vi "OxygenExtractor_elife34.vi"(14 "Image_array":T3[](array[typedef])=["IMAGE0", "Image1"]) -> (19 "Local error":errorcluster caption="error in")   [LabVIEW 2013]
uses:
  <vilib>/vision/Image Controls.llb/IMAQ Image.ctl
  <vilib>/Analysis/baseanly.llb/Mean (DBL).vi
  <vilib>/Analysis/NI_AALBase.lvlib
  Phosphorescence - Mode.lvlib
  <vilib>/vision/NI_Vision_Development_Module.lvlib
  <vilib>/Analysis/NI_AALPro.lvlib
panel:
  out "Acquisition Time":timestamp=timestamp(-9593251200 s since 1904-01-01)
  in  "Point Number":i32
  in  "Save":bool
  in  "Time onglets":enum32{"Averaged", "Time-lapsed"}(tab)
  out "Average fit":dbl[][](graph)
  out "DataValues":T1(array[cluster])
  in  "Analyse Average":bool
  in  "Pulse Amplitu Analysis":enum32{"RBC Flow", "EAT", "pO2 RBC/InterRBC"}(tab)=enum."pO2 RBC/InterRBC"
  in  "Channel Analysed RBC Flow":u16(ring)=1 items=["1", "2"]
  out "RBC anal Checked":dbl[][](graph)
  out "Mean Flow":dbl format="%#_3g"
  out "Mean Hematocrit":dbl format="%#_3g"
  in  "Analyse RBCs Flow":bool
  in  "from time (s)":dbl
  in  "to time (s)":dbl max=9.984
  in  "Point Analysed":i32 max=600
  in  "Analyse EAT":bool
  in  "Channel analysed for EAT":u16(ring) items=["1", "2"]
  in  "Around RBCs Analysis":enum32{"Tau", "Po2", "Number of decays"}(tab)=enum."Number of decays"
  out "Tau / RBCs":cluster{dbl[], dbl[]}(graph) caption="Measurement"
  out "PO2 / RBCs":cluster{dbl[], dbl[]}(graph) caption="Measurement"
  out "Decays / RBCs":cluster{dbl[], i32[]}(graph) caption="Measurement"
  out "Point EAT":i32 max=600
  in  "RBC before":bool
  in  "RBC after":bool
  in  "Analyse PO2 RBC/InterRBC":bool
  out "Std pO2 (1)":dbl format="%#_3g"
  out "pO2 (1)":dbl format="%#_3g"
  out "Std pO2 (2)":dbl format="%#_3g"
  out "pO2 (2)":dbl format="%#_3g"
  out "Std Tau 1":dbl format="%#_3g"
  out "Amplitude 1":dbl format="%#_3g"
  out "Std Tau 2":dbl format="%#_3g"
  out "Amplitude 2":dbl format="%#_3g"
  out "Number of decays 2":i32
  out "Number of decays 1":i32
  out "Tau 2 (us)":dbl format="%#_3g"
  out "Tau 1 (us)":dbl format="%#_3g"
  out "Average fit 1/2":dbl[][](graph)
  in  "From time (ms) 1":dbl=-1.0 min=-10.7328
  in  "To time (ms) 1":dbl=1.0 max=38.1888
  in  "From time (ms) 2":dbl=8.0 min=-10.7328
  in  "To time (ms) 2":dbl=12.0 max=38.1888
  in  "Min":dbl=-3.0 format="%#.1f"
  in  "Max":dbl=20.0 format="%#.1f"
  in  "Channel Analysed":u16(ring) items=["1", "2"]
  out "Total number of points":i32=1
  in  "LUT":u16(ring)=7 items=["grey-progress", "gray", "gray + high", "gray + bounds", "gradient", "temperature", "cold/hot (1/2)", "cold/hot (1/4)", "odd/even"]
  in  "Display raw Data":bool=TRUE
  out "Standard error Tau (us)":dbl format="%#_3g"
  out "element 2":dbl
  out "element":dbl
  out "Tau (us)":dbl format="%#_3g"
  out "Area (au)":dbl format="%#_3g"
  out "amplitude":dbl caption="Amplitude (au)" format="%#_3g"
  out "size(s) 3":i32[](array[numeric])=[2, 40000]
  out "size(s) 2":i32[](array[numeric])=[4, 267]
  out "size(s)":i32[](array[numeric])=[8, 267]
  in  "Time":dbl[](array[numeric])
  in  "Tau":dbl[](array[numeric])
  in  "Po2":dbl[](array[numeric])
  in  "Decays":i32[](array[numeric])=[0, 0, 0, 0, 0, 0, 0, 0, 0, 0, 0, 0, 0, 0, 0, 0, 0, 0, 0, 0, 0, 0, 0, 0, 0, 0, 0, 0, 0, 0, 0, 0, 0, 0, 0, 0, 0, 0, 0, 0, 0, 0, 0, 0, 0, 0, 0, 0, 0, 0, 0, 0, 0, 0, 0, 0, 0, 0, 0, 0, 0, 0, 0, 0, 0, 0, 0, 0, 0, 0, 0, 0, 0, 0, 0, 0, 0, 0, 0, 0, 0, 0, 0, 0, 0, 0, 0, 0, 0, 0, 0, 0, 0, 0, 0, 0, 0, 0, 0, 0, 0, 0, 0, 0, 0, 0, 0, 0, 0, 0, 0, 0, 0, 0, 0, 0, 0, 0, 0, 0, 0, 0, 0, 0, 0, 0, 0, 0, 0, 0, 0, 0, 0, 0, 0, 0, 0, 0, 0, 0, 0, 0, 0, 0, 0, 0, 0, 0, 0, 0, 0, 0, 0, 0, 0, 0, 0, 0, 0, 0, 0, 0, 0, 0, 0, 0, 0, 0, 0, 0, 0, 0, 0, 0, 0, 0, 0, 0, 0, 0, 0, 0, 0, 0, 0, 0, 0, 0, 0, 0, 0, 0, 0, 0, 0, 0, 0, 0, 0, 0, 0, 0, 0, 0, 0, 0, 0, 0, 0, 0, 0, 0, 0, 0, 0, 0, 0, 0, 0, 0, 0, 0, 0, 0, 0]
  out "Decays Max":i32=20000
  out "BA":bool
  out "RBC_before":i32[](array[numeric])
  out "RBC_after":i32[](array[numeric])
  out "Cells detect":u8[](array[numeric])
  out "Average fit 2":dbl[][](graph)=[[234.9197268868795, 232.23934305222366, 229.69994463923234, 227.888171249308, 226.6098911238236, 223.73740542535523, 221.40745525004613, 219.90182690533308, 217.30485329396566, 217.11736482745894, 216.68702712677614, 215.40763978593836, 215.2103709171434, 214.11810297102787, 212.40228824506366, 210.0345082118472, 208.90514855139324, 208.88060527772652, 208.52112935966045, 207.90090422587193, 207.060712308544, 206.41409854216644, 207.19985237128623, 206.4203727625023, 204.68186012179368, 203.77246724487912, 202.63627975641262, 201.80531463369624, 201.31887802177525, 201.88134342129544, 201.80715999261855, 201.11422771729102, 200.49898505259273, 199.00756597158147, 197.83299501753092, 198.52112935966045, 199.2378667650858, 198.64772098173094, 198.0005536076767, 197.43329027495847, 197.48902011441226, 197.4725964200037, 197.0042443255213, 197.83078058682415, 197.77966414467613, 198.14965860859937, 198.19154825613583, 197.06551024174203, 196.30872854770251, 195.9422402657317, 195.32349141908102, 196.50433659346743, 196.7776342498616, 196.0428123269976, 196.01107215353386, 196.26960693854954, 195.3941686658055, 194.80162391585162, 194.9665990035062, 195.37386971766009, 195.15630190071968, 194.81823214615244, 194.5357076951467, 193.93854954788708, 193.71858276434767, 193.5956818601218, 194.29027495847942, 194.8739619856062, 194.54456541797379, 194.27495847942424, 194.0310020298948, 193.6194869902196, 193.30540690164236, 192.56966229931723, 192.14965860859937, 193.18988743310575, 193.57446023251524, 193.7158147259642, 193.98523712862152, 194.10075659715815, 193.94777634249863, 193.32884295995572, 193.38125115334933, 193.38734083779295, 193.57556744786862, 193.61192101863813, 193.41169957556744, 192.5100572061266, 192.1064772098173, 192.0363535707695, 191.87027126776158, 192.7449713969367, 193.06809374423327, 192.66248385310942, 192.8745155932829, 192.62059420557298, 192.75770437350064, 192.75899612474626, 192.55729839453772, 193.15925447499538, 193.2967337147075, 193.37479239712124, 193.3400996493818, 192.9815464107769, 192.63388078981362, 192.15501014947407, 192.01974534046872, 192.24801623915852, 192.51577781878575, 192.4493448975826, 192.21184720428124, 192.29839453773758, 192.13452666543643, 192.4899427938734, 192.4096696807529, 192.51097988558774, 192.4880974349511, 192.27514301531647, 192.53607676693116, 192.73150027680384, 192.39084701974534, 192.19265547148922, 192.27440487174755, 192.38678723011625, 192.49086547333457, 192.3098357630559, 192.0819339361506, 191.84406717106478, 191.68794980623733, 191.9007196899797, 192.50931906255767, 192.63332718213692, 192.58184166820448, 192.7067724672449, 192.61985606200406, 191.94390108876178, 192.1225318324414, 191.83262594574646, 191.80697545672632, 192.260380143938, 192.4270160546226, 192.17457095405055, 191.94611551946855, 191.8180476102602, 191.9922494925263, 191.99372577966415, 191.9245248200775, 192.31241926554713, 192.28510795349695, 192.29507289167742, 192.155748293043, 191.37183982284554, 191.57316848126962, 191.7805868241373, 191.67023436058312, 192.65731684812695, 192.9660453958295, 192.74589407639786, 192.6015870086732, 192.0226979147444, 191.5517623177708, 191.25004613397306, 191.38125115334933, 191.8900166082303, 192.3965676324045, 192.22144307067725, 191.96272374976934, 191.21147813249678, 191.03598449898504, 191.27385126407086, 191.3098357630559, 191.8317032662853, 192.10131020483485, 192.72393430522237, 193.18693485883003, 192.75456726333272, 192.1961616534416, 192.45137479239713, 192.3436058313342, 192.58294888355786, 192.28289352279018, 192.12862151688503, 192.365011994833, 191.81472596420005, 191.3781140431814, 191.20760287875993, 191.21369256320355, 191.57981177338993, 191.9007196899797, 192.23399151134896, 192.3393615058129, 192.0219597711755, 191.6170880236206, 191.19468536630376, 191.197268868795, 191.3513563388079, 191.62391585163314, 191.79590330319246, 192.00073814356892, 191.77929507289167, 192.0658793135265, 192.2967337147075, 192.2199667835394, 192.44952943347482, 192.5238973980439, 192.2502306698653, 192.15740911607307, 191.81195792581656, 191.43513563388078, 191.23731315740912, 191.18305960509318, 191.61431998523713, 192.27016054622624, 192.17401734637386, 192.09909577412807, 191.96438457279942, 192.07215353386235, 191.81306514116997, 191.51743864181583, 191.63775604355047, 191.8167558590146, 191.86934858830043, 192.27606569477763, 191.9911422771729, 191.9119763794058, 191.67613950913452, 191.75179922494925, 192.06329581103526, 192.0856246539952, 192.32939656763241, 192.3816202251338, 191.96622993172173, 191.66340653257058, 191.47093559697362, 191.5458571692194, 191.7211662668389, 191.88503413914006, 192.316294519284, 192.32607492157226, 191.97342683151874, 191.92710832256873, 191.8597527219044, 191.78150950359844, 192.44270160546228, 192.78759918804207, 192.5065510241742, 192.47536445838716, 192.19173279202806, 192.2384203727625, 192.50212216276066, 192.82026204096698, 192.72282708986899, 192.4179737959033, 192.07233806975458, 192.0219597711755, 191.6997601033401, 191.66377560435504, 191.5322015131943, 191.57852002214432, 191.4043181398782, 191.9815464107769, 192.11016792766193, 192.05572983945376, 191.9719505443809, 192.1956080457649, 191.72208894630006, 191.44860675401367], [231.0665661286319, 229.30635283621848, 227.6254158206747, 226.02018464647355, 224.4872496829386, 223.02335486193417, 221.62539076173397, 220.29038800237745, 219.01551093848562, 217.79805163613858, 216.63542412102234, 215.5251588856263, 214.46489764382545, 213.4523883217047, 212.485480273986, 211.5621197158976, 210.68034536078187, 209.83828425417641, 209.0341477955191, 208.26622793902712, 207.53289356568047, 206.8325870186035, 206.1638207944857, 205.5251743840136, 204.91529125460332, 204.33287596902403, 203.77669143379282, 203.24555627149593, 202.738342311455, 202.2539721934085, 201.7914170791181, 201.34969446703982, 200.92786610541722, 200.52503599936492, 200.1403485077085, 199.7729865255391, 199.42216974862143, 199.0871530159696, 198.7672247270695, 198.46170533038642, 198.16994587994668, 197.89132665692833, 197.62525585333185, 197.3711683149361, 197.1285243408685, 196.89680853724016, 196.67552872241083, 196.46421488155846, 196.2624181683326, 196.06970995147137, 195.88568090435666, 195.70994013557393, 195.5421143586296, 195.38184709906278, 195.22879793726705, 195.0826417854136, 194.9430681969407, 194.8097807071418, 194.6824962034527, 194.560944324099, 194.4448668838279, 194.33401732550323, 194.22816019639978, 194.12707064808416, 194.03053395882003, 193.93834507748304, 193.85030818801692, 193.76623629350578, 193.68595081897848, 193.6092812321022, 193.53606468095913, 193.4661456481366, 193.3993756203968, 193.33561277322343, 193.27472166957583, 193.21657297221077, 193.16104316896028, 193.1080143103828, 193.05737375922962, 193.00901395119513, 192.962832166442, 192.91873031141688, 192.87661471049202, 192.83639590699156, 192.79798847317875, 192.76131082880104, 192.7262850678077, 192.69283679287133, 192.66089495736253, 192.6303917144416, 192.6012622729467, 192.57344475977263, 192.54688008844772, 192.52151183362983, 192.49728611125462, 192.47415146408187, 192.45205875239643, 192.43096104963172, 192.41081354269434, 192.3915734367777, 192.37319986446252, 192.35565379891156, 192.33889797097362, 192.32289679002108, 192.30761626835277, 192.29302394900162, 192.2790888367935, 192.2657813325113, 192.2530731700239, 192.24093735624686, 192.22934811380705, 192.21828082628957, 192.20771198595077, 192.19761914378586, 192.18798086184574, 192.17877666770107, 192.16998701095739, 192.16159322172848, 192.15357747098037, 192.1459227326609, 192.13861274753523, 192.1316319886501, 192.12496562835318, 192.1185995067983, 192.11252010186868, 192.1067145004551, 192.10117037102734, 192.09587593744124, 192.09081995392515, 192.0859916811932, 192.0813808636342, 192.0769777075279, 192.0727728602425, 192.06875739036897, 192.06492276874994, 192.0612608503632, 192.05776385702111, 192.0544243608492, 192.0512352685086, 192.04818980612947, 192.04528150492268, 192.0425041874397, 192.0398519544511, 192.03731917241635, 192.03490046151757, 192.0325906842325, 192.03038493442205, 192.02827852690916, 192.02626698752726, 192.02434604361676, 192.0225116149496, 192.0207598050625, 192.0190868929807, 192.01748932531424, 192.0159637087103, 192.01450680264549, 192.0131155125427, 192.01178688319806, 192.0105180925038, 192.00930644545386, 192.00814936841965, 192.00704440368324, 192.0059892042172, 192.00498152869918, 192.00401923675125, 192.0031002843936, 192.00222271970296, 192.00138467866643, 192.00058438122238, 191.99982012747947, 191.99909029410568, 191.99839333088056, 191.9977277574023, 191.99709215994312, 191.99648518844674, 191.99590555366038, 191.9953520243966, 191.99482342491794, 191.99431863243973, 191.9938365747451, 191.99337622790756, 191.99293661411613, 191.99251679959835, 191.9921158926369, 191.99173304167545, 191.99136743351008, 191.99101829156177, 191.990684874227, 191.99036647330246, 191.9900624124809, 191.98977204591446, 191.9894947568429, 191.98922995628354, 191.9889770817803, 191.98873559620884, 191.9885049866358, 191.9882847632293, 191.9880744582184, 191.98787362489952, 191.98768183668778, 191.98749868621073, 191.98732378444305, 191.98715675988038, 191.98699725775012, 191.9868449392578, 191.98669948086763, 191.98656057361512, 191.98642792245093, 191.9863012456141, 191.9861802740336, 191.9860647507567, 191.98595443040344, 191.98584907864512, 191.98574847170676, 191.9856523958917, 191.98556064712778, 191.9854730305338, 191.9853893600055, 191.98530945782056, 191.9852331542607, 191.9851602872515, 191.98509070201797, 191.9850242507559, 191.9849607923179, 191.98490019191348, 191.98484232082285, 191.9847870561235, 191.98473428042914, 191.9846838816402, 191.98463575270594, 191.98458979139687, 191.9845459000878, 191.98450398555028, 191.9844639587547, 191.9844257346812, 191.98438923213894, 191.98435437359387, 191.98432108500378, 191.98428929566126, 191.98425893804338, 191.98422994766827, 191.98420226295823, 191.98417582510885, 191.98415057796421, 191.98412646789745, 191.98410344369702, 191.9840814564578, 191.98406045947723, 191.98404040815618, 191.98402125990413, 191.98400297404876, 191.9839855117496, 191.9839688359154, 191.9839529111254, 191.98393770355423, 191.98392318089984, 191.983909312315, 191.98389606834186, 191.98388342084922, 191.98387134297283, 191.9838598090584, 191.98384879460704, 191.98383827622322, 191.98382823156513, 191.98381863929714, 191.9838094790446, 191.9838007313504], [236.6262185575532, 233.9168654267263, 231.36638716432952, 229.46511580591297, 228.15291172316577, 225.1913434645764, 222.78412271875396, 221.28731431960676, 218.61083027480655, 218.4686786585376, 218.04278191224296, 216.7151395278533, 216.50897751453505, 215.3766704202868, 213.57554136949977, 211.14940322093548, 209.99719303386448, 210.0026506034353, 209.65871406989817, 208.9722796281753, 208.08140571853608, 207.42169950673673, 208.27859090179476, 207.48003577290848, 205.6633865926187, 204.714343472552, 203.5470226995514, 202.67316481630306, 202.13477026192092, 202.77149163417295, 202.71059837215444, 201.95886807614508, 201.3224431923964, 199.77566249561448, 198.53191792742783, 199.2718649691466, 200.04232982514614, 199.40944527949063, 198.7032124682996, 198.12294829909882, 198.20004100442614, 198.20164503633788, 197.72141526161138, 198.5664660081357, 198.4960658223256, 198.8706788474995, 198.92534620366226, 197.74133892340302, 196.9423412470641, 196.58368168961104, 195.95449446246917, 197.21293843230475, 197.46421057179646, 196.65068380980603, 196.61716211822178, 196.9666860652067, 196.03944833327645, 195.4070417087573, 195.58770501118283, 195.98679385779226, 195.7430317492035, 195.38010784654531, 195.0896810578094, 194.4745984760779, 194.24584194489236, 194.10329643363303, 194.8645426022806, 195.48250800147278, 195.08363970634107, 194.79025625878498, 194.52155670437855, 194.09555287606295, 193.7986510633217, 193.0230994106797, 192.55827756553458, 193.67237972143687, 194.09113056832376, 194.2298868891572, 194.5093647013314, 194.65130906315983, 194.500986700652, 193.8390888732644, 193.91375562916883, 193.85239193516128, 194.05818345116845, 194.11564853481707, 193.87029649680906, 192.90838211656845, 192.48369076245245, 192.43347797668966, 192.26937235389326, 193.20909811622698, 193.55501707016458, 193.0818327938614, 193.3359588247288, 193.05102906711207, 193.2131130414731, 193.23498868084442, 192.97796078019388, 193.65707566112286, 193.77857565296242, 193.85075714213136, 193.7998935606442, 193.43763246474737, 193.07961300342564, 192.56219183817635, 192.40633279090167, 192.6557438838756, 192.96071009630424, 192.86983910754813, 192.58301392879702, 192.72232358976467, 192.5595673864358, 193.00006456350965, 192.89204828674644, 192.93840517203012, 192.90402668025402, 192.63741074357856, 192.9385288472247, 193.20201268039784, 192.83285036062748, 192.59345863020565, 192.7271801062424, 192.8126726936899, 192.90265293592046, 192.67833997628793, 192.42829987286413, 192.2236253043258, 192.0937337569141, 192.30684116453853, 192.97396366647777, 193.06864318325276, 192.97281981247735, 193.10112316735726, 193.00150675502326, 192.2868161956913, 192.53651681843158, 192.21110834954814, 192.19789461552094, 192.6675655045845, 192.83061819483606, 192.5382261153347, 192.2753559061272, 192.20670037833304, 192.43223413199865, 192.4034868780543, 192.33986236167632, 192.74258616835172, 192.6998860444645, 192.66604012162742, 192.55039798558857, 191.69009516182422, 191.92995142463693, 192.1879409395458, 192.0533872121068, 193.11174204267104, 193.4428734205042, 193.16702597052407, 192.98498282268358, 192.3760662825357, 191.89777504970516, 191.56539752125886, 191.7357966323987, 192.26174640072034, 192.79962937096, 192.6154466160675, 192.34773994434124, 191.51676105471378, 191.3334189201643, 191.6425762166577, 191.6891998544663, 192.21471819155488, 192.49829513682275, 193.1637195763447, 193.70628868324854, 193.2388024397523, 192.62168783580142, 192.91511572695617, 192.81157867410158, 193.0209730150035, 192.66409605257547, 192.48505188099244, 192.76945573631676, 192.19076637487535, 191.72190873129034, 191.53737907418176, 191.54632702124437, 191.90606790289795, 192.26808206211322, 192.61122094039158, 192.71358177360997, 192.39200510031483, 191.97307514421945, 191.52313611446277, 191.5558725885915, 191.67719264542183, 191.95903819098956, 192.1351316877156, 192.3616659128391, 192.17074063700505, 192.51001674289498, 192.7717659802508, 192.67823520189958, 192.86976441736704, 192.95685272466903, 192.66701880863178, 192.5388443468772, 192.17184083272565, 191.76728998519033, 191.55221298231538, 191.5002306077201, 191.9531942097333, 192.66416098950762, 192.58783326886504, 192.47539843107737, 192.35136043633761, 192.5586917415031, 192.2631972316567, 191.88557045378099, 191.95385767343785, 192.18437938020332, 192.26573741924986, 192.76795285706407, 192.42167268350977, 192.32242755628437, 192.04017071981698, 192.12847053094276, 192.4220511126696, 192.4307031345332, 192.70072410054323, 192.77835860919137, 192.36913601693948, 192.04266950261172, 191.80830163873244, 191.93012556558148, 192.11456068010742, 192.24636990050462, 192.6982147146858, 192.69319231684014, 192.34285608143048, 192.31761436012863, 192.2612560681386, 192.1535080166765, 192.86668481388574, 193.22866685964823, 192.887897136364, 192.86523274660993, 192.61969988551502, 192.65385825095495, 192.94155403582377, 193.2984858331657, 193.14578092683539, 192.76939168761237, 192.3936108524359, 192.3449598119352, 192.05564839660448, 192.02945811365035, 191.8840108132697, 191.98358052340132, 191.74178232915372, 192.35865110104183, 192.47754849779463, 192.40509391824074, 192.35126153405633, 192.62770728609317, 192.12215677962152, 191.81696029193262], [233.2132352162058, 230.56182067772102, 228.03350211413516, 226.311226692703, 225.0668705244814, 222.28346738613408, 220.0307877813383, 218.5163394910594, 215.99887631312478, 215.76605099638027, 215.33127234130933, 214.10014004402342, 213.91176431975174, 212.85953552176892, 211.22903512062754, 208.9196132027589, 207.813104068922, 207.75855995201772, 207.38354464942273, 206.82952882356855, 206.04001889855192, 205.40649757759616, 206.1211138407777, 205.3607097520961, 203.70033365096864, 202.83059101720625, 201.72553681327383, 200.93746445108943, 200.50298578162958, 200.99119520841793, 200.90372161308267, 200.26958735843695, 199.67552691278905, 198.23946944754846, 197.134072107634, 197.7703937501743, 198.43340370502548, 197.88599668397126, 197.2978947470538, 196.7436322508181, 196.77799922439837, 196.74354780366951, 196.28707338943124, 197.0950951655126, 197.06326246702668, 197.42863836969923, 197.4577503086094, 196.38968156008104, 195.67511584834094, 195.30079884185236, 194.69248837569288, 195.7957347546301, 196.09105792792673, 195.43494084418916, 195.40498218884593, 195.5725278118924, 194.74888899833454, 194.19620612294594, 194.34549299582955, 194.7609455775279, 194.56957205223586, 194.25635644575956, 193.981734332484, 193.40250061969627, 193.19132358380298, 193.08806728661057, 193.71600731467822, 194.26541596973962, 194.0054911296065, 193.7596607000635, 193.54044735541106, 193.14342110437624, 192.81216273996301, 192.11622518795477, 191.74103965166415, 192.70739514477464, 193.0577898967067, 193.20174256277122, 193.46110955591163, 193.55020413115648, 193.39456598434526, 192.81859704664706, 192.84874667752982, 192.92228974042462, 193.0929514445688, 193.1081935024592, 192.95310265432582, 192.11173229568473, 191.72926365718217, 191.63922916484935, 191.4711701816299, 192.28084467764643, 192.58117041830195, 192.24313491235745, 192.41307236183698, 192.1901593440339, 192.3022957055282, 192.2830035686481, 192.13663600888157, 192.6614332888679, 192.81489177645258, 192.89882765211112, 192.88030573811943, 192.52546035680643, 192.1881485762016, 191.74782846077179, 191.63315789003576, 191.84028859444143, 192.07084554126726, 192.02885068761705, 191.84068047976547, 191.8744654857105, 191.70948594443706, 191.97982102423717, 191.92729107475935, 192.08355459914537, 192.07216818964818, 191.9128752870544, 192.13362468663763, 192.26098787320984, 191.9488436788632, 191.7918523127728, 191.8216296372527, 191.9609017665426, 192.07907801074867, 191.94133154982387, 191.73556799943705, 191.46450903780377, 191.28216585556055, 191.49459821542087, 192.04467445863756, 192.1980111810211, 192.1908635239316, 192.31242176713252, 192.23820536898486, 191.60098598183225, 191.70854684645124, 191.45414354194477, 191.4160562979317, 191.85319478329149, 192.02341391440916, 191.8109157927664, 191.6168751328099, 191.42939484218738, 191.55226485305394, 191.58396468127398, 191.50918727847866, 191.88225236274255, 191.8703298625294, 191.92410566172742, 191.7610986004974, 191.05358448386687, 191.2163855379023, 191.37323270872878, 191.28708150905945, 192.20289165358287, 192.48921737115478, 192.32476218227166, 192.2181911946628, 191.66932954695312, 191.20574958583643, 190.93469474668726, 191.02670567429996, 191.51828681574025, 191.993505893849, 191.82743952528702, 191.57770755519743, 190.90619521027978, 190.7385500778058, 190.90512631148403, 190.9304716716455, 191.44868834101572, 191.70432527284694, 192.28414903410004, 192.6675810344115, 192.27033208691313, 191.7706354710818, 191.9876338578381, 191.87563298856682, 192.14492475211222, 191.90169099300488, 191.77219115277762, 191.96056825334924, 191.43868555352475, 191.03431935507245, 190.8778266833381, 190.88105810516274, 191.25355564388192, 191.53335731784617, 191.85676208230635, 191.9651412380158, 191.65191444203614, 191.26110090302174, 190.86623461814474, 190.83866514899847, 191.02552003219398, 191.28879351227673, 191.4566749186693, 191.63981037429875, 191.3878495087783, 191.621741884158, 191.8217014491642, 191.76169836517923, 192.0292944495826, 192.0909420714188, 191.8334425310988, 191.77597388526894, 191.45207501890746, 191.10298128257122, 190.92241333250286, 190.86588860246624, 191.27544576074095, 191.87616010294485, 191.76020142388268, 191.72279311717878, 191.57740870926122, 191.58561532622159, 191.36293305068324, 191.14930682985067, 191.32165441366308, 191.44913233782586, 191.472959757351, 191.78417853249118, 191.56061187083606, 191.5015252025272, 191.31210829845205, 191.37512791895574, 191.7045405094009, 191.74054617345723, 191.9580690347216, 191.9848818410762, 191.56332384650398, 191.28414356252944, 191.1335695552148, 191.16158877285733, 191.3277718535704, 191.5236983777755, 191.93437432388222, 191.95895752630437, 191.603997581607, 191.53660228500883, 191.45824937567022, 191.40951099052037, 192.0187183970388, 192.3465315164359, 192.1252049119844, 192.0854961701644, 191.7637656985411, 191.82298249457006, 192.06269028969754, 192.34203824876826, 192.2998732529026, 192.06655590419422, 191.75106528707326, 191.69895973041577, 191.34387181007574, 191.29809309505973, 191.18039221311892, 191.17345952088732, 191.06685395060268, 191.60444172051197, 191.74278735752924, 191.70636576066678, 191.59263955470544, 191.76350880543666, 191.3220211129786, 191.08025321609472]]
  out "Average fit  3":dbl[][](graph)=[[361.98715164676076, 357.74737604053564, 349.9804560260586, 339.81722765110385, 333.22982265653275, 327.76076728193993, 324.60712993123417, 319.78954035468695, 314.35522982265655, 309.4455302207745, 302.92001447701773, 299.2213174086138, 297.1279406442273, 293.2345276872964, 288.36138255519364, 284.0752804922186, 277.904632645675, 272.4963807455664, 268.9420919290626, 268.5562794064423, 265.80528411147304, 263.0919290626131, 261.20285921100253, 257.7978646398842, 254.13011219688744, 251.06170828809266, 248.2643865363735, 247.28447339847992, 245.47828447339847, 242.92001447701773, 240.62269272529858, 240.8581252262034, 239.92327180600796, 236.69905899384727, 233.0515743756786, 232.7178791169019, 233.18005790807095, 232.46073108939558, 231.76239594643502, 229.27723488961274, 226.4196525515744, 225.17643865363735, 223.99077090119437, 223.76981541802388, 224.55899384726746, 222.7792254795512, 221.2839305103149, 219.96000723850887, 219.96833152370613, 219.2757871878393, 216.91639522258416, 216.61871154542163, 216.4361201592472, 215.30365544697793, 213.71226927252985, 212.47828447339847, 211.58161418747738, 211.16322837495477, 210.09428157799493, 209.7529858849077, 209.29044516829532, 209.3346000723851, 208.7547955121245, 209.28736880202678, 208.22909880564603, 207.3825551936301, 205.70774520448788, 205.89268910604414, 205.5019905899385, 205.28646398841838, 205.2082880926529, 204.88545059717697, 203.99764748461817, 203.07908070937387, 203.4011943539631, 203.5910242490047, 203.22891784292435, 203.17734346724575, 203.31270358306188, 203.44064422728917, 202.24068041983352, 200.93213897937025, 199.82446615997105, 199.93376764386537, 199.7801302931596, 199.94553022077451, 200.42309084328627, 200.57148027506335, 199.97140788997467, 199.16847629388346, 198.45258776692, 198.62486427795875, 199.06623235613463, 198.66865725660514, 198.60351067680057, 198.60712993123417, 197.88128845457837, 197.78935939196526, 197.2616720955483, 197.10495837857403, 197.3108939558451, 197.18349619978284, 197.04524068041982, 196.42870068765833, 197.34183858125226, 197.97792254795513, 197.55971769815417, 197.13789359391964, 196.14513210278682, 195.66757148027506, 195.06279406442272, 195.01791530944627, 195.40047050307638, 195.40047050307638, 195.3720593557727, 195.30094100615273, 196.22566051393412, 196.6138255519363, 197.31921824104234, 195.9719507781397, 195.18946796959827, 194.83586681143683, 194.39974665218966, 194.0988056460369, 193.8373145132103, 194.3291711907347, 195.00941006152732, 194.63282663771264, 194.20629750271445, 194.52497285559176, 194.73163228374955, 196.42580528411148, 196.24212812160695, 195.60369163952225, 195.0866811436844, 194.33568584871517, 194.0640608034745, 193.89721317408615, 193.7303655446978, 193.44064422728917, 193.24665218964893, 193.36789721317407, 193.8346000723851, 193.57582338038364, 193.87423090843285, 193.61165399927614, 193.44607310893957, 194.20810712993122, 194.1838581252262, 193.5727470141151, 193.30962721679333, 193.1026058631922, 192.7915309446254, 192.9011943539631, 192.95674990951863, 193.45747376040535, 194.13264567499095, 194.50723850886718, 194.41838581252262, 193.50506695620703, 193.0743756786102, 193.21679334057185, 192.85088671733624, 192.98117987694536, 192.91820484980093, 193.347629388346, 193.76492942453854, 193.11093014838943, 192.55211726384366, 191.89902280130292, 191.50941006152732, 191.94100615273254, 191.8177705392689, 192.33260948244663, 192.76746290264205, 192.8460007238509, 192.40589938472675, 192.27687296416937, 192.43901556279405, 192.81505609844373, 193.07419471588852, 193.256786102063, 193.0893955845096, 192.28610206297503, 192.07853782120884, 192.0106768005791, 191.62540716612378, 192.10622511762577, 192.5727470141151, 193.05772710821572, 193.17625769091566, 192.5358306188925, 192.01719145855952, 192.1550850524792, 191.9902280130293, 192.3916033297141, 192.50470503076366, 192.9605501266739, 193.20557365182773, 192.90408975750995, 192.3564965617083, 192.066594281578, 191.96905537459284, 192.9632645674991, 193.2328990228013, 193.1539992761491, 193.00162866449512, 192.49149475208108, 192.17752442996743, 191.97068403908796, 191.8563155989866, 192.23977560622512, 192.85486789721318, 193.24846181686573, 193.08070937386898, 192.89359391965255, 192.55573651827723, 191.95204487875498, 191.83116178067317, 192.54578356858488, 192.9167571480275, 192.9534925805284, 192.54759319580165, 192.37893593919654, 192.0088671733623, 191.67734346724575, 191.38472674629026, 191.661961635903, 191.9254433586681, 192.3836409699602, 192.71425986246834, 192.42978646398842, 192.44245385450597, 192.1521896489323, 191.4755700325733, 191.8816503800217, 192.1900108577633, 192.49077090119437, 192.35251538183135, 192.28356858487152, 191.91929062613102, 191.49258052841114, 191.51972493666304, 192.19525877669201, 192.1628664495114, 192.14603691639522, 192.17046688382194, 192.2495475931958, 192.17625769091566, 192.05066956207023, 192.07238508867172, 192.352696344553, 192.40463264567498, 192.50253347810352, 192.8845457835686, 192.92309084328627, 192.17788635541078, 192.01501990589938, 192.4835323923272, 193.14332247557005, 192.74068041983352, 192.4545783568585, 192.5901194353963, 192.371335504886, 191.93811074918565, 191.90644227289178, 191.65924719507782], [350.75705096081435, 345.0654666784949, 339.5784851222621, 334.2887511738493, 329.18917411891886, 324.2729181421932, 319.5333931642692, 314.9642460078337, 310.5593518814381, 306.31280616941694, 302.2189165169451, 298.2721951996231, 294.46735176736337, 290.79928595271565, 287.2630808341264, 283.85399624496745, 280.56746241949816, 277.39907386724497, 274.3445834675865, 271.39989677662777, 268.56106653873314, 265.82428739535976, 263.1858907840998, 260.64234002109316, 258.1902255602191, 255.82626042271187, 253.5472757910737, 251.35021676137936, 249.2321382482778, 247.19020103720223, 245.22166797849627, 243.32390031835507, 241.49435416166247, 239.73057706198333, 238.03020473413983, 236.39095788496488, 234.8106391579847, 233.28713018793468, 231.8183887611605, 230.4024460780978, 229.03740411416123, 227.721433075505, 226.45276894624422, 225.2297111238498, 224.05062013954665, 222.91391546065978, 221.8180733719621, 220.7616249331845, 219.7431540099495, 218.76129537548996, 217.81473288060727, 216.90219768941682, 216.02246657851518, 215.17436029728935, 214.3567419871701, 213.56851565771052, 212.80862471744683, 212.07605055757233, 211.36981118652574, 210.6889599136638, 210.03258408025377, 209.3998038360842, 208.78977096005482, 208.20166772316406, 207.6347057923701, 207.0881251738565, 206.56119319428538, 206.053203518673, 205.56347520357093, 205.09135178428375, 204.63620039489965, 204.19741091995462, 203.77439517659272, 203.3665861261262, 202.97343711393893, 202.59442113671378, 202.229030136002, 201.87677431718774, 201.53718149293428, 201.20979645023255, 200.894180340203, 200.58991008983324, 200.29657783486243, 200.01379037305273, 199.7411686371147, 199.47834718657992, 199.22497371794017, 198.98070859239618, 198.74522438058293, 198.51820542366139, 198.29934741018815, 198.08835696819617, 197.88495127193903, 197.68885766277248, 197.49981328366445, 197.31756472684393, 197.14186769411603, 196.97248666938845, 196.80919460296974, 196.65177260721686, 196.50000966312328, 196.35370233745513, 196.21265451005556, 196.07667711095203, 195.94558786691445, 195.8192110571237, 195.69737727762376, 195.5799232142413, 195.4666914236683, 195.35753012241454, 195.2522929833469, 195.15083893954252, 195.05303199519327, 194.95874104330787, 194.8678396899673, 194.78020608489786, 194.69572275813485, 194.61427646255814, 194.5357580220878, 194.46006218533756, 194.38708748452845, 194.3167360994747, 194.24891372645908, 194.18352945182176, 194.12049563009356, 194.05972776651018, 194.00114440374955, 193.94466701274118, 193.8902198874004, 193.8377300431469, 193.78712711907122, 193.73834328361835, 193.69131314366177, 193.64597365684605, 193.6022640470807, 193.56012572307174, 193.5195021997821, 193.48033902271524, 193.44258369492067, 193.40618560662355, 193.37109596738398, 193.33726774069484, 193.3046555809312, 193.27321577256575, 193.24290617156964, 193.2136861489199, 193.18551653613736, 193.1583595727829, 193.1321788558405, 193.10693929092037, 193.0826070452161, 193.05914950215274, 193.03653521766557, 193.01473387805018, 192.993716259328, 192.97345418807262, 192.95392050364404, 192.93508902178095, 192.9169344995014, 192.8994326012655, 192.88255986635446, 192.8662936774222, 192.85061223017757, 192.83549450415643, 192.82092023454442, 192.80686988501253, 192.79332462152948, 192.78026628711515, 192.76767737750185, 192.7555410176704, 192.74384093922973, 192.73256145860955, 192.72168745603716, 192.7112043552699, 192.701098104056, 192.6913551552982, 192.6819624488942, 192.67290739423012, 192.66417785330302, 192.65576212445046, 192.6476489266648, 192.63982738447132, 192.63228701334998, 192.6250177056814, 192.61800971719776, 192.61125365392107, 192.60474045957076, 192.59846140342407, 192.5924080686128, 192.58657234084077, 192.5809463975069, 192.5755226972192, 192.5702939696859, 192.56525320596975, 192.5603936490928, 192.55570878497895, 192.55119233372193, 192.54683824116745, 192.54264067079768, 192.5385939959076, 192.53469279206269, 192.53093182982752, 192.52730606775592, 192.52381064563312, 192.52044087796077, 192.51719224767618, 192.51406040009726, 192.51104113708544, 192.5081304114179, 192.50532432136274, 192.50261910544847, 192.50001113742218, 192.49749692138852, 192.49507308712361, 192.49273638555738, 192.49048368441822, 192.48831196403438, 192.48621831328614, 192.4841999257035, 192.48225409570438, 192.48037821496763, 192.47856976893684, 192.4768263334496, 192.475145571488, 192.47352523004594, 192.471963137109, 192.47045719874296, 192.46900539628706, 192.4676057836478, 192.46625648469052, 192.4649556907243, 192.4637016580777, 192.46249270576118, 192.4613272132139, 192.4602036181315, 192.45912041437168, 192.45807614993547, 192.45706942502073, 192.45609889014585, 192.45516324434075, 192.454261233403, 192.4533916482166, 192.45255332313124, 192.45174513439972, 192.45096599867162, 192.45021487154116, 192.4494907461471, 192.44879265182317, 192.4481196527969, 192.44747084693523, 192.44684536453528, 192.44624236715842, 192.44566104650653, 192.44510062333842, 192.44456034642525, 192.44403949154358, 192.4435373605046, 192.44305328021812, 192.4425866017905, 192.44213669965467, 192.44170297073157, 192.44128483362184, 192.44088172782648, 192.44049311299543, 192.44011846820328, 192.439757291251, 192.43940909799278], [365.25570048647614, 360.9663185287028, 353.1168188169238, 342.80036533045757, 336.15022351613686, 330.63089566292956, 327.4778222209384, 322.6706033882907, 317.1528636098707, 312.21577067293975, 305.6181598375633, 301.88915296850456, 299.7438890811282, 295.81082213317205, 290.8625686002171, 286.5097095691867, 280.21951425160745, 274.74874032103213, 271.1291203250122, 270.77254842490163, 268.007196364775, 265.2248507650524, 263.2885604886723, 259.85028033659023, 256.14573976352807, 253.0154184556474, 250.1789879764434, 249.20641141731264, 247.36450433863592, 244.78458999965915, 242.42001085406397, 242.71027749594745, 241.73428301643256, 238.4056901916552, 234.66130424142887, 234.33496478409245, 234.866310165342, 234.1518046791831, 233.38799380555704, 230.81439764410095, 227.8806360951708, 226.63731916607878, 225.44219412347707, 225.1972440809539, 226.04204753459226, 224.24640916369358, 222.6777639131533, 221.32791210243698, 221.35664558029754, 220.6769468200448, 218.22691267711716, 217.89249835635127, 217.71227072175017, 216.57516531500963, 214.92777148557138, 213.7023562508207, 212.7641707332041, 212.36348166830666, 211.25962412270658, 210.87697472983314, 210.4096231156084, 210.4523063916633, 209.84067777182509, 210.43425025224832, 209.34373592391154, 208.43813681330226, 206.73114952285852, 206.93572729896462, 206.51530943523562, 206.26495433341225, 206.2102675420696, 205.88237156179878, 204.962485376975, 203.97265077962686, 204.32338943088251, 204.55547110906448, 204.13334228726367, 204.09561836348593, 204.21225938247156, 204.41224122026244, 203.1506991774739, 201.7723437231445, 200.61331593156902, 200.72879514120459, 200.56028230612537, 200.73707921605174, 201.28109132539097, 201.43682617224212, 200.81900806034346, 199.94427329907975, 199.18143630964315, 199.34842835757675, 199.83879118286657, 199.4069939942787, 199.35942257908906, 199.38443832065994, 198.65724985541203, 198.59844695481172, 197.99621125447538, 197.77279857841202, 198.00458281787013, 197.87228054027526, 197.73044901117427, 197.09110511878183, 198.0902869935195, 198.78383866886884, 198.30190492027313, 197.82199814427568, 196.7485055525714, 196.25753505207874, 195.58164360682846, 195.5972086456585, 196.02296413646957, 196.03654051152543, 196.00603174467705, 195.89981116788834, 196.92116374047302, 197.3619054361548, 198.08817628653028, 196.63691323091277, 195.7532544357004, 195.3985124823186, 194.93101683542727, 194.59328793212205, 194.31015174328294, 194.84492720958698, 195.6100782884604, 195.23056450494715, 194.74532639668277, 195.1057467683169, 195.3369080625557, 197.15162285037871, 196.96620676005725, 196.2161508769852, 195.6473191194192, 194.88013180717752, 194.5894246425438, 194.4292466416272, 194.27492655298255, 193.92890573001222, 193.66006115355995, 193.79762782519794, 194.3114999475609, 194.07041922008648, 194.4209471618432, 194.14337601669712, 193.93500208147066, 194.7655581070133, 194.71310349669426, 194.03890769663695, 193.7357644656997, 193.539331370242, 193.22325580910336, 193.38665754173903, 193.4755755132856, 193.93876008345958, 194.6744958036813, 195.07288158255466, 194.97493561692835, 193.98770737103484, 193.5574805482085, 193.74124179988897, 193.3278915153728, 193.4226488139067, 193.32907452362184, 193.79798678784238, 194.28823130304207, 193.6022797957139, 193.00122125875484, 192.29900100293384, 191.85669157542844, 192.32416858620286, 192.1399293956919, 192.72368791366182, 193.2035220179836, 193.31899587615004, 192.87690800006376, 192.7010624912482, 192.9369584537053, 193.33011590194096, 193.57022226981778, 193.73134277308566, 193.52473404408175, 192.64458189166066, 192.4351828844709, 192.42987405962523, 191.994103716551, 192.48034796861896, 192.98019221769152, 193.53626887197356, 193.66044733056816, 192.97795741340556, 192.403528576285, 192.60778159712524, 192.41617718442674, 192.80196919313602, 192.93596024546457, 193.42940345950853, 193.6738394589513, 193.3699704441271, 192.76715379919517, 192.45494287502288, 192.3507863473849, 193.45098181599795, 193.71523543508346, 193.60212216941034, 193.39678441709418, 192.88531416990034, 192.56164306814932, 192.35987941863158, 192.24534857936146, 192.63729906984597, 193.3066929159672, 193.76142834615214, 193.55715806817912, 193.34959791154495, 192.9798591055439, 192.31038992192066, 192.19138195235107, 192.96633594701427, 193.36737982289037, 193.4229157770797, 192.94968157155427, 192.81637163212196, 192.423755088423, 192.05073712984833, 191.73183938370002, 192.01706244477162, 192.28222674034433, 192.77114536129224, 193.1550400998317, 192.8519792906563, 192.874824401097, 192.58607738983903, 191.81923325909324, 192.22729744952747, 192.5821635678914, 192.91650981031688, 192.73306528363287, 192.67249383504273, 192.31178462772624, 191.84832531114282, 191.89232684442578, 192.62039618664386, 192.55702882310072, 192.52634070620832, 192.55277715238435, 192.66775697972045, 192.6114863292112, 192.4599899503847, 192.5068110085425, 192.78701379815723, 192.8150056380759, 192.91290248941928, 193.3010912441786, 193.4034118717372, 192.59216864780015, 192.43270969132632, 192.9747909566735, 193.63108829884337, 193.17298469670257, 192.8214244802668, 192.98547443077652, 192.78245724116846, 192.31170130125676, 192.29825363067582, 192.0460791027105], [358.7186028070454, 354.5284335523685, 346.84409323519344, 336.83408997175013, 330.30942179692863, 324.8906389009503, 321.73643764152996, 316.9084773210832, 311.55759603544243, 306.6752897686093, 300.22186911647213, 296.55348184872304, 294.5119922073264, 290.65823324142076, 285.86019651017017, 281.6408514152505, 275.58975103974257, 270.24402117010067, 266.755063533113, 266.34001038798294, 263.6033718581711, 260.95900736017376, 259.11715793333275, 255.74544894317822, 252.1144846302468, 249.10799812053793, 246.3497850963036, 245.3625353796472, 243.59206460816102, 241.0554389543763, 238.82537459653318, 239.00597295645937, 238.11226059558336, 234.99242779603935, 231.44184450992833, 231.10079344971138, 231.4938056507999, 230.76965749960806, 230.136798087313, 227.74007213512454, 224.958669007978, 223.7155581411959, 222.53934767891167, 222.34238675509386, 223.07594015994266, 221.31204179540882, 219.89009710747646, 218.59210237458075, 218.58001746711471, 217.87462755563382, 215.60587776805116, 215.344924734492, 215.15996959674422, 214.03214557894623, 212.49676705948832, 211.25421269597624, 210.39905764175066, 209.96297508160288, 208.92893903328329, 208.62899703998227, 208.17126722098223, 208.21689375310686, 207.66891325242392, 208.14048735180523, 207.11446168738053, 206.32697357395796, 204.68434088611724, 204.84965091312367, 204.48867174464135, 204.3079736434245, 204.2063086432362, 203.88852963255516, 203.03280959226134, 202.18551063912088, 202.47899927704367, 202.62657738894492, 202.32449339858502, 202.25906857100557, 202.4131477836522, 202.4690472343159, 201.33066166219314, 200.091934235596, 199.03561638837309, 199.13874014652615, 198.99997828019383, 199.1539812254973, 199.56509036118157, 199.70613437788458, 199.12380771960588, 198.39267928868716, 197.72373922419686, 197.90130019834075, 198.2936735294027, 197.93032051893158, 197.84759877451208, 197.8298215418084, 197.1053270537447, 196.9802718291188, 196.52713293662123, 196.43711817873603, 196.61720509382008, 196.49471185929042, 196.36003234966537, 195.76629625653484, 196.59339016898502, 197.17200642704142, 196.81753047603522, 196.4537890435636, 195.54175865300223, 195.07760790847138, 194.54394452201697, 194.43862197323404, 194.7779768696832, 194.76440049462732, 194.73808696686837, 194.7020708444171, 195.5301572873952, 195.86574566771776, 196.5502601955544, 195.30698832536663, 194.62568150349614, 194.27322114055505, 193.86847646895205, 193.60432335995176, 193.36447728313763, 193.81341517188244, 194.40874183459425, 194.03508877047813, 193.66726860874613, 193.94419894286662, 194.1263565049434, 195.69998771784424, 195.51804948315666, 194.9912324020593, 194.52604316794958, 193.79123989025283, 193.53869696440518, 193.3651797065451, 193.18580453641306, 192.95238272456612, 192.8332432257379, 192.93816660115021, 193.35770019720928, 193.0812275406808, 193.3275146550225, 193.07993198185517, 192.9571441364085, 193.65065615284914, 193.65461275375816, 193.10658633159323, 192.88348996788696, 192.6658803561424, 192.35980608014745, 192.41573116618716, 192.43792430575166, 192.97618743735111, 193.5907955463006, 193.9415954351797, 193.86183600811688, 193.02242654137922, 192.59127080901192, 192.69234488125474, 192.37388191929966, 192.53971093998402, 192.50733517598002, 192.89727198884964, 193.241627546035, 192.61958050106495, 192.10301326893247, 191.499044599672, 191.1621285476262, 191.55784371926222, 191.49561168284592, 191.94153105123144, 192.3314037873005, 192.37300557155174, 191.93489076938974, 191.85268343709055, 191.9410726718828, 192.2999962949465, 192.57816716195927, 192.78222943104032, 192.65405712493742, 191.9276222342894, 191.7218927579468, 191.59147954153295, 191.25671061569656, 191.73210226663258, 192.16530181053866, 192.57918534445787, 192.69206805126316, 192.09370382437945, 191.63085434083405, 191.70238850783315, 191.56427884163188, 191.98123746629216, 192.07344981606275, 192.49169679383925, 192.73730784470416, 192.4382090708928, 191.94583932422142, 191.67824568813313, 191.58732440180077, 192.47554731900024, 192.75056261051913, 192.70587638288788, 192.60647291189605, 192.09767533426182, 191.79340579178555, 191.58148865954433, 191.46728261861176, 191.84225214260428, 192.40304287845916, 192.7354952875793, 192.60426067955885, 192.43758992776014, 192.13161393101055, 191.5936998355893, 191.47094160899528, 192.1252311901555, 192.46613447316463, 192.4840693839771, 192.14550482004904, 191.94150024627112, 191.59397925830157, 191.30394980464317, 191.0376141088805, 191.30686082703437, 191.56865997699188, 191.99613657862815, 192.27347962510498, 192.00759363732055, 192.01008330791495, 191.71830190802558, 191.13190680605337, 191.53600331051595, 191.7978581476352, 192.06503199207185, 191.97196548002984, 191.8946433347003, 191.5267966245358, 191.13683574567946, 191.1471230289003, 191.77012136674017, 191.76870407592207, 191.76573312658212, 191.78815661525954, 191.83133820667118, 191.74102905262012, 191.64134917375574, 191.63795916880093, 191.9183788909488, 191.99425965327407, 192.09216446678775, 192.4680003229586, 192.44276981483534, 191.7636040630214, 191.59733012047244, 191.99227382798088, 192.65555665229672, 192.30837614296448, 192.08773223345017, 192.1947644400161, 191.96021376860352, 191.56452019711455, 191.51463091510774, 191.27241528744514]]
  in  "data type":waveform(i16)[](array[waveform])
  out "N samples/decay min":i32=312
  in  "Acquisition properties":T2
  out "TmpDataPicture":T3
  in  "Conversion Policy (Full Dynamic)":T4 {"Conversion Method" items=["Full Dynamic", "Downshift", "Given Range", "90 % Dynamic", "Given Percent Range"]}
  out "Std / RBCs":dbl[][](array[numeric])
  out "Average / RBCs":dbl[][](array[numeric])
  out "Error PO2 around RBCs":dbl[](array[numeric])=[0.0, 0.0, 161.2040836868454, 38.73219150764863, 52.06123314905531, 6.087160624580337e-38, 60.47946338434948, 39.16434541629099, 32.485481230904, 28.270798219450068, 26.524399919792735, 25.53003502797235, 14.686097914670983, 15.041296822114678, 12.716397973751537, 10.654989523366996, 14.840602984999663, 14.594225661502515, 9.992995683945168, 9.781709150383362, 6.649256981373154, 4.747291645345802, 3.604424626341186, 3.8913018687881737, 2.9714025655174785, 3.0113546041649903, 2.3209689027815488, 2.098876087788983, 2.2812018175936504, 1.960349947295764, 1.9401110060900029, 1.782805684716071, 1.6941962801095243, 1.98518458325514, 1.7287816678511916, 1.7526642008773734, 1.8897383911909105, 1.878540076894968, 1.733168757087298, 1.8868589103363567, 1.776194555784892, 1.9813611382762704, 1.8686822217652008, 1.688803172744231, 1.795086387016551, 1.7722543662647712, 1.856920213450666, 1.7573820115627203, 1.8535099843963962, 1.967673257541561, 2.1607253001388567, 2.104453631230401, 1.7969389376694542, 2.11117037623537, 2.0178463798184643, 1.891767885225448, 2.1041179278743893, 1.8645920574866277, 2.1640278119963963, 1.8645815043158054, 2.302597415982519, 1.964011069218976, 2.0017134436441655, 2.3081010926050203, 1.9479715651397123, 1.7915270967536567, 1.9848376130851482, 2.1862229031068496, 2.191385105908004, 2.28685039508108, 2.3344353267703584, 2.4393757877156514, 2.190311209257636, 2.2540297938527822, 2.469830590583495, 2.499078935808259, 2.660235474457339, 2.316177567674948, 2.6831805912749602, 2.314170727077041, 2.3932789462729733, 2.2675374090515223, 2.2734619546061055, 2.879249477545812, 2.320399820608915, 2.587167839888272, 2.795265880061753, 2.48732110376029, 3.363501846656955, 2.995599257684123, 2.53449024944146, 3.2142951886004782, 2.630813026520676, 2.8984290827620196, 3.220952821168442, 3.6451853566529255, 2.8991411036864863, 2.766774860402428, 2.865777546922853, 2.9579232541115785, 3.302487033344295, 3.5524546046268948, 3.2277469064864643, 2.984152533471737, 3.112617935129897, 3.300209620876161, 3.3919816548160893, 3.8971209181836213, 3.106431410711107, 3.878065370504629, 4.694009237609732, 4.426377842153757, 3.858214995127652, 3.851170395395452, 4.703553259332945, 5.017442966095774, 3.9303241113716934, 3.6911383287194894, 6.103545230349116, 3.8723424578866914, 4.355249867188351, 5.035319735328459, 5.352974557207512, 5.381207341355095, 5.839822414617204, 5.1663220615076995, 5.514825646946649, 5.292333793666374, 6.0068390689593825, 5.587767428713819, 6.5025270001052675, 4.9275930895263755, 5.994295409034131, 5.520881874751722, 6.990114690130615, 6.851835399436859, 7.815130015429131, 6.782332242810148, 6.210935142445731, 8.665159733182241, 7.145520287106814, 6.58629211255175, 6.47603891527165, 6.493891009729253, 7.799906973202586, 7.443532821101292, 7.0519298161835255, 7.112833235973139, 6.304563757763698, 7.5660448065711785, 6.901420464745087, 7.145444324647901, 10.275972231576638, 6.9077585064344795, 9.67353910377255, 8.680129498346265, 8.728268583156048, 6.99792809499278, 12.173991377802801, 9.08536112440855, 8.155783389934925, 11.113989677720808, 5.195385223698934, 7.779333933443114, 12.092975573883283, 9.214654261618524, 10.56115665492472, 12.718066296441274, 11.307261793405148, 10.527066108349509, 13.642696146897466, 15.275701379527831, 10.982648577182445, 10.492480395102408, 13.613241802935923, 10.606524220518557, 11.74941434951697, 10.405448033941093, 9.604134535909845, 16.038283075257908, 10.878289513755787, 8.014107382493725, 10.666506779265509, 13.749063316957146, 12.116265510980329, 12.059869783566473, 13.3011232683534, 9.704449291281088, 12.736354165477488, 18.71913872084713, 17.636106608975926, 12.894073435051938, 18.07502192264925, 10.722718443521362, 10.22034069250413, 22.60323761516492, 12.619111573455319, 15.666238232852974, 12.454325572254342, 20.419708837113514, 16.772124427268643, 20.697556298460356, 20.362973833463982, 27.299358978389765, 15.794925105879734, 15.517439812732434, 12.545977071653782, 17.80312822515806, 16.6987404554246, 29.707674645701623, 44.36628564675225, 84.72568788219994, 0.0, 0.0, 0.0, 0.0, 0.0, 0.0, 0.0, 0.0, 0.0, 0.0, 0.0, 0.0, 0.0]
  out "Error Tau around RBCs":dbl[](array[numeric])=[0.0, 0.0, 2.6576160295760656, 0.6512933230021577, 1.2866105004716557, 8650172.95719788, 2.0747757813806973, 1.906895593328938, 1.661024964368098, 1.87932063312799, 2.3798249604109425, 1.254878911900616, 1.3118739695535155, 0.9466496893792453, 0.9788629761834915, 1.0365250945720552, 0.9692871034651528, 0.8696852239229983, 0.8315092537330896, 0.8644916384510862, 0.5753481503128666, 0.5856911072918298, 0.5469623015609284, 0.4999620181045545, 0.4605749198761034, 0.36824829240140605, 0.36112317232920266, 0.3824884010867234, 0.3689895335867095, 0.35592806540491445, 0.3597988334012117, 0.3498169279220879, 0.37251461482167897, 0.3243869550228511, 0.371648747420223, 0.3344545755034697, 0.3197374069595918, 0.3337359328519561, 0.34952438825353377, 0.3548705847624204, 0.37697292964180423, 0.35535575190897417, 0.36615408268974653, 0.33722150015670804, 0.3516571434974923, 0.37784274517138355, 0.38724688355965325, 0.3608845772067099, 0.34082676339717893, 0.42007747142581003, 0.38083130743739224, 0.37775378972788876, 0.39865295083089736, 0.39164972314511565, 0.37640358897214576, 0.38783678657504944, 0.4160440427685393, 0.45903294625854174, 0.4543099069005354, 0.4495543376567774, 0.35071488828930725, 0.40489190301283584, 0.4394758326899525, 0.3909599417702084, 0.43946946667145487, 0.4938361552246875, 0.42496334657689716, 0.4042272018883289, 0.4907028152271008, 0.43758399026282424, 0.4363314210702704, 0.3999381542822442, 0.4173542179004429, 0.5282563935904515, 0.4398727681991261, 0.47579005800314766, 0.4781725899364983, 0.43281323986017334, 0.4463093360693441, 0.47158066000982984, 0.445634669615095, 0.493188036244302, 0.5342839129262239, 0.4394732577702433, 0.5110306020644609, 0.5086943103846755, 0.4244421954372179, 0.469896037698148, 0.5303911022808998, 0.505371580540754, 0.48063381751284373, 0.5520847824596418, 0.4972434558489703, 0.48217034686923665, 0.6994940283949235, 0.39366486376608684, 0.5139935349320608, 0.5619464162617158, 0.5986776540639416, 0.6307757519056567, 0.45185323263332217, 0.5122632986331821, 0.6364419780823835, 0.6199428076917348, 0.6612902903105693, 0.5983747785397913, 0.5243544268284576, 0.47593793056654266, 0.4527357013933716, 0.5228034035400911, 0.5209661716352424, 0.4429824511148201, 0.5463930803288212, 0.4978439120167496, 0.5880168528708206, 0.6965383280846398, 0.5402426954357552, 0.59445543716921, 0.4173108574480802, 0.5484194986941393, 0.6367894179509829, 0.5902145906180545, 0.6362623388963498, 0.6640641836538175, 0.49481449962303337, 0.710933315984112, 0.4369069898030028, 0.5087856390107606, 0.5584575435985493, 0.7116033778319356, 0.5821455078732853, 0.8651527343944123, 0.5726452040462615, 0.3773102236499747, 0.5619000145278623, 0.586115847831369, 0.5878693324743061, 0.6381106944607859, 0.48265407962202367, 0.6029188835037391, 0.7166291677461237, 0.5233622107119065, 0.6131769506299126, 0.5823523256068754, 0.4506616770282787, 0.5596165953512222, 0.5428520254756775, 0.49537380875138876, 0.6207417556924902, 0.8058284732375991, 0.5849666462061632, 0.6591911235602361, 0.6229994207088455, 0.7086025156735122, 0.5690006173371945, 0.4278011835010632, 0.6317478583353395, 0.5436828014008961, 0.8934954875678451, 0.5466158462749693, 0.6102609186963864, 0.4184688078299235, 0.976063116045834, 0.5595160330997428, 0.670615486254349, 0.7116161436200583, 0.4771358774553331, 0.8052894749490437, 0.7233792946573152, 0.6494903504816727, 0.4803069709893352, 1.0072573027236795, 0.7986215972739006, 0.6972277596119231, 0.5827595848000051, 0.4596756485322112, 0.5637869774847095, 0.5639576990612836, 0.7342803000381696, 0.8196133263590659, 0.5845366363082696, 1.3379634863242305, 1.0489024973360253, 0.7627585475913266, 0.6966618232550706, 0.7517841394105966, 1.1913599206358338, 0.9194514605667794, 0.43446926990183715, 0.8714574584310243, 0.4298746245709736, 0.8002752680542307, 0.6659726848701372, 0.6872963368940408, 0.9331000143154946, 0.4992931998953268, 0.528252709398058, 0.8763153006918569, 0.8530907856508387, 0.8463684417648877, 0.340393048196582, 0.7784783820525997, 1.5798729175301187, 1.0861920597735435, 0.5524267616799177, 0.32174870287547624, 0.21324231450156003, 0.29328686875757376, 0.47779109664561653, 1.3464490544033443, 1.3810784600946726, 135.4563749539329, 0.0, 0.0, 0.0, 0.0, 0.0, 0.0, 0.0, 0.0, 0.0, 0.0, 0.0, 0.0, 0.0]
  out "Working file":path
  in  "Not NewlyAcquired":bool
  out "All means and fits":dbl[][][](array[numeric])=[[[349.428925, 343.6205, 338.531525, 332.91075, 327.67785, 323.45455, 318.4022, 312.48885, 307.314, 303.080025, 298.2751, 295.1001, 292.14425, 288.0041, 283.807025, 280.3876, 277.46575, 274.482675, 271.758725, 269.7288, 267.18155, 264.9167, 262.893425, 260.3201, 257.76725, 255.102775, 252.860525, 251.251925, 248.772025, 247.093675, 245.096325, 243.21415, 242.04005, 241.245375, 239.590625, 238.45325, 237.22325, 235.7478, 234.74065, 233.188475, 232.3254, 230.863175, 229.260175, 228.4722, 227.66315, 226.798025, 226.254725, 225.16775, 223.8162, 222.738925, 222.043925, 221.799, 220.8176, 219.7423, 218.7699, 218.0023, 217.273375, 216.50885, 216.164825, 216.2126, 215.3894, 214.6441, 213.988075, 213.567825, 212.6586, 212.272175, 212.23375, 211.9841, 211.35695, 211.30985, 211.15085, 210.4566, 209.727125, 209.0575, 208.621825, 208.534975, 208.329075, 207.745775, 207.58585, 206.9373, 206.533775, 205.675125, 205.4675, 205.3395, 205.18675, 205.09895, 205.015975, 204.50265, 204.134125, 203.85715, 203.373175, 203.414075, 203.199525, 203.03155, 203.2572, 202.937925, 202.75615, 202.323925, 202.156975, 202.17665, 201.895725, 202.001175, 201.95765, 201.3064, 201.104525, 200.889525, 200.4423, 200.666875, 200.660275, 200.485925, 200.6514, 200.313775, 200.05665, 199.73595, 199.298625, 199.6958, 199.9936, 199.78935, 199.4502, 198.895825, 198.588, 198.43695, 198.5303, 198.959675, 198.7242, 198.9982, 199.201475, 198.688125, 198.536125, 198.303425, 197.962325, 198.139175, 198.2954, 198.4124, 198.399225, 197.9953, 197.77015, 197.48625, 197.29135, 197.311375, 197.5119, 197.699525, 197.830325, 197.425625, 197.104875, 196.954125, 196.81285, 197.1861, 197.393875, 197.22835, 197.196175, 196.939275, 196.5688, 196.4476, 196.4522, 196.887075, 197.1458, 197.130125, 197.1908, 196.7003, 196.478775, 196.420225, 196.176825, 196.63035, 196.892775, 196.923275, 196.9035, 196.449125, 196.0815, 195.9317, 196.209825, 196.568875, 196.737025, 196.7999, 196.606925, 196.116875, 196.121, 195.833525, 195.49185, 195.69615, 195.795825, 195.9883, 196.0518, 195.7182, 195.586175, 195.494675, 195.233275, 195.66215, 195.877325, 195.87045, 195.93525, 195.68435, 195.5484, 195.34775, 195.40915, 196.21845, 196.365775, 196.1651, 195.9423, 195.558975, 195.2553, 195.32825, 195.009225, 195.38975, 195.57815, 195.63395, 195.720825, 195.48375, 195.200475, 195.0311, 195.07815, 195.510925, 195.699275, 195.615125, 195.62465, 195.34845, 195.20295, 195.0683, 195.09575, 195.39375, 195.603225, 195.9734, 196.02185, 195.582625, 195.386375, 195.379575, 195.331475, 195.392925, 195.4479, 195.59395, 195.469075, 194.997475, 194.820075, 194.72835, 195.061075, 195.395975, 195.41375, 195.452275, 195.45675, 195.2783, 195.102025, 194.8792, 194.637175, 195.20895, 195.529375, 195.515375, 195.39555, 194.988725, 194.78175, 194.861075, 194.8726, 195.1937, 195.2665, 195.2673, 195.41285, 195.156775, 194.902775, 194.774, 194.607775, 195.0283, 195.34645, 195.377175, 195.341125, 194.95315, 194.751325, 194.81975, 194.871025], [337.3160923513005, 332.77227462914755, 328.3740564690022, 324.11677235966806, 319.9959062889887, 316.0070869533835, 312.14608312088706, 308.4087991427722, 304.7912706089962, 301.2896601428618, 297.9002533304313, 294.61945478037666, 291.44378431008494, 288.36987325397496, 285.3944608901074, 282.51439098129885, 279.72660842707086, 277.0281560228815, 274.41617132320243, 271.88788360511444, 269.4406109291985, 267.0717572946075, 264.77880988529813, 262.5593364045036, 260.4109824946187, 258.3314692397608, 256.31859074835745, 254.37021181319597, 252.48426564645325, 250.65875168730304, 248.89173347977487, 247.1813366186139, 245.52574676096233, 243.92320770175346, 242.37201951077665, 240.87053672943728, 239.41716662529865, 238.01036750255432, 236.64864706663883, 235.33056084124178, 234.05471063604654, 232.8197430635674, 231.62434810351274, 230.467257713151, 229.3472444822049, 228.26312033084784, 227.21373524942084, 226.19797607853337, 225.21476532825383, 224.2630600351373, 223.3418506558781, 222.45015999641333, 221.587042175342, 220.7515816205594, 219.94289209804282, 219.1601157717587, 218.402422293693, 217.6690079230405, 216.9590946736184, 216.27192948859937, 215.60678344168917, 214.9629509639015, 214.33974909510923, 213.73651675957882, 213.15261406471905, 212.58742162230013, 212.04033989142334, 211.51078854254445, 210.99820584187552, 210.5020480555129, 210.02178887265913, 209.55691884732656, 209.1069448579306, 208.67138958420003, 208.24979100084812, 207.84170188746896, 207.44668935413796, 207.06433438221399, 206.69423137985567, 206.33598775178038, 205.98922348281, 205.65357073476085, 205.32867345625095, 205.01418700501037, 204.70977778229386, 204.41512287900846, 204.1299097331801, 203.8538357983965, 203.58660822287376, 203.32794353880743, 203.0775673616773, 202.83521409918777, 202.60062666953468, 202.37355622869995, 202.1537619064844, 201.9410105509993, 201.73507648134503, 201.53574124821495, 201.34279340217014, 201.15602826933969, 200.9752477343081, 200.80026002995982, 200.63087953405775, 200.46692657234036, 200.30822722792797, 200.15461315683646, 200.00592140940245, 199.86199425743075, 199.7226790268805, 199.58782793591277, 199.4572979381274, 199.3309505708234, 199.20865180812132, 199.09027191879233, 198.97568532864275, 198.86477048730833, 198.757409739317, 198.653489199283, 198.55289863110036, 198.45553133100745, 198.36128401439856, 198.2700567062622, 198.18175263513052, 198.09627813042655, 198.0135425231011, 197.93345804945346, 197.855939758034, 197.78090541953, 197.70827543953897, 197.63797277413713, 197.5699228481532, 197.5040534760611, 197.44029478540756, 197.37857914269324, 197.31884108162888, 197.26101723369058, 197.20504626090008, 197.15086879075903, 197.09842735326842, 197.0476663199658, 196.9985318449161, 196.9509718075935, 196.90493575759314, 196.8603748611149, 196.81724184916166, 196.7754909673977, 196.7350779276138, 196.69595986074728, 196.65809527140797, 196.62144399386077, 196.58596714941896, 196.55162710520287, 196.51838743421982, 196.48621287672333, 196.4550693028106, 196.4249236762185, 196.39574401927936, 196.36749937900015, 196.34015979422827, 196.31369626386956, 196.28808071612482, 196.2632859787119, 196.23928575004211, 196.2160545713202, 196.19356779953839, 196.17180158133561, 196.15073282769475, 196.13033918945018, 196.1105990335805, 196.0914914202608, 196.07299608065023, 196.05509339539137, 196.0377643737986, 196.02099063371318, 196.00475438200405, 195.98903839569334, 195.97382600368664, 195.9591010690888, 195.9448479720864, 195.93105159337856, 195.91769729813882, 195.90477092049102, 195.89225874848236, 195.88014750953832, 195.86842435638323, 195.85707685341242, 195.84609296350084, 195.8354610352343, 195.82516979055006, 195.8152083127733, 195.80556603503715, 195.7962327290734, 195.78719849436283, 195.77845374763294, 195.76998921269225, 195.7617959105904, 195.7538651500935, 195.74618851846478, 195.73875787254036, 195.73156533009154, 195.72460326146324, 195.7178642814809, 195.71134124161625, 195.70502722240457, 195.6989155261046, 195.6929996695937, 195.68727337749087, 195.6817305754999, 195.67636538396596, 195.67117211163853, 195.66614524963444, 195.66127946559402, 195.65656959802484, 195.65201065082638, 195.64759778799043, 195.64332632847115, 195.63919174121943, 195.63518964037667, 195.63131578062223, 195.62756605267015, 195.6239364789102, 195.62042320918837, 195.61702251672295, 195.6137307941511, 195.61054454970227, 195.6074604034943, 195.60447508394805, 195.60158542431708, 195.59878835932844, 195.59608092193096, 195.59346024014812, 195.59092353403136, 195.58846811271124, 195.58609137154303, 195.58379078934388, 195.58156392571817, 195.57940841846906, 195.57732198109258, 195.57530240035226, 195.5733475339313, 195.57145530816015, 195.56962371581673, 195.56785081399727, 195.56613472205538, 195.56447361960699, 195.5628657445994, 195.56130939144225, 195.559802909198, 195.55834469983094, 195.55693321651194, 195.55556696197755, 195.55424448694177, 195.55296438855882, 195.5517253089348, 195.5505259336875, 195.549364990552, 195.54824124803113, 195.54715351408916, 195.5461006348872, 195.54508149355945, 195.54409500902827, 195.54314013485745, 195.5422158581422, 195.54132119843482, 195.5404552067043, 195.53961696433004, 195.5388055821271], [350.6119615167477, 344.78430663105763, 339.67502629269904, 334.0255796689903, 328.76956349342873, 324.52645177586726, 319.44976479197186, 313.50859415817985, 308.31082127038906, 304.0604680429785, 299.2374358421049, 296.0504162865592, 293.07995491264523, 288.9152423267414, 284.69102064104766, 281.25997449765345, 278.3261866969298, 275.33040281672305, 272.58993017941384, 270.5450193018815, 267.9876760197636, 265.71096424225675, 263.6806960844552, 261.0950102832908, 258.52400926039, 255.83901026576598, 253.582687199089, 251.96949522755256, 249.4722533485121, 247.7815136838495, 245.7717492601228, 243.8776925700318, 242.6987556578245, 241.8981483577994, 240.2305667177976, 239.0859593194042, 237.84242175443165, 236.35659451778002, 235.33996341941375, 233.7782665892961, 232.91741809230882, 231.44376266680663, 229.82498467444728, 229.03152583028944, 228.21787903930831, 227.34014480873927, 226.78841188128374, 225.69675038539543, 224.33595383999446, 223.25400806647679, 222.55675901300017, 222.3042523032852, 221.31317266571713, 220.2248928858963, 219.2420686987717, 218.47384350527577, 217.7421596304837, 216.97159202374752, 216.62372726240775, 216.6738411544203, 215.83471209049497, 215.08046952045228, 214.4133916521192, 213.99306273497214, 213.08015018965838, 212.69310611805167, 212.6584020608374, 212.39928178991832, 211.7614315782794, 211.7141333719366, 211.55440267451343, 210.85369755780036, 210.1167288136439, 209.4413270458081, 209.0019611173537, 208.9109827401713, 208.70201375451086, 208.10855085003172, 207.94383896385835, 207.29279235992877, 206.89194940965433, 206.02145605842657, 205.8158394785891, 205.67868591471895, 205.52378582986225, 205.4327596148592, 205.35009675624312, 204.83580550396837, 204.46341732019152, 204.18518891133056, 203.69342087879548, 203.73166996874536, 203.51378010396706, 203.34037698046794, 203.57611597436318, 203.25279442220923, 203.0708547937027, 202.63225357464054, 202.4634046242145, 202.47665738510815, 202.18388708987843, 202.29222699808707, 202.24647582798625, 201.58831542255786, 201.38613602382205, 201.1765960460964, 200.72061209867297, 200.9397413570658, 200.93256619118714, 200.75035218051926, 200.92441799519634, 200.58731840013283, 200.33372265025517, 200.00853758581405, 199.5610508608688, 199.95852404069478, 200.2618806696838, 200.04980825608808, 199.70160541809793, 199.14354420961894, 198.83676909755835, 198.6880776380995, 198.7819644781207, 199.21236784214707, 198.9669041014466, 199.2465921570199, 199.45539435643155, 198.93739334481063, 198.78735227484214, 198.54845299116985, 198.20197063972637, 198.38175072041113, 198.53290459410505, 198.65613148525784, 198.63821964399855, 198.23541479170962, 198.01413376836265, 197.72066167104785, 197.51970926821443, 197.53203475622036, 197.73505255759179, 197.92524709350073, 198.06131421432582, 197.65446811046868, 197.32803018570235, 197.17618740229292, 197.03589705360514, 197.40443867996703, 197.61683587871443, 197.44771270514136, 197.4103247601195, 197.15781901944885, 196.7810338342819, 196.65668975071964, 196.66508438852813, 197.10729824315027, 197.3696508455624, 197.35005642070223, 197.4120980849081, 196.9127459684196, 196.68565364797385, 196.63148446345366, 196.38093882902194, 196.83944059692377, 197.10700812522808, 197.13311527784688, 197.11688170538676, 196.65731906882368, 196.28497405287592, 196.13018475603369, 196.42084389716737, 196.77880527153286, 196.94369134154775, 197.00775714806025, 196.80829079072944, 196.31481399093119, 196.33122383660043, 196.03746557106635, 195.68383295064783, 195.88818373565454, 195.98731361503818, 196.1822999654066, 196.24889190538678, 195.90804266108805, 195.77917020550194, 195.6904654282418, 195.418022930149, 195.8459945068106, 196.07026576978728, 196.05533936332287, 196.1221418676292, 195.87442206627207, 195.74381088489642, 195.53781624634172, 195.60457436492655, 196.43369509748177, 196.58000132504253, 196.36242794986964, 196.1258578601361, 195.74826955036727, 195.4399486746439, 195.51960581725788, 195.1921988157428, 195.57305459929697, 195.7672077287879, 195.8202553077208, 195.90638306276736, 195.67071267915932, 195.38480611408377, 195.2155541767479, 195.26053384951643, 195.69535220655072, 195.88469534607037, 195.79864185183072, 195.81030127001839, 195.53257065898464, 195.38883012005707, 195.2540226786845, 195.2892066348008, 195.58081938291298, 195.78946930827541, 196.17535451792668, 196.21868303981913, 195.77295087994736, 195.57579406512806, 195.56811040435545, 195.52166519094874, 195.5724625333283, 195.6226924079866, 195.77703243521688, 195.64556170230676, 195.1689205247757, 194.9949807068819, 194.90266175062786, 195.25152685709546, 195.584181623741, 195.58867389851997, 195.62728246929234, 195.63040041602582, 195.45616952023252, 195.28149123748628, 195.05748222761676, 194.80561253909238, 195.38360295158523, 195.7105408933898, 195.69759103686349, 195.57184136324543, 195.16144593444878, 194.9555525148651, 195.0388450498428, 195.05222804759003, 195.37258902148469, 195.44542855611596, 195.44232243789799, 195.59018989292295, 195.33768050341266, 195.07906340165331, 194.95070776539248, 194.77915713402726, 195.2021950365242, 195.52917045742043, 195.55533352940705, 195.51565647701307, 195.12773281380748, 194.9289080218337, 195.00362568898154, 195.0559134995375], [348.24588848325226, 342.45669336894235, 337.38802370730093, 331.7959203310097, 326.5861365065712, 322.3826482241327, 317.3546352080281, 311.4691058418202, 306.317178729611, 302.0995819570214, 297.3127641578951, 294.1497837134408, 291.20854508735476, 287.0929576732586, 282.92302935895236, 279.5152255023466, 276.6053133030702, 273.6349471832769, 270.9275198205862, 268.91258069811846, 266.3754239802364, 264.12243575774323, 262.1061539155448, 259.5451897167093, 257.01049073960996, 254.36653973423404, 252.13836280091098, 250.53435477244744, 248.07179665148792, 246.40583631615047, 244.42090073987723, 242.55060742996818, 241.3813443421755, 240.59260164220058, 238.9506832822024, 237.8205406805958, 236.60407824556836, 235.13900548222, 234.14133658058623, 232.59868341070393, 231.73338190769118, 230.2825873331934, 228.69536532555273, 227.91287416971053, 227.1084209606917, 226.25590519126072, 225.72103811871628, 224.6387496146046, 223.29644616000556, 222.2238419335232, 221.53109098699983, 221.2937476967148, 220.32202733428286, 219.2597071141037, 218.2977313012283, 217.53075649472422, 216.80459036951626, 216.04610797625247, 215.70592273759226, 215.75135884557972, 214.94408790950501, 214.20773047954773, 213.56275834788082, 213.14258726502786, 212.23704981034163, 211.85124388194834, 211.80909793916257, 211.5689182100817, 210.95246842172062, 210.9055666280634, 210.74729732548656, 210.05950244219966, 209.3375211863561, 208.67367295419191, 208.24168888264632, 208.1589672598287, 207.95613624548912, 207.3829991499683, 207.22786103614163, 206.58180764007122, 206.17560059034565, 205.32879394157345, 205.1191605214109, 205.00031408528102, 204.84971417013773, 204.7651403851408, 204.68185324375688, 204.1694944960316, 203.8048326798085, 203.52911108866942, 203.05292912120453, 203.09648003125463, 202.88526989603292, 202.72272301953208, 202.93828402563685, 202.62305557779078, 202.4414452062973, 202.01559642535946, 201.8505453757855, 201.87664261489184, 201.60756291012157, 201.7101230019129, 201.66882417201376, 201.02448457744214, 200.82291397617794, 200.6024539539036, 200.163987901327, 200.3940086429342, 200.3879838088129, 200.22149781948076, 200.37838200480365, 200.04023159986716, 199.7795773497448, 199.46336241418595, 199.03619913913118, 199.4330759593052, 199.72531933031618, 199.52889174391194, 199.19879458190206, 198.64810579038107, 198.33923090244164, 198.1858223619005, 198.27863552187932, 198.70698215785293, 198.4814958985534, 198.7498078429801, 198.94755564356842, 198.4388566551894, 198.28489772515786, 198.05839700883016, 197.72267936027362, 197.89659927958886, 198.05789540589495, 198.16866851474214, 198.16023035600145, 197.75518520829036, 197.52616623163735, 197.25183832895218, 197.06299073178556, 197.09071524377964, 197.2887474424082, 197.47380290649926, 197.59933578567416, 197.1967818895313, 196.88171981429764, 196.73206259770708, 196.58980294639485, 196.967761320033, 197.1709141212856, 197.00898729485866, 196.98202523988053, 196.72073098055117, 196.3565661657181, 196.23851024928035, 196.23931561147188, 196.66685175684975, 196.9219491544376, 196.91019357929775, 196.96950191509188, 196.48785403158038, 196.27189635202618, 196.20896553654632, 195.97271117097807, 196.42125940307622, 196.67854187477192, 196.7134347221531, 196.69011829461326, 196.24093093117634, 195.8780259471241, 195.73321524396633, 195.99880610283262, 196.35894472846712, 196.53035865845223, 196.59204285193977, 196.40555920927054, 195.9189360090688, 195.9107761633996, 195.62958442893367, 195.29986704935217, 195.50411626434544, 195.60433638496184, 195.79430003459342, 195.8547080946132, 195.52835733891195, 195.39317979449805, 195.2988845717582, 195.048527069851, 195.4783054931894, 195.68438423021274, 195.68556063667714, 195.74835813237078, 195.49427793372791, 195.35298911510355, 195.15768375365826, 195.21372563507347, 196.0032049025182, 196.1515486749575, 195.96777205013035, 195.75874213986387, 195.36968044963274, 195.07065132535612, 195.1368941827421, 194.82625118425716, 195.20644540070302, 195.3890922712121, 195.4476446922792, 195.53526693723262, 195.29678732084065, 195.01614388591625, 194.84664582325212, 194.89576615048355, 195.32649779344925, 195.51385465392963, 195.4316081481693, 195.43899872998162, 195.1643293410154, 195.0170698799429, 194.8825773213155, 194.90229336519923, 195.20668061708704, 195.4169806917246, 195.77144548207332, 195.82501696018088, 195.39229912005266, 195.1969559348719, 195.19103959564453, 195.14128480905129, 195.2133874666717, 195.27310759201342, 195.41086756478313, 195.29258829769324, 194.82602947522432, 194.6451692931181, 194.55403824937216, 194.87062314290452, 195.207768376259, 195.23882610148002, 195.27726753070763, 195.28309958397418, 195.10043047976748, 194.92255876251372, 194.70091777238324, 194.46873746090765, 195.03429704841474, 195.34820910661017, 195.33315896313653, 195.21925863675455, 194.8160040655512, 194.60794748513487, 194.6833049501572, 194.69297195240998, 195.01481097851533, 195.08757144388406, 195.09227756210203, 195.23551010707703, 194.97586949658736, 194.72648659834667, 194.59729223460752, 194.43639286597275, 194.85440496347582, 195.16372954257957, 195.19901647059294, 195.16659352298694, 194.7785671861925, 194.5737419781663, 194.63587431101845, 194.6861365004625]]]
  in  "Associated files":T5
  in  "Pulse properties":T6={"N pulses"=0, "Samples"=0, "Last samples"=0, "AO pulse ticks"=0, "Skip samples"=0, "N samples/decay"=0, "Sliding Step \n(nb pulses)"=0, "Slidiing window\n (nb pulses)"=0, "Interpoints \ninterval (ms)"=100.0, "Repeat \neach point"=8, "Number of points"=0, "Mean and Time-Lapsed on Point Number"=0, "Oxygen dye type"=10106, "N samples/ decay min"=0, "Interpulse Interval"=0.0, "Wait"=30} {"Oxygen dye type" items=["PtP-C343 (30 kDa)", "PtP-C343 (65 KDa)"]; "Repeat \neach point" min=2 step=1}
  out "Raw Data Image":T3[][](array[typedef])=[["Phosphorescence decay Raw - Point 1 - Channel1"], ["Phosphorescence decay Raw - Point 1 - Channel2"]]
  out "localTimeData":timestamp[][](array[timestamp])=[[timestamp(3535365076.1922503 s since 1904-01-01)]]
  out "ForceEnd":bool
  in  "Channel Acq":u16(ring)=1 items=["1", "1&2"]
  in  "Interpoints interval (ms)":dbl=100.0
  in  "Repeat each point":i64=1 min=0
  in  "waveformType":waveform(dbl) caption="waveform"
  out "Raw Data Display":T3
  in  "Display raw changed":bool
  out "Local Raw Data":T3
  out "Image 8bit":T3
  out "Image To Save":T3
  out "Task AI":refnum<k21> caption="task out"
  in  "Last samples":i32=15
  out "Analyse":bool
  in  "Skip samples":i32=45
  out "N samples/decay":i32=312
  in  "AO pulse ticks":i32=30 min=2 step=1
  in  "Interpulse interval (us)":dbl=249.6 caption="Interpulse\ninterval (us)"
  in  "N pulses per point":i32=40000 min=100 max=2147483600 step=100
  out "Total time per point (s)":dbl=4.992 max=599.99
  out "Samples":i64=12480000
  in  "stop":bool
  in  "Scan rate (kHz)":dbl=1250.0 caption="Rate (kHz)" max=5000.0
  # "File Information"
  # "Analysis"
  # "Display Raw Data"
  # "Results :"
  # "Limit analysis"
  # "Time Periods\nRBC\n\nInter RBC"
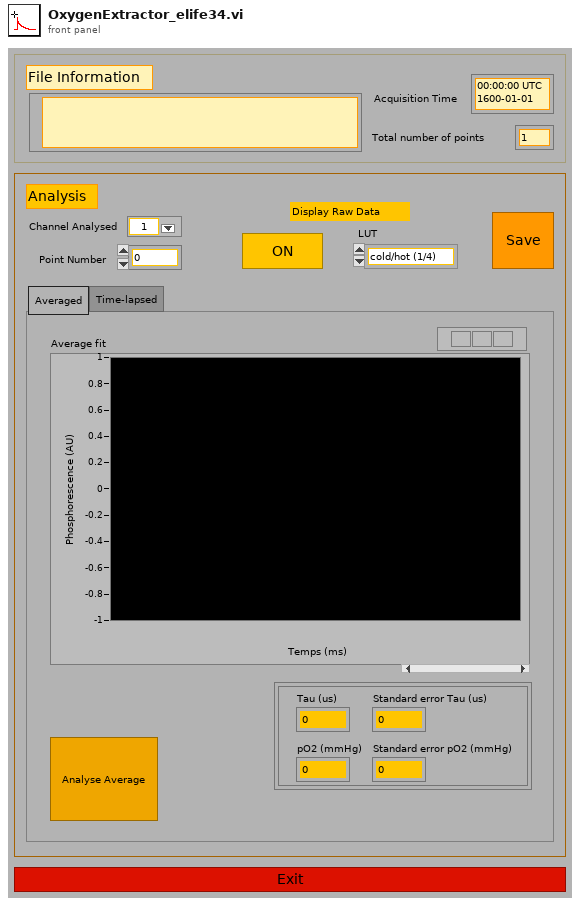
[diagram p1: front panel]
types:
  T1 = cluster{"amplitude":dbl, "Area (au)":dbl, "Tau (us)":dbl, "Standard error pO2 (mmHg)":dbl, "pO2 (mmHg)":dbl, "Standard error Tau (us)":dbl}[]
  T2 = cluster{"scan rate (kHz)":dbl, "Selection coordinates":dbl[], "Channel Acq":u16, "pwr_rel":dbl, "Pictures coordinates":dbl[], "MP synch":bool}
  T3 = typedef "IMAQ Image.ctl" = refnum<image>
  T4 = cluster{"Conversion Method":u32, "Minimum Value":i32, "Maximum Value":i32, "# Shifts":i32}
  T5 = cluster{"Raw Images file":string[][], "Mean and fit file":string, "Reference image files":string[], "Reference text file":string, "Timing file":string, "Results file":string, "TDMS path":string}
  T6 = cluster{"N pulses":i32, "Samples":i32, "Last samples":i32, "AO pulse ticks":i32, "Skip samples":i32, "N samples/decay":i32, "Sliding Step \n(nb pulses)":i32, "Slidiing window\n (nb pulses)":i32, "Interpoints \ninterval (ms)":dbl, "Repeat \neach point":i32, "Number of points":i32, "Mean and Time-Lapsed on Point Number":i32, "Oxygen dye type":i16, "N samples/ decay min":i32, "Interpulse Interval":dbl, "Wait":i32}
  T7 = enum32{"AutoM", "Close", "Dilate", "Erode", "Gradient", "Gradient out", "Gradient in", "Hit miss", "Open", "PClose", "POpen", "Thick", "Thin"}
  T8 = typedef "Image Type" = u32
  T9 = cluster{"scan rate (kHz)":dbl, "Selection coordinates":dbl[], "Channel":i32, "pwr_rel":dbl, "Pictures coordinates":dbl[]}
  T10 = cluster{"Mean and fit file":string, "Reference image files":string[], "Reference text file":string, "Results file":string, "Timing file":string, "Raw Images file":string[][], "TDMS path":string}
  T11 = cluster{"N pulses":i32, "Samples":i32, "Last samples":i32, "AO pulse ticks":i32, "Skip samples":i32, "N samples/decay":i32, "Sliding Step \n(nb pulses)":i32, "Slidiing window\n (nb pulses)":i32, "Interpoints \ninterval (ms)":dbl, "Mean and Time-Lapsed on Point Number":i32, "Number of points":i32, "Repeat \neach point":i32, "Oxygen dye type":i16, "Interpulse Interval":dbl, "N samples/ decay min":i32}
  T12 = cluster{"amplitude":dbl, "Area (au)":dbl, "Tau (us)":dbl, dbl, dbl, "Standard error Tau (us)":dbl}
  T13 = cluster{"Lower value":sgl, "Upper value":sgl, "Replace Value":sgl, "Keep/Replace Value (Replace)":bool}[]
  T14 = cluster{"amplitude":dbl, "Area (au)":dbl, "Tau (us)":dbl, "element":dbl, "element 2":dbl, "Standard error Tau (us)":dbl}
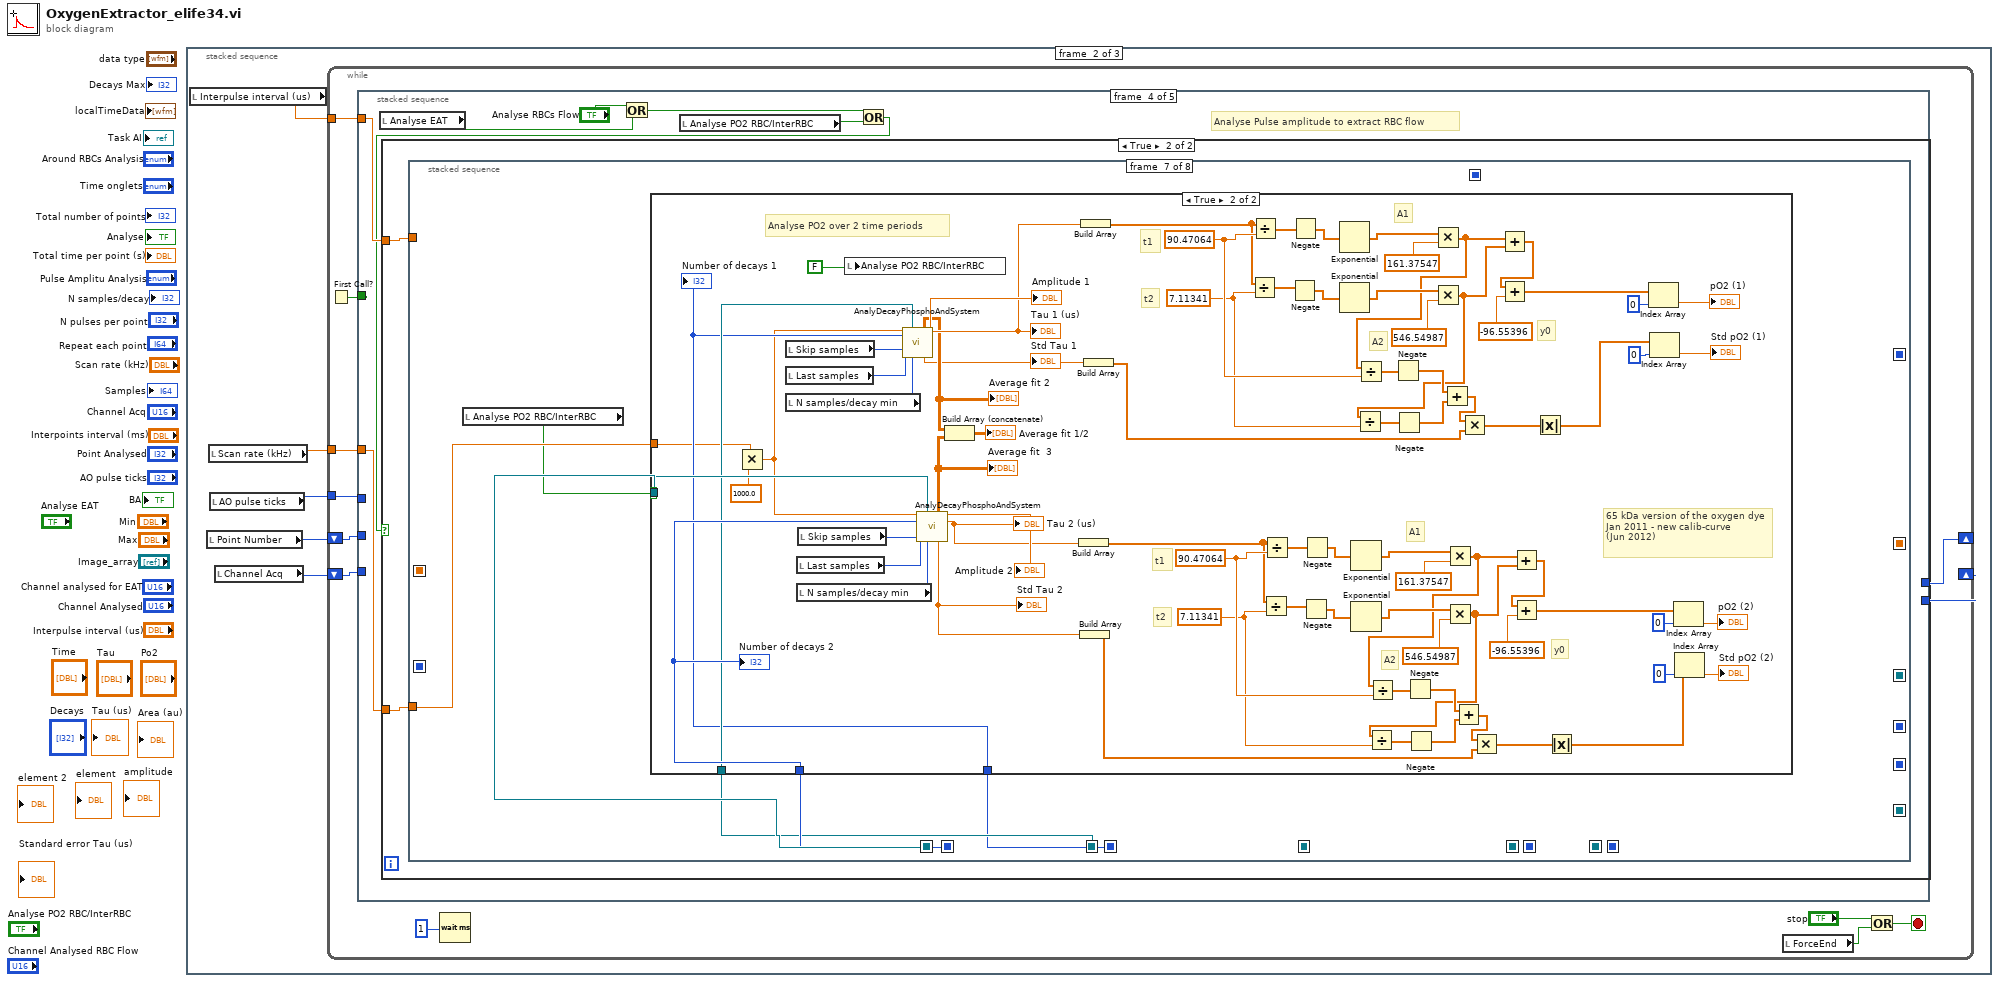
[diagram p0: block diagram]
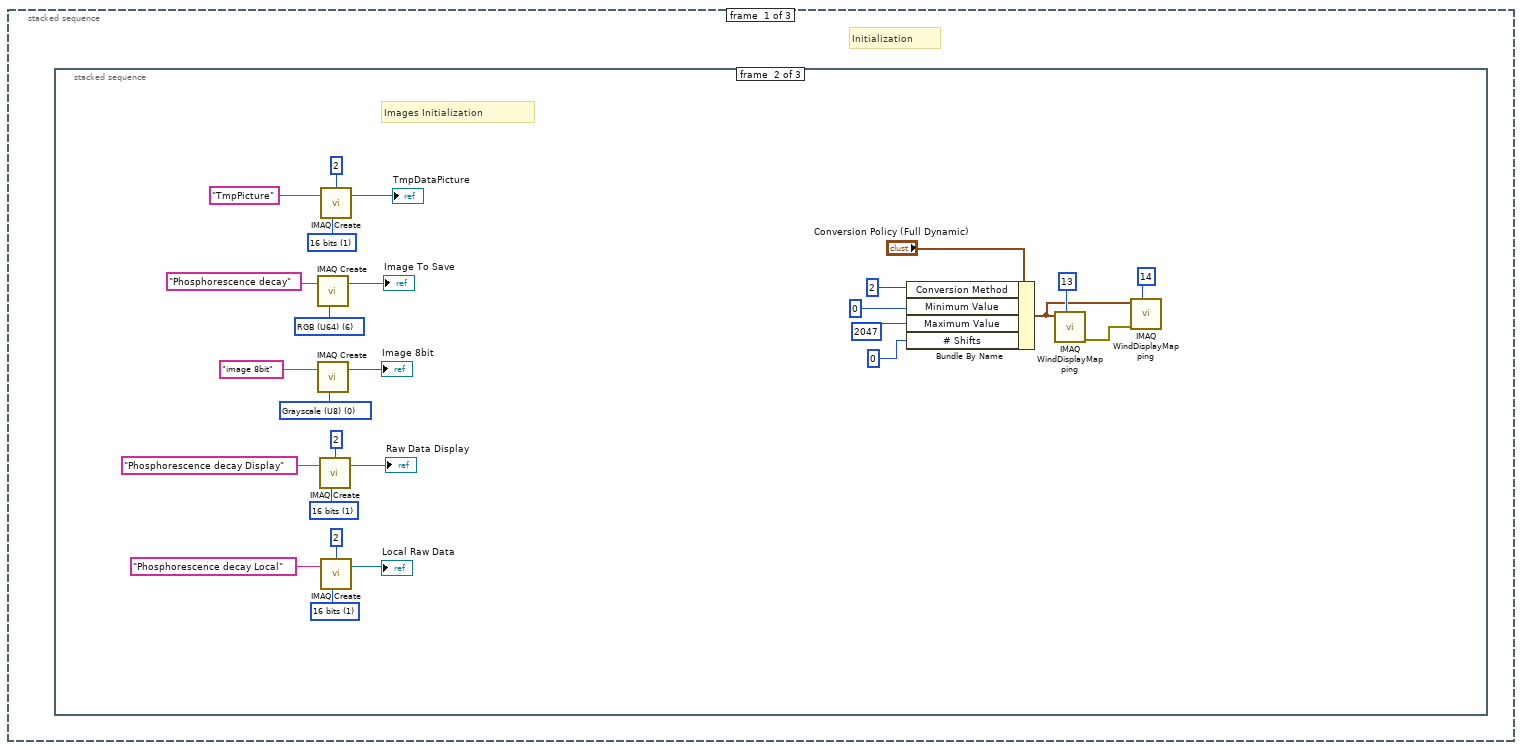
[diagram p2: hidden frame]
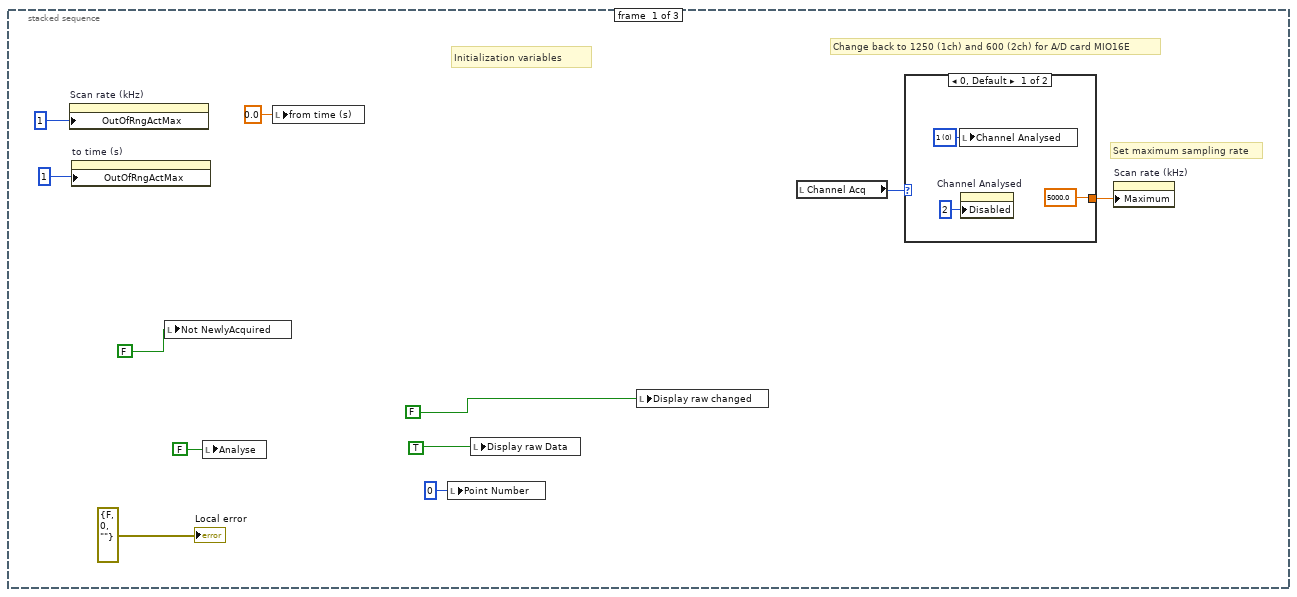
[diagram p3: hidden frame]
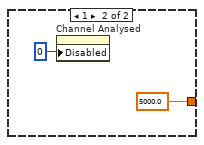
[diagram p4: hidden frame]
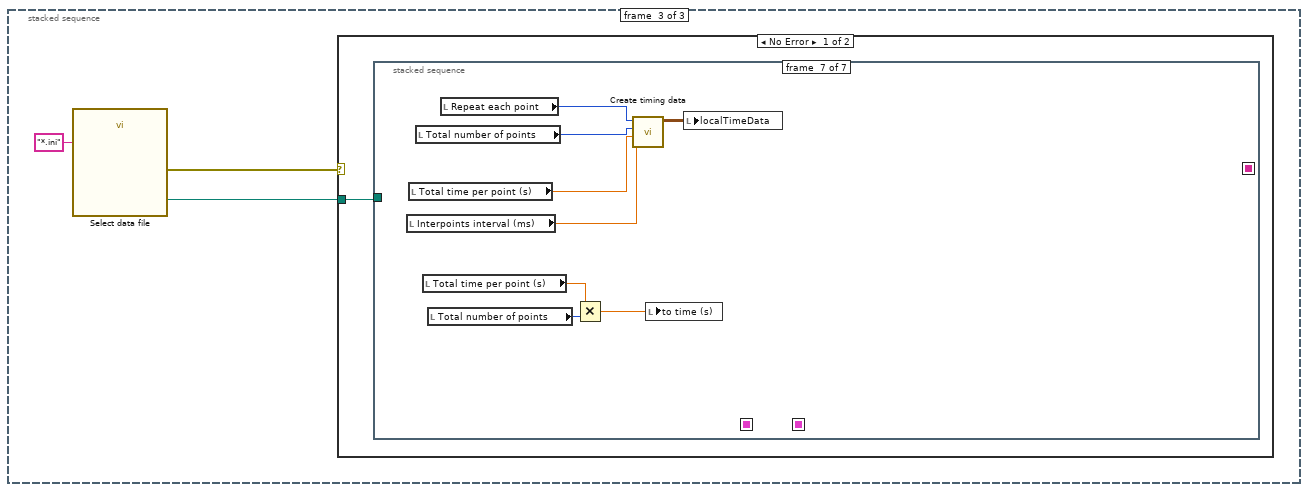
[diagram p5: hidden frame]
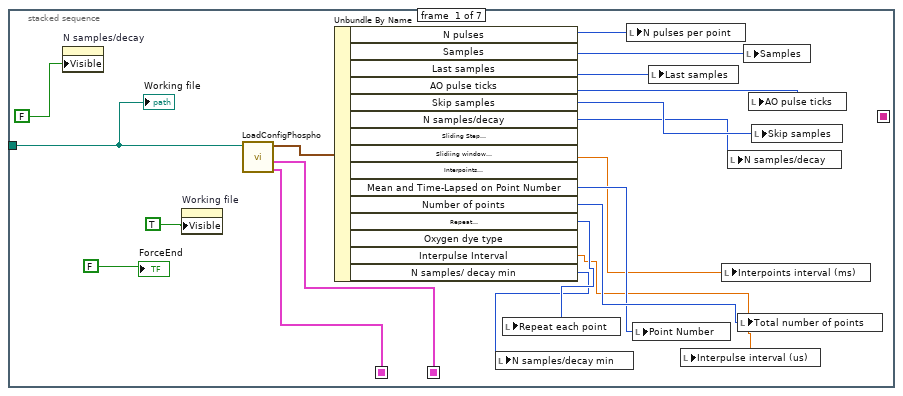
[diagram p6: hidden frame]
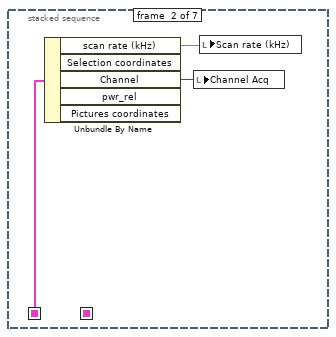
[diagram p7: hidden frame]
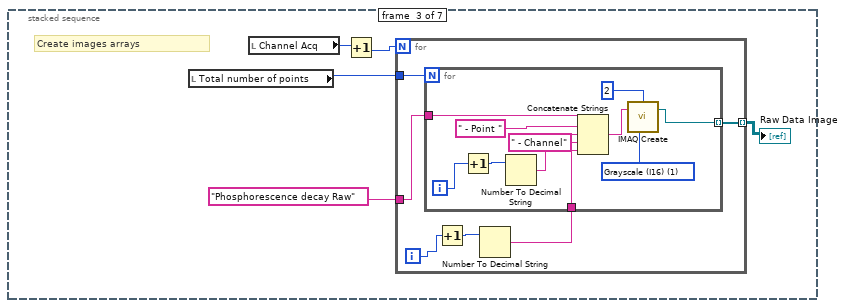
[diagram p8: hidden frame]
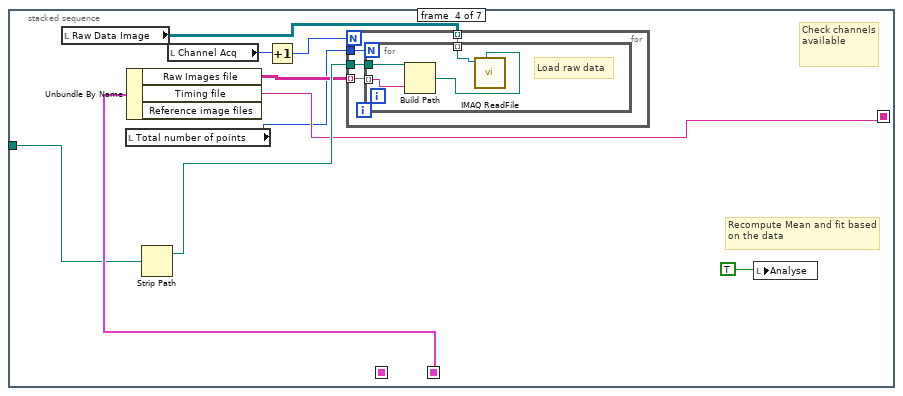
[diagram p9: hidden frame]
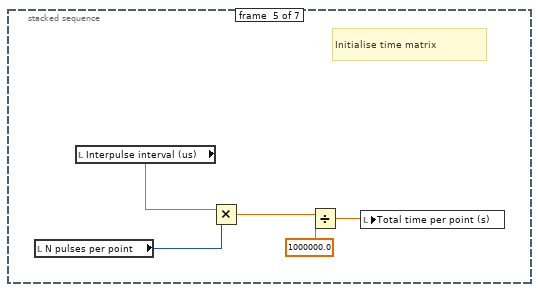
[diagram p10: hidden frame]
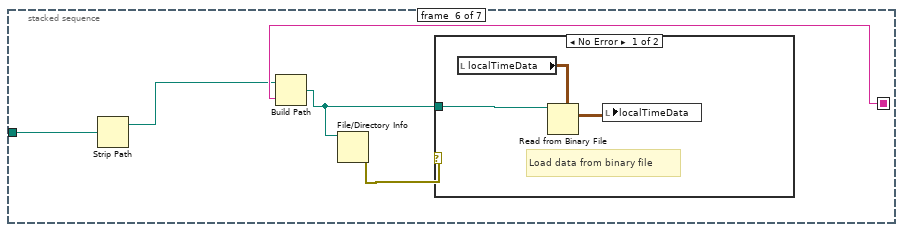
[diagram p11: hidden frame]
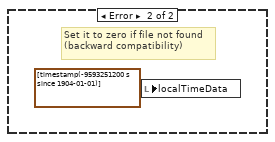
[diagram p12: hidden frame]
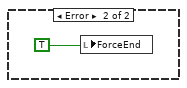
[diagram p13: hidden frame]
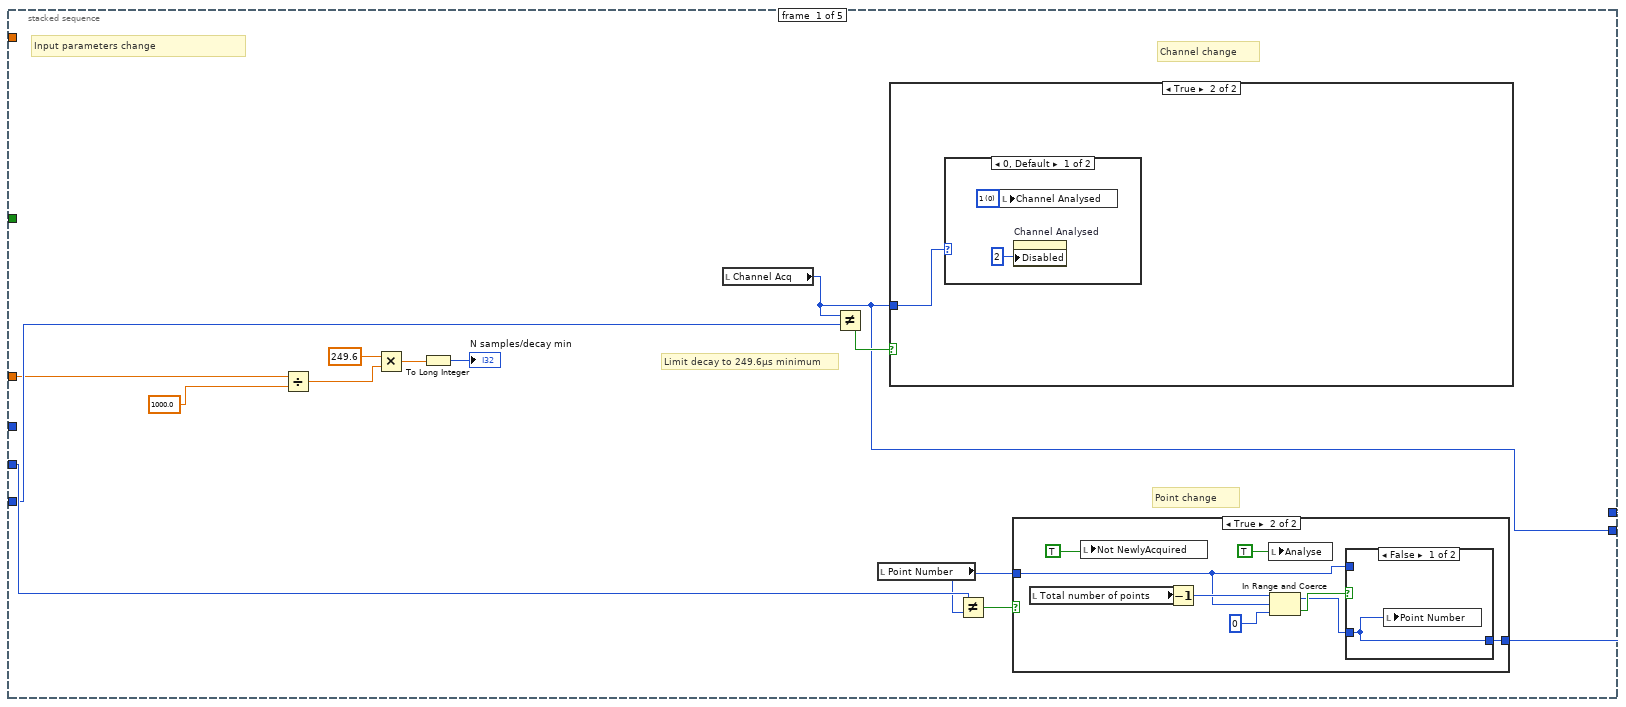
[diagram p14: hidden frame]
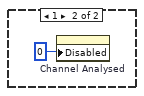
[diagram p16: hidden frame]
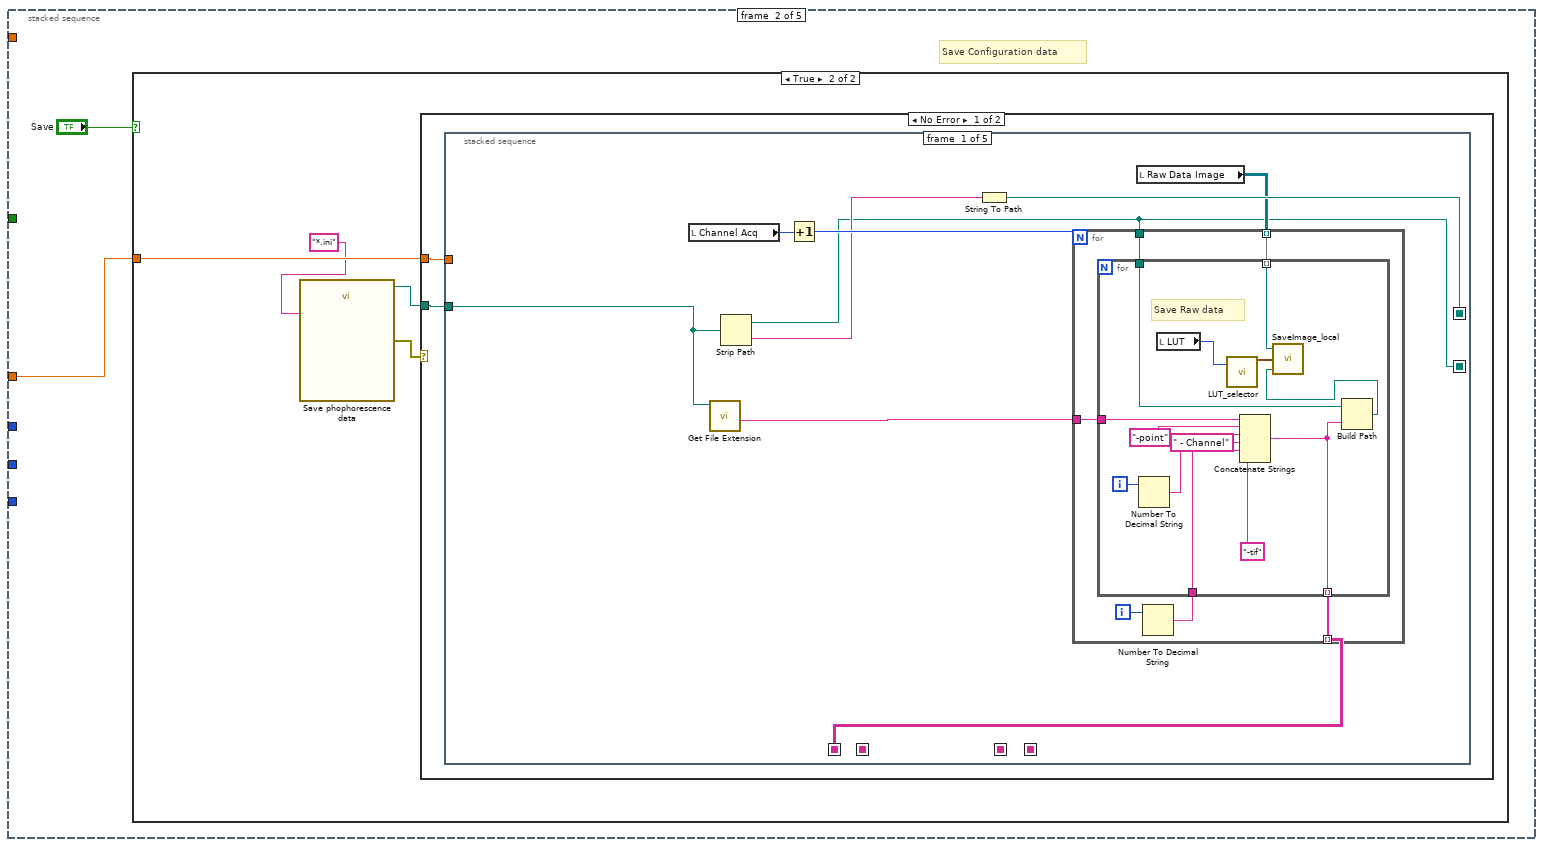
[diagram p19: hidden frame]
diagram:
  n1 = stacked-sequence {
    frame #0 {
      # "Initialization"
      n2 = stacked-sequence {
        frame #0 {
          # "Initialization variables"
          # "Change back to 1250 (1ch) and 600 (2ch) for A/D card MIO16E"
          # "Set maximum sampling rate"
          n3 = property on="Scan rate (kHz)" class="DigNum (strict)"("OutOfRngActMax"=u8 1 ("Réponse aux valeurs hors gamme : maximum")) -> ()  [unwired: 2 in, 2 out]
          n4 = property on="to time (s)" class="DigNum (strict)"("OutOfRngActMax"=u8 1 ("Réponse aux valeurs hors gamme : maximum")) -> ()  [unwired: 2 in, 2 out]
          n5 = local write "Not NewlyAcquired"(FALSE ("Acquire")) -> ()
          n6 = local write "Analyse"(FALSE ("Analyse")) -> ()
          n7 = local write "from time (s)"(0.0 ("from time (s)")) -> ()
          n8 = local write "Point Number"(0 ("Point Number")) -> ()
          n9 = local write "Display raw Data"(TRUE) -> ()
          n10 = local write "Display raw changed"(FALSE ("Display raw")) -> ()
          n11 = local read "Channel Acq"() -> (w8:u16)
          n12 = case shown="0, Default" w8 {
            tunnel: [5000.0 ("Limites d'entrée des données : maximum") 5000.0 ("Limites d'entrée des données : maximum")] -> w7
            frame 0, Default {
              w12 = u16 0 items=["1", "2"] ("Acq  & Analyse Ch")
              n13 = local write "Channel Analysed"(w12) -> ()
              n14 = property on="Channel Analysed" class="Ring (strict)"("Disabled"=u8 2 ("Désactivé")) -> ()  [unwired: 2 in, 2 out]
            }
            frame 1 {
              n15 = property on="Channel Analysed" class="Ring (strict)"("Disabled"=u8 0 ("Désactivé")) -> ()  [unwired: 2 in, 2 out]
            }
          }
          n16 = property on="Scan rate (kHz)" class="DigNum (strict)"("Maximum"=w7) -> ()  [unwired: 2 in, 2 out]
          "Local error" <- errorcluster {"status"=FALSE, "code"=0, "source"=""} ("Local error")
        }
        frame #1 {
          w19 = u32 1 items=["8 bits", "16 bits", "Float", "Complex", "RGB", "HSL"] ("Image Type")
          w23 = u32 1 items=["8 bits", "16 bits", "Float", "Complex", "RGB", "HSL"] ("Image Type")
          w28 = T8 0 items=["Grayscale (U8)", "Grayscale (I16)", "Grayscale (SGL)", "Complex (CSG)", "RGB (U32)", "HSL (U32)", "RGB (U64)", "Grayscale (U16)"] ("Image Type")
          w29 = T8 6 items=["Grayscale (U8)", "Grayscale (I16)", "Grayscale (SGL)", "Complex (CSG)", "RGB (U32)", "HSL (U32)", "RGB (U64)", "Grayscale (U16)"] ("Image Type")
          w33 = u32 1 items=["8 bits", "16 bits", "Float", "Complex", "RGB", "HSL"] ("Image Type")
          # "Images Initialization"
          n17 = call "IMAQ Create"("Image Name"="Phosphorescence decay" ("Title"), "Image Type"=w29) -> ("New Image"=→"Image To Save":T3)  [unwired: 2 in, 2 out]
          n18 = call "IMAQ Create"("Image Name"="image 8bit", "Image Type"=w28) -> ("New Image"=→"Image 8bit":T3)  [unwired: 2 in, 2 out]
          n19 = call "IMAQ Create"("Border Size"=2, "Image Name"="Phosphorescence decay Display", "Image Type"=w19) -> ("New Image"=→"Raw Data Display":T3)  [unwired: 1 in, 2 out]
          n20 = call "IMAQ Create"("Border Size"=2, "Image Name"="TmpPicture", "Image Type"=w33) -> ("New Image"=→"TmpDataPicture":T3)  [unwired: 1 in, 2 out]
          n21 = call "IMAQ Create"("Border Size"=2, "Image Name"="Phosphorescence decay Local", "Image Type"=w23) -> ("New Image"=→"Local Raw Data":T3)  [unwired: 1 in, 2 out]
          n22 = Bundle By Name(cluster="Conversion Policy (Full Dynamic)", "Conversion Method"=u32 2, "Minimum Value"=0, "Maximum Value"=2047, "# Shifts"=0) -> (w37:T4)
          n23 = call "IMAQ WindDisplayMapping"("Window Number (0...15)"=13, "Conversion Policy (Default)"=w37) -> ("error out"=w36:errorcluster)  [unwired: 2 in, 7 out]
          n24 = call "IMAQ WindDisplayMapping"("Window Number (0...15)"=14, "error in (no error)"=w36, "Conversion Policy (Default)"=w37) -> ()  [unwired: 1 in, 8 out]
        }
        frame #2 {
          n25 = call "Select data file"("pattern (all files)"="*.ini") -> ("selected path"=w45:path, "error out"=w44:errorcluster)  [unwired: 6 in, 7 out]
          n26 = case shown="No Error" w44 {
            tunnel: w45 -> [w47 _]
            frame No Error {
              n27 = stacked-sequence {
                seq-local: [w65 _ _ _ _ _ _] -> [_ w69 _ _ _ _ _]
                seq-local: [w64 _ _ _ _ _ _] -> [_ _ _ w101 _ _ _]
                seq-local: [_ _ _ w96 _ _ _] -> [_ _ _ _ _ w118 _]
                tunnel: w47 -> [w57 _ _ w100 _ w119 _]
                frame #0 {
                  n28 = property on="N samples/decay" class="DigNum (strict)"("Visible"=FALSE) -> ()  [unwired: 2 in, 2 out]
                  n29 = property on="Working file" class="Path"("Visible"=TRUE) -> ()  [unwired: 2 in, 2 out]
                  n30 = call "LoadConfigPhospho.vi"("configuration file path"=w57) -> ("Acquisition properties"=w65:T9, "Associated files"=w64:T10, "Pulse properties"=w66:T11)  [unwired: 5 out]
                  n31 = Unbundle By Name(w66) -> ("N pulses"=w63:i32, "Samples"=w62:i32, "Last samples"=w61:i32, "AO pulse ticks"=w60:i32, "Skip samples"=w59:i32, "N samples/decay"=w58:i32, "Interpoints \ninterval (ms)"=w52:dbl, "Mean and Time-Lapsed on Point Number"=w53:i32, "Number of points"=w54:i32, "Repeat \neach point"=w55:i32, "Interpulse Interval"=w49:dbl, "N samples/ decay min"=w50:i32)  [unwired: 3 out]
                  n32 = local write "N samples/decay min"(w50) -> ()
                  n33 = local write "Repeat each point"(w55) -> ()
                  n34 = local write "N pulses per point"(w63) -> ()
                  n35 = local write "Point Number"(w53) -> ()
                  n36 = local write "Last samples"(w61) -> ()
                  n37 = local write "Interpulse interval (us)"(w49) -> ()
                  n38 = local write "Interpoints interval (ms)"(w52) -> ()
                  n39 = local write "N samples/decay"(w58) -> ()
                  n40 = local write "Total number of points"(w54) -> ()
                  n41 = local write "Samples"(w62) -> ()
                  n42 = local write "AO pulse ticks"(w60) -> ()
                  n43 = local write "Skip samples"(w59) -> ()
                  "ForceEnd" <- FALSE ("stop")
                  "Working file" <- w57
                }
                frame #1 {
                  n44 = Unbundle By Name(w69) -> ("scan rate (kHz)"=w67:dbl, "Channel"=w68:i32)  [unwired: 3 out]
                  n45 = local write "Channel Acq"(w68) -> ()
                  n46 = local write "Scan rate (kHz)"(w67) -> ()
                }
                frame #2 {
                  # "Create images arrays"
                  n47 = local read "Total number of points"() -> (w70:i32)
                  n48 = local read "Channel Acq"() -> (w73:u16)
                  n49 = Increment(x=w73) -> (x+1=w72:u16)
                  n50 = for {
                    N: w72 -> [_]
                    tunnel: "Phosphorescence decay Raw" ("Image Name") -> [w80]
                    tunnel: [w79] -> w71 mode=indexing
                    tunnel: w70 -> [w75]
                    i -> [w77]
                    n51 = Increment(x=w77) -> (x+1=w78:i32)
                    n52 = Number To Decimal String(number=w78) -> (decimal integer string=w76:string)  [unwired: 1 out]
                    n53 = for {
                      N: w75 -> [_]
                      tunnel: w80 -> [w89]
                      tunnel: [w90] -> w79 mode=indexing
                      tunnel: w76 -> [w82]
                      i -> [w86]
                      w81 = T8 1 items=["Grayscale (U8)", "Grayscale (I16)", "Grayscale (SGL)", "Complex (CSG)", "RGB (U32)", "HSL (U32)", "RGB (U64)", "Grayscale (U16)"] ("Image Type")
                      n54 = Increment(x=w86) -> (x+1=w85:i32)
                      n55 = Number To Decimal String(number=w85) -> (decimal integer string=w84:string)  [unwired: 1 out]
                      n56 = Concatenate Strings(w89, " - Point " ("chaîne"), w84, " - Channel" ("chaîne"), w82) -> (w88:string)
                      n57 = call "IMAQ Create"("Border Size"=2, "Image Name"=w88, "Image Type"=w81) -> ("New Image"=w90:T3)  [unwired: 1 in, 2 out]
                    }
                  }
                  "Raw Data Image" <- w71
                }
                frame #3 {
                  # "Check channels available"
                  # "Recompute Mean and fit based on the data"
                  n58 = local read "Raw Data Image"() -> (w92:T3[][])
                  n59 = local read "Total number of points"() -> (w93:i32)
                  n60 = Unbundle By Name(w101) -> ("Raw Images file"=w97:string[][], "Timing file"=w96:string)  [unwired: 1 out]
                  n61 = Strip Path(path=w100) -> (stripped path=w98:path)  [unwired: 1 out]
                  n62 = local read "Channel Acq"() -> (w95:u16)
                  n63 = Increment(x=w95) -> (x+1=w94:u16)
                  n64 = for {
                    N: w94 -> [_]
                    tunnel: w98 -> [w105]
                    tunnel: w97 -> [w104] mode=indexing
                    tunnel: w92 -> [w103] mode=indexing
                    tunnel: w93 -> [w102]
                    n65 = for {
                      N: w102 -> [_]
                      tunnel: w105 -> [w109]
                      tunnel: w104 -> [w108] mode=indexing
                      tunnel: w103 -> [w106] mode=indexing
                      # "Load raw data"
                      n66 = Build Path(base path=w109, name or relative path=w108) -> (appended path=w107:path)
                      n67 = call "IMAQ ReadFile"("File Path"=w107, "Image"=w106) -> ()  [unwired: 3 in, 7 out]
                    }
                  }
                  n68 = local write "Analyse"(TRUE ("Acquired")) -> ()
                }
                frame #4 {
                  # "Initialise time matrix"
                  n69 = local read "N pulses per point"() -> (w113:i32)
                  n70 = local read "Interpulse interval (us)"() -> (w114:dbl)
                  n71 = Multiply(x=w114, y=w113) -> (x*y=w112:dbl)
                  n72 = Divide(x=w112, y=1000000.0) -> (x/y=w111:dbl)
                  n73 = local write "Total time per point (s)"(w111) -> ()
                }
                frame #5 {
                  n74 = Strip Path(path=w119) -> (stripped path=w117:path)  [unwired: 1 out]
                  n75 = Build Path(base path=w117, name or relative path=w118) -> (appended path=w116:path)
                  n76 = File/Directory Info(path=w116) -> (error out=w115:errorcluster)  [unwired: 1 in, 6 out]
                  n77 = case shown="No Error" w115 {
                    tunnel: w116 -> [w120 _]
                    frame No Error {
                      # "Load data from binary file"
                      n78 = local read "localTimeData"() -> (w121:timestamp[][])
                      n79 = Read from Binary File(5:w121, 11:w120) -> (2:w122:timestamp[][])  [unwired: 1 in, 6 out]
                      n80 = local write "localTimeData"(w122) -> ()
                    }
                    frame Error {
                      # "Set it to zero if file not found (backward compatibility)"
                      n81 = local write "localTimeData"(timestamp[][] [[timestamp(-9593251200 s since 1904-01-01)]] ("localTimeData")) -> ()
                    }
                  }
                }
                frame #6 {
                  n82 = local read "Interpoints interval (ms)"() -> (w128:dbl)
                  n83 = local read "Total time per point (s)"() -> (w129:dbl)
                  n84 = local read "Total number of points"() -> (w130:i32)
                  n85 = local read "Total time per point (s)"() -> (w125:dbl)
                  n86 = local read "Total number of points"() -> (w124:i32)
                  n87 = local read "Repeat each point"() -> (w131:i64)
                  n88 = Multiply(x=w125, y=w124) -> (x*y=w126:dbl)
                  n89 = call "Create timing data.vi"("Interpoints \ninterval (ms)"=w128, "Total time per point (s)"=w129, "Number of points"=w130, "Repeat \neach point"=w131) -> ("localTimeData"=w127:timestamp[][])  [unwired: 7 in]
                  n90 = local write "to time (s)"(w126) -> ()
                  n91 = local write "localTimeData"(w127) -> ()
                }
              }
            }
            frame Error {
              n92 = local write "ForceEnd"(TRUE ("stop")) -> ()
            }
          }
        }
      }
    }
    frame #1 {
      n93 = local read "Interpulse interval (us)"() -> (w134:dbl)
      n94 = local read "Point Number"() -> (w137:i32)
      n95 = local read "Scan rate (kHz)"() -> (w135:dbl)
      n96 = local read "AO pulse ticks"() -> (w133:i32)
      n97 = local read "Channel Acq"() -> (w136:u16)
      n98 = while {
        shift-right: [w146] -> _
        shift-left: w137 -> [w147]
        shift-right: [w144] -> _
        shift-left: w136 -> [w145]
        tunnel: w135 -> [w140]
        tunnel: w134 -> [w139]
        tunnel: w133 -> [w138]
        stop <- w149 stop-if-true
        n99 = First Call?() -> (First Call?: T/F=w142:bool)
        n100 = stacked-sequence {
          tunnel: w139 -> [_ _ _ w464 _]
          tunnel: w138 -> [_ _ _ _ _]
          tunnel: w147 -> [w161 _ _ _ _]
          tunnel: [w154 _ _ _ _] -> w146
          tunnel: w145 -> [w152 _ _ _ _]
          tunnel: [w151 _ _ _ _] -> w144
          tunnel: w142 -> [_ _ _ _ _]
          tunnel: w140 -> [w150 w179 w361 w465 _]
          frame #0 {
            # "Limit decay to 249.6µs minimum"
            # "Input parameters change"
            # "Point change"
            # "Channel change"
            n101 = Divide(x=w150, y=1000.0) -> (x/y=w158:dbl)
            n102 = Multiply(x=249.6, y=w158) -> (x*y=w156:dbl)
            n103 = To Long Integer(number=w156) -> (32bit integer=→"N samples/decay min":i32)
            n104 = local read "Channel Acq"() -> (w151:u16)
            n105 = Not Equal?(x=w151, y=w152) -> (x != y?=w153:bool)
            n106 = local read "Point Number"() -> (w160:i32)
            n107 = case shown="True" w153 {
              tunnel: w151 -> [_ w163]
              frame False {
              }
              frame True {
                n108 = case shown="0, Default" w163 {
                  frame 0, Default {
                    w165 = u16 0 items=["1", "2"] ("Acq  & Analyse Ch")
                    n109 = local write "Channel Analysed"(w165) -> ()
                    n110 = property on="Channel Analysed" class="Ring (strict)"("Disabled"=u8 2 ("Désactivé")) -> ()  [unwired: 2 in, 2 out]
                  }
                  frame 1 {
                    n111 = property on="Channel Analysed" class="Ring (strict)"("Disabled"=u8 0 ("Désactivé")) -> ()  [unwired: 2 in, 2 out]
                  }
                }
              }
            }
            n112 = Not Equal?(x=w161, y=w160) -> (x != y?=w162:bool)
            n113 = case shown="True" w162 {
              tunnel: [w167 w171] -> w154
              tunnel: w160 -> [w167 w170]
              frame False {
              }
              frame True {
                n114 = local read "Total number of points"() -> (w175:i32)
                n115 = local write "Not NewlyAcquired"(TRUE ("Not NewlyAcquired")) -> ()
                n116 = Decrement(x=w175) -> (x-1=w174:i32)
                n117 = local write "Analyse"(TRUE ("Analyse")) -> ()
                n118 = In Range and Coerce(upper limit=w174, x=w170, lower limit=0 ("limite inférieure")) -> (coerced(x)=w169:i32, In Range?=w172:bool)
                n119 = case shown="False" w172 {
                  tunnel: [w177 w178] -> w171
                  tunnel: w170 -> [_ w178]
                  tunnel: w169 -> [w177 _]
                  frame False {
                    n120 = local write "Point Number"(w177) -> ()
                  }
                  frame True {
                  }
                }
              }
            }
          }
          frame #1 {
            # "Save Configuration data"
            n121 = case shown="True" "Save" {
              tunnel: w179 -> [_ w184]
              frame False {
              }
              frame True {
                n122 = call "Save phophorescence data"("pattern (all files)"="*.ini") -> ("selected path"=w182:path, "error out"=w183:errorcluster)  [unwired: 6 in, 7 out]
                n123 = case shown="No Error" w183 {
                  tunnel: w184 -> [w186 _]
                  tunnel: w182 -> [w185 _]
                  frame No Error {
                    n124 = stacked-sequence {
                      seq-local: [w188 _ _ _ _] -> [_ w238 w268 w288 w356]
                      seq-local: [w195 _ _ _ _] -> [_ w239 w269 w289 w358]
                      seq-local: [w193 _ _ _ _] -> [_ _ _ _ w341]
                      seq-local: [_ w230 _ _ _] -> [_ _ _ _ w342]
                      seq-local: [_ _ w266 _ _] -> [_ _ _ _ w339]
                      seq-local: [_ _ _ w286 _] -> [_ _ _ _ w338]
                      tunnel: w186 -> [_ w231 _ _ _]
                      tunnel: w185 -> [w194 _ _ _ _]
                      frame #0 {
                        n125 = local read "Channel Acq"() -> (w192:u16)
                        n126 = call <vilib>:"Get File Extension.vi"("file"=w194) -> ("filename without extension"=w187:string)  [unwired: 1 in, 9 out]
                        n127 = Strip Path(path=w194) -> (stripped path=w188:path, name=w189:string)
                        n128 = Increment(x=w192) -> (x+1=w191:u16)
                        n129 = String To Path(string=w189) -> (path=w195:path)
                        n130 = local read "Raw Data Image"() -> (w190:T3[][])
                        n131 = for {
                          N: w191 -> [_]
                          tunnel: w187 -> [w201]
                          tunnel: w188 -> [w200]
                          tunnel: [w199] -> w193 mode=indexing
                          tunnel: w190 -> [w196] mode=indexing
                          i -> [w198]
                          n132 = Number To Decimal String(number=w198) -> (decimal integer string=w197:string)  [unwired: 1 out]
                          n133 = for {
                            tunnel: w201 -> [w214]
                            tunnel: w200 -> [w213]
                            tunnel: [w211] -> w199 mode=indexing
                            tunnel: w197 -> [w206]
                            tunnel: w196 -> [w205] mode=indexing
                            i -> [w208]
                            # "Save Raw data"
                            n134 = Number To Decimal String(number=w208) -> (decimal integer string=w209:string)  [unwired: 1 out]
                            n135 = local read "LUT"() -> (w203:u16)
                            n136 = call "LUT_selector.vi"("LUT1"=w203) -> ("Palette1"=w204:cluster{u8, u8, u8}[])  [unwired: 1 in, 1 out]
                            n137 = Concatenate Strings(w214, "-point" ("chaîne"), w209, " - Channel" ("chaîne"), w206, "-tif") -> (w211:string)
                            n138 = Build Path(base path=w213, name or relative path=w211) -> (appended path=w212:path)
                            n139 = call "SaveImage_local.vi"("File Path"=w212, "Color Palette"=w204, "Image"=w205) -> ()  [unwired: 1 in]
                          }
                        }
                      }
                      frame #1 {
                        # "Save Mean data"
                        n140 = Reciprocal(x=w231) -> (1/x=w236:dbl)
                        n141 = local read "localTimeData"() -> (w229:timestamp[][])
                        n142 = Multiply(x=0.001, y=w236) -> (x*y=w217:dbl)
                        n143 = local read "Point Number"() -> (w228:i32)
                        n144 = call <vilib>:"Get File Extension.vi"("file"=w239) -> ("filename without extension"=w240:string)  [unwired: 1 in, 9 out]
                        n145 = Array Subset(array=w229, index (col)=w228, length (col)=1 ("longueur")) -> (w225:timestamp[][])  [unwired: 2 in]
                        n146 = local read "Repeat each point"() -> (w226:i64)
                        n147 = Concatenate Strings(w240, "-Mean." ("chaîne"), "txt" ("chaîne")) -> (w230:string)
                        n148 = Build Path(base path=w238, name or relative path=w230) -> (appended path=w234:path)
                        n149 = local read "Total time per point (s)"() -> (w222:dbl)
                        n150 = Reshape Array(w225, w226) -> (w224:timestamp[])
                        n151 = To Double Precision Float(number=w224) -> (double precision float=w223:dbl[])
                        n152 = call-poly <vilib>:"Mean.vi"("X"=w223) -> ("mean"=w219:dbl)  [unwired: 1 out]
                        n153 = Divide(x=w222, y=2.0) -> (x/y=w220:dbl)
                        n154 = Add(x=w219, y=w220) -> (x+y=w218:dbl)
                        n155 = To Time Stamp(1:w218) -> (0:w215:timestamp)
                        n156 = for {
                          N: 3 -> [_]
                          tunnel: w217 -> [w245]
                          tunnel: [w249] -> w235 mode=indexing
                          tunnel: "NI_ChannelName" ("Channel Name") -> [w248]
                          tunnel: w215 -> [w247]
                          i -> [w246]
                          n157 = case shown="2" w246 {
                            selector: w246 -> [w253 w257 w264]
                            tunnel: [w252 w256 w259] -> w244
                            tunnel: ["Raw Data" "Exponential fit" "standard error"] -> w243
                            frame 0, Default {
                              n158 = local read "Average fit"() -> (w254:dbl[][])
                              n159 = Index Array(array=w254, index (row)=w253) -> (element=w252:dbl[])  [unwired: 1 in]
                            }
                            frame 1 {
                              n160 = local read "Average fit"() -> (w258:dbl[][])
                              n161 = Index Array(array=w258, index (row)=w257) -> (element=w256:dbl[])  [unwired: 1 in]
                            }
                            frame 2 {
                              n162 = local read "Average fit"() -> (w265:dbl[][])
                              n163 = Index Array(array=w265, index (row) #1=w264, index (row) #2=0 ("indice (ligne)")) -> (element #1=w262:dbl[], element #2=w261:dbl[])  [unwired: 2 in]
                              n164 = Subtract(x=w262, y=w261) -> (x-y=w259:dbl[])
                            }
                          }
                          n165 = Bundle By Name(cluster="waveformType", "Y"=w244, "t0"=w247, "dt"=w245) -> (w250:waveform(dbl))
                          n166 = Set Waveform Attribute(5:w243, 6:w248, 7:w250) -> (3:w249:waveform(dbl))  [unwired: 1 in, 2 out]
                        }
                        n167 = call "Écrire dans un fichier de mesures"("Signals"=w235, "File Name"=w234) -> ()  [unwired: 5 in, 13 out]
                      }
                      frame #2 {
                        # "Save timing parameters"
                        n168 = call <vilib>:"Get File Extension.vi"("file"=w269) -> ("filename without extension"=w271:string)  [unwired: 1 in, 9 out]
                        n169 = Concatenate Strings(w271, "-Timing data" ("chaîne"), ".dat" ("chaîne")) -> (w266:string)
                        n170 = local read "localTimeData"() -> (w273:timestamp[][])
                        n171 = Build Path(base path=w268, name or relative path=w266) -> (appended path=w267:path)
                        n172 = Write to Binary File(file (use dialog)=w267, data=w273) -> ()  [unwired: 1 in, 6 out]
                      }
                      frame #3 {
                        w276 = "\t"
                        # "Save Averaged Results"
                        n173 = local read "localTimeData"() -> (w293:timestamp[][])
                        n174 = local read "DataValues"() -> (w294:T1)
                        n175 = Concatenate Strings("Point" ("chaîne"), w276, "Time" ("chaîne"), w276, "Amplitude (au)" ("chaîne"), w276, "Area (au)" ("chaîne"), w276, "pO2 (mmHg)" ("chaîne"), w276, "Standard error pO2 (mmHg)" ("chaîne"), w276, "Tau (us)" ("chaîne"), w276, "Standard error Tau (us)" ("chaîne"), "\r\n") -> (w283:string)
                        n176 = for {
                          tunnel: w294 -> [w330] mode=indexing
                          tunnel: w293 -> [w320]
                          shift-right: [w299] -> w282
                          shift-left: w283 -> [w300]
                          i -> [w311]
                          w295 = "\t"
                          # "Average point of measure"
                          n177 = Unbundle By Name(w330) -> ("amplitude"=w319:dbl, "Area (au)"=w318:dbl, "pO2 (mmHg)"=w317:dbl, "Standard error pO2 (mmHg)"=w316:dbl, "Tau (us)"=w315:dbl, "Standard error Tau (us)"=w314:dbl)
                          n178 = local read "Repeat each point"() -> (w324:i64)
                          n179 = Array Subset(array=w320, index (col)=w311, length (col)=1 ("longueur")) -> (w323:timestamp[][])  [unwired: 2 in]
                          n180 = Number To Decimal String(number=w311) -> (decimal integer string=w309:string)  [unwired: 1 out]
                          n181 = Reshape Array(w323, w324) -> (w322:timestamp[])
                          n182 = local read "Total time per point (s)"() -> (w328:dbl)
                          n183 = Number To Exponential String(number=w314) -> (E-format string=w304:string)  [unwired: 3 out]
                          n184 = Concatenate Strings("Point ", w309) -> (w297:string)
                          n185 = To Double Precision Float(number=w322) -> (double precision float=w321:dbl[])
                          n186 = Number To Exponential String(number=w315) -> (E-format string=w303:string)  [unwired: 3 out]
                          n187 = Number To Exponential String(number=w316) -> (E-format string=w305:string)  [unwired: 3 out]
                          n188 = Number To Exponential String(number=w319) -> (E-format string=w308:string)  [unwired: 3 out]
                          n189 = Number To Exponential String(number=w318) -> (E-format string=w307:string)  [unwired: 3 out]
                          n190 = Number To Exponential String(number=w317) -> (E-format string=w306:string)  [unwired: 3 out]
                          n191 = call-poly <vilib>:"Mean.vi"("X"=w321) -> ("mean"=w329:dbl)  [unwired: 1 out]
                          n192 = Divide(x=w328, y=2.0) -> (x/y=w327:dbl)
                          n193 = Add(x=w329, y=w327) -> (x+y=w326:dbl)
                          n194 = To Time Stamp(1:w326) -> (0:w312:timestamp)
                          n195 = Format Date/Time String(time format string (%c)="%H:%M:%S%3u" ("chaîne de format de l'heure (%c)"), seconds (now)=w312) -> (date/time string=w296:string)  [unwired: 1 out]
                          n196 = Concatenate Strings(w297, w295, w296, w295, w308, w295, w307, w295, w306, w295, w305, w295, w303, w295, w304, "\r\n") -> (w301:string)
                          n197 = Concatenate Strings(w300, w301) -> (w299:string)
                        }
                        n198 = call <vilib>:"Get File Extension.vi"("file"=w289) -> ("filename without extension"=w291:string)  [unwired: 1 in, 9 out]
                        n199 = Concatenate Strings(w291, "-Results" ("chaîne"), ".txt" ("chaîne")) -> (w286:string)
                        n200 = Build Path(base path=w288, name or relative path=w286) -> (appended path=w287:path)
                        n201 = Write to Text File(file (use dialog)=w287, text=w282) -> ()  [unwired: 1 in, 4 out]
                      }
                      frame #4 {
                        # "Associated files"
                        # "Acquisition properties"
                        # "Pulse properties"
                        n202 = local read "N samples/decay min"() -> (w334:i32)
                        n203 = local read "Interpulse interval (us)"() -> (w333:dbl)
                        n204 = local read "N pulses per point"() -> (w354:i32)
                        n205 = local read "Samples"() -> (w353:i64)
                        n206 = local read "Last samples"() -> (w352:i32)
                        n207 = local read "Interpoints interval (ms)"() -> (w346:dbl)
                        n208 = local read "AO pulse ticks"() -> (w351:i32)
                        n209 = local read "Total number of points"() -> (w344:i32)
                        n210 = local read "Point Number"() -> (w335:i32)
                        n211 = local read "Skip samples"() -> (w350:i32)
                        n212 = local read "N samples/decay"() -> (w349:i32)
                        n213 = local read "Repeat each point"() -> (w345:i64)
                        n214 = Bundle(cluster="Pulse properties", "N pulses"=w354, "Samples"=w353, "Last samples"=w352, "AO pulse ticks"=w351, "Skip samples"=w350, "N samples/decay"=w349, "Interpoints \ninterval (ms)"=w346, "Repeat \neach point"=w345, "Number of points"=w344, "Mean and Time-Lapsed on Point Number"=w335, "N samples/ decay min"=w334, "Interpulse Interval"=w333) -> (w331:T6)  [unwired: 4 in]
                        n215 = local read "Channel Acq"() -> (w347:u16)
                        n216 = local read "Scan rate (kHz)"() -> (w348:dbl)
                        n217 = Bundle By Name(cluster="Associated files", "Raw Images file"=w341, "Mean and fit file"=w342, "Timing file"=w339, "Results file"=w338) -> (w340:T5)
                        n218 = Bundle(cluster="Acquisition properties", "scan rate (kHz)"=w348, "Channel Acq"=w347) -> (w336:T2)  [unwired: 4 in]
                        n219 = call <vilib>:"Get File Extension.vi"("file"=w358) -> ("filename without extension"=w359:string)  [unwired: 1 in, 9 out]
                        n220 = Concatenate Strings(w359, ".ini" ("chaîne")) -> (w357:string)
                        n221 = Build Path(base path=w356, name or relative path=w357) -> (appended path=w355:path)
                        n222 = call "SaveConfigPhospho.vi"("configuration file path"=w355, "Associated files"=w340, "Pulse properties"=w331, "Acquisition properties"=w336) -> ()  [unwired: 16 in]
                      }
                    }
                  }
                  frame Error {
                  }
                }
              }
            }
          }
          frame #2 {
            # "Average decays analysis"
            n223 = local read "Analyse"() -> (w362:bool)
            n224 = case shown="True" w362 {
              tunnel: w361 -> [_ w363]
              frame False {
              }
              frame True {
                n225 = stacked-sequence {
                  tunnel: w363 -> [w365 _]
                  frame #0 {
                    # "Analyse average of all pulses"
                    n226 = Multiply(x=w365, y=1000.0) -> (x*y=w364:dbl)
                    n227 = case shown="False" "Not NewlyAcquired" {
                      tunnel: w364 -> [w389 _]
                      frame False {
                        n228 = local read "Channel Analysed"() -> (w384:u16)
                        n229 = local read "Raw Data Image"() -> (w385:T3[][])
                        n230 = Index Array(array=w385, index (row)=w384) -> (element=w383:T3[])  [unwired: 1 in]
                        n231 = for {
                          N -> [w425]
                          tunnel: w389 -> [w439]
                          tunnel: w383 -> [w419] mode=indexing
                          tunnel: [w428] -> w388 mode=indexing
                          tunnel: [w427] -> w387 mode=indexing
                          i -> [w426]
                          stop <- w423 stop-if-true
                          w400 = 7.11341 ("y")
                          w402 = 90.47064 ("y")
                          # "y0"
                          # "A1"
                          # "A2"
                          # "t1"
                          # "t2"
                          n232 = local read "N pulses per point"() -> (w422:i32)
                          n233 = local read "Repeat each point"() -> (w421:i64)
                          n234 = local read "N samples/decay min"() -> (w418:i32)
                          n235 = Multiply(x=w421, y=w422) -> (x*y=w420:i64)
                          n236 = call "AnalyDecayPhosphoAndSystem.vi"("Scan rate (Hz)"=w439, "Raw Data Image"=w419, "N pulses"=w420, "Skip samples"="Skip samples", "Last samples"="Last samples", "N samples/decay"=w418) -> ("mean and fit"=w427:dbl[][], "amplitude"=w434:dbl, "Tau (us)"=w432:dbl, "Standard error Tau (us)"=w429:dbl, "Area (au)"=w433:dbl)  [unwired: 3 in, 2 out]
                          n237 = Build Array(w429) -> (w392:dbl[])
                          n238 = Build Array(w432) -> (w393:dbl[])
                          n239 = Divide(x=w393, y=w400) -> (x/y=w417:dbl[])
                          n240 = Divide(x=w393, y=w402) -> (x/y=w416:dbl[])
                          n241 = Negate(x=w417) -> (-x=w408:dbl[])
                          n242 = Negate(x=w416) -> (-x=w409:dbl[])
                          n243 = Not Equal?(x=w393, y=0.0 ("indice")) -> (x != y?=w396:bool[])
                          n244 = Exponential(1:w409) -> (0:w415:dbl[])
                          n245 = Exponential(1:w408) -> (0:w414:dbl[])
                          n246 = Boolean To (0,1)(Boolean=w396) -> (0, 1=w395:i16[])
                          n247 = Multiply(x=w415, y=161.37547) -> (x*y=w403:dbl[])
                          n248 = Divide(x=w403, y=w402) -> (x/y=w407:dbl[])
                          n249 = Negate(x=w407) -> (-x=w404:dbl[])
                          n250 = Multiply(x=w414, y=546.54987) -> (x*y=w401:dbl[])
                          n251 = Divide(x=w401, y=w400) -> (x/y=w406:dbl[])
                          n252 = Negate(x=w406) -> (-x=w405:dbl[])
                          n253 = Add(x=w404, y=w405) -> (x+y=w399:dbl[])
                          n254 = Multiply(x=w399, y=w392) -> (x*y=w398:dbl[])
                          n255 = Add(x=w403, y=w401) -> (x+y=w411:dbl[])
                          n256 = Add(x=w411, y=-96.55396) -> (x+y=w394:dbl[])
                          n257 = Multiply(x=w395, y=w394) -> (x*y=w390:dbl[])
                          n258 = Decrement(x=w425) -> (x-1=w424:i32)
                          n259 = Absolute Value(x=w398) -> (abs(x)=w391:dbl[])
                          n260 = call "waitbar.vi"("Number at end of work"=w424, "Current Number"=w426) -> ("Break Computation"=w423:bool)
                          n261 = Index Array(array=w391, index=0 ("indice")) -> (element=w431:dbl)
                          n262 = Index Array(array=w390, index=0 ("indice")) -> (element=w430:dbl)
                          n263 = Bundle("amplitude"=w434, "Area (au)"=w433, "Tau (us)"=w432, w431, w430, "Standard error Tau (us)"=w429) -> (w428:T12)  [unwired: 1 out]
                        }
                        "DataValues" <- w388
                        "All means and fits" <- w387
                        n264 = local read "localTimeData"() -> (w377:timestamp[][])
                        n265 = local read "Total time per point (s)"() -> (w373:dbl)
                        n266 = Array Subset(array=w377, index (col)="Point Number", length (col)=1 ("longueur")) -> (w378:timestamp[][])  [unwired: 2 in]
                        n267 = local read "Repeat each point"() -> (w379:i64)
                        n268 = Divide(x=w373, y=2.0) -> (x/y=w372:dbl)
                        n269 = Reshape Array(w378, w379) -> (w381:timestamp[])
                        n270 = To Double Precision Float(number=w381) -> (double precision float=w376:dbl[])
                        n271 = Add(x=w376, y=w372) -> (x+y=w374:dbl[])
                        n272 = call-poly <vilib>:"Mean.vi"("X"=w374) -> ("mean"=w375:dbl)  [unwired: 1 out]
                        n273 = To Time Stamp(1:w375) -> (0:w382:timestamp)
                        n274 = local write "Acquisition Time"(w382) -> ()
                        n275 = local read "Point Number"() -> (w370:i32)
                        n276 = Index Array(array=w387, index (dim 0)=w370) -> (element=→"Average fit":dbl[][])  [unwired: 2 in]
                        n277 = Build Array(w370) -> (w386:i32[])
                        n278 = property on="DataValues" class="Arr (strict)"("Index Values"=w386) -> ()  [unwired: 2 in, 2 out]
                      }
                      frame True {
                        n279 = local read "Point Number"() -> (w451:i32)
                        n280 = local read "localTimeData"() -> (w447:timestamp[][])
                        n281 = local read "All means and fits"() -> (w457:dbl[][][])
                        n282 = local read "Point Number"() -> (w454:i32)
                        n283 = Array Subset(array=w447, index (col)=w451, length (col)=1 ("longueur")) -> (w448:timestamp[][])  [unwired: 2 in]
                        n284 = Index Array(array=w457, index (dim 0)=w454) -> (element=w456:dbl[][])  [unwired: 2 in]
                        n285 = Build Array(w454) -> (w455:i32[])
                        n286 = local read "Repeat each point"() -> (w449:i64)
                        n287 = local write "Average fit"(w456) -> ()
                        n288 = property on="DataValues" class="Arr (strict)"("Index Values"=w455) -> ()  [unwired: 2 in, 2 out]
                        n289 = local read "Total time per point (s)"() -> (w443:dbl)
                        n290 = Reshape Array(w448, w449) -> (w452:timestamp[])
                        n291 = To Double Precision Float(number=w452) -> (double precision float=w446:dbl[])
                        n292 = local write "Not NewlyAcquired"(FALSE ("Not NewlyAcquired")) -> ()
                        n293 = call-poly <vilib>:"Mean.vi"("X"=w446) -> ("mean"=w445:dbl)  [unwired: 1 out]
                        n294 = Divide(x=w443, y=2.0) -> (x/y=w440:dbl)
                        n295 = Add(x=w440, y=w445) -> (x+y=w441:dbl)
                        n296 = To Time Stamp(1:w441) -> (0:→"Acquisition Time":timestamp)
                      }
                    }
                  }
                  frame #1 {
                    # "Turn off analysis for future iteration"
                    n297 = local write "Analyse"(FALSE ("Analyse")) -> ()
                  }
                }
              }
            }
          }
          frame #3 {
            # "Analyse Pulse amplitude to extract RBC flow"
            n298 = local read "Analyse EAT"() -> (w462:bool)
            n299 = Or(x="Analyse RBCs Flow", y=w462) -> (x .or. y?=w461:bool)
            n300 = local read "Analyse PO2 RBC/InterRBC"() -> (w459:bool)
            n301 = Or(x=w461, y=w459) -> (x .or. y?=w460:bool)
            n302 = case shown="True" w460 {
              tunnel: w465 -> [_ w467]
              tunnel: w464 -> [_ w466]
              frame False {
              }
              frame True {
                n303 = stacked-sequence {
                  seq-local: [_ w474 _ _ _ _ _ _] -> [_ _ w533 _ w645 w704 _ _]
                  seq-local: [_ w475 _ _ _ _ _ _] -> [_ _ w537 _ _ _ _ _]
                  seq-local: [_ w473 _ _ _ _ _ _] -> [_ _ _ _ w634 _ _ _]
                  seq-local: [_ _ w534 _ _ _ _ _] -> [_ _ _ _ w647 _ _ _]
                  seq-local: [_ _ w574 _ _ _ _ _] -> [_ _ _ _ _ _ _ _]
                  seq-local: [_ _ w529 _ _ _ _ _] -> [_ _ _ _ _ w694 _ _]
                  seq-local: [_ _ _ _ _ w698 _ _] -> [_ _ _ _ _ _ _ _]
                  seq-local: [_ _ _ _ _ w696 _ _] -> [_ _ _ _ _ _ _ _]
                  seq-local: [_ _ _ _ _ w697 _ _] -> [_ _ _ _ _ _ _ _]
                  seq-local: [_ _ _ _ _ w695 _ _] -> [_ _ _ _ _ _ _ _]
                  seq-local: [_ _ w555 _ _ _ _ _] -> [_ _ _ _ _ w693 _ _]
                  seq-local: [_ _ w553 _ _ _ _ _] -> [_ _ _ _ _ w699 _ _]
                  seq-local: [_ w485 _ _ _ _ _ _] -> [_ _ _ _ _ w705 _ w991]
                  seq-local: [_ _ _ _ _ w703 _ _] -> [_ _ _ _ _ _ w907 _]
                  seq-local: [_ _ _ _ _ w702 _ _] -> [_ _ _ _ _ _ w908 _]
                  seq-local: [_ _ _ _ _ w700 _ _] -> [_ _ _ _ _ _ w906 _]
                  seq-local: [_ _ _ _ _ w701 _ _] -> [_ _ _ _ _ _ w905 _]
                  seq-local: [_ _ _ _ _ w692 _ _] -> [_ _ _ _ _ _ _ w990]
                  tunnel: w467 -> [_ _ _ _ _ _ w904 w992]
                  tunnel: w466 -> [_ w476 _ _ _ _ _ w988]
                  frame #0 {
                    w468 = u16 1 items=["1", "2"] ("Channel Analysed")
                    n304 = local write "Channel Analysed RBC Flow"(w468) -> ()
                    n305 = local write "Analyse RBCs Flow"(FALSE ("Analyse amplitude pulse")) -> ()
                  }
                  frame #1 {
                    # "Filter pulse amplitude with a sliding averaging filter and reduce to 1D"
                    # "Image part"
                    # "Laser pulse"
                    # "Extract the pulse amplitude from raw data"
                    n306 = local read "N pulses per point"() -> (w478:i32)
                    n307 = local read "Repeat each point"() -> (w497:i64)
                    n308 = Divide(x=w476, y=1000000.0) -> (x/y=w473:dbl)
                    n309 = local read "Total time per point (s)"() -> (w495:dbl)
                    n310 = Multiply(x=w497, y=w478) -> (x*y=w492:i64)
                    n311 = Divide(x="from time (s)", y=w495) -> (x/y=w494:dbl)
                    n312 = Divide(x="to time (s)", y=w495) -> (x/y=w493:dbl)
                    n313 = Multiply(x=w494, y=w492) -> (x*y=w490:dbl)
                    n314 = Multiply(x=w493, y=w492) -> (x*y=w491:dbl)
                    n315 = To Long Integer(number=w490) -> (32bit integer=w488:i32)
                    n316 = To Long Integer(number=w491) -> (32bit integer=w487:i32)
                    n317 = local read "N samples/decay min"() -> (w484:i32)
                    n318 = local read "Channel Analysed RBC Flow"() -> (w500:u16)
                    n319 = local read "Raw Data Image"() -> (w510:T3[][])
                    n320 = local read "Point Number"() -> (w501:i32)
                    n321 = Decrement(x=37.0) -> (x-1=w489:dbl)
                    n322 = Decrement(x=3.0) -> (x-1=w509:dbl)
                    n323 = Index Array(array=w510, index (row)=w500, index (col)=w501) -> (element=w499:T3)
                    n324 = Divide(x=3.0, y=2000.0) -> (x/y=w505:dbl)
                    n325 = Build Array(w509, w488, w489, w487) -> (w503:dbl[])
                    n326 = Build Array(0 ("element"), w488, w484, w487) -> (w485:i32[])
                    n327 = Divide(x=w505, y=w473) -> (x/y=w504:dbl)
                    n328 = Round Toward -Infinity(1:w504) -> (0:w483:dbl)
                    n329 = call "IMAQ ImageToArray"("Optional Rectangle"=w503, "Image"=w499) -> ("Image Pixels (I16)"=w502:i16[][])  [unwired: 1 in, 5 out]
                    n330 = To Long Integer(number=w483) -> (32bit integer=w480:i32)
                    n331 = Array Size(array=w502) -> (size(s)=w508:i32[])
                    n332 = Multiply(x=w480, y=2) -> (x*y=w481:i32)
                    n333 = Index Array(array=w508, index=0 ("indice")) -> (element=w474:i32)
                    n334 = Increment(x=w481) -> (x+1=w479:i32)
                    n335 = for {
                      N: w474 -> [_]
                      tunnel: w502 -> [w521]
                      tunnel: [w517] -> w475 mode=indexing
                      tunnel: w480 -> [w512]
                      tunnel: w479 -> [w511]
                      i -> [w513]
                      n336 = Subtract(x=w513, y=w512) -> (x-y=w520:i32)
                      n337 = Array Subset(array=w521, index (row)=w520, length (row)=w511) -> (w516:i16[][])  [unwired: 2 in]
                      n338 = To Long Integer(number=w516) -> (32bit integer=w518:i32[][])
                      n339 = Array Size(array=w516) -> (size(s)=w515:i32[])
                      n340 = Add Array Elements(numeric array=w518) -> (sum=w519:i32)
                      n341 = Multiply Array Elements(1:w515) -> (0:w514:i32)
                      n342 = Divide(x=w519, y=w514) -> (x/y=w517:dbl)
                    }
                  }
                  frame #2 {
                    w552 = T8 0 items=["Grayscale (U8)", "Grayscale (I16)", "Grayscale (SGL)", "Complex (CSG)", "RGB (U32)", "HSL (U32)", "RGB (U64)", "Grayscale (U16)"] ("Image Type")
                    w562 = T8 0 items=["Grayscale (U8)", "Grayscale (I16)", "Grayscale (SGL)", "Complex (CSG)", "RGB (U32)", "HSL (U32)", "RGB (U64)", "Grayscale (U16)"] ("Image Type")
                    w578 = T8 1 items=["Grayscale (U8)", "Grayscale (I16)", "Grayscale (SGL)", "Complex (CSG)", "RGB (U32)", "HSL (U32)", "RGB (U64)", "Grayscale (U16)"] ("Image Type")
                    w592 = u32 0 items=["8 bits", "16 bits", "Float", "Complex", "RGB", "HSL"] ("Image Type")
                    w597 = T8 1 items=["Grayscale (U8)", "Grayscale (I16)", "Grayscale (SGL)", "Complex (CSG)", "RGB (U32)", "HSL (U32)", "RGB (U64)", "Grayscale (U16)"] ("Image Type")
                    w599 = T8 0 items=["Grayscale (U8)", "Grayscale (I16)", "Grayscale (SGL)", "Complex (CSG)", "RGB (U32)", "HSL (U32)", "RGB (U64)", "Grayscale (U16)"] ("Image Type")
                    # "7. Label image"
                    # "4. Morph"
                    # "3. Threshold"
                    # "2. Negative"
                    # "1. Convert"
                    # "6. Distance outside RBCs"
                    # "5. Distance inside RBCs"
                    # "Convert 0s to 1s and viceversa"
                    # "Extract distribution of distance to RBCs border"
                    # "Count RBCs"
                    n343 = call "IMAQ Create"("Border Size"=3, "Image Name"="Distance MAP", "Image Type"=w562) -> ("New Image"=w561:T3)  [unwired: 1 in, 2 out]
                    n344 = call "IMAQ Create"("Border Size"=3, "Image Name"="Binarized RBCs", "Image Type"=w599) -> ("New Image"=w589:T3)  [unwired: 1 in, 2 out]
                    n345 = call "IMAQ Create"("Border Size"=3, "Image Name"="Raw RBCs", "Image Type"=w597) -> ("New Image"=w594:T3)  [unwired: 1 in, 2 out]
                    n346 = Build Array(w537) -> (w598:dbl[][])
                    n347 = call "IMAQ Create"("Border Size"=3, "Image Name"="Counted RBCs", "Image Type"=w578) -> ("New Image"=w575:T3)  [unwired: 1 in, 2 out]
                    n348 = Transpose 2D Array(2D array=w598) -> (transposed array=w593:dbl[][])
                    n349 = call "IMAQ Create"("Border Size"=3, "Image Name"="Distance MAP INSIDE RBCs", "Image Type"=w552) -> ("New Image"=w549:T3)  [unwired: 1 in, 2 out]
                    n350 = call "IMAQ ArrayToImage"("Image Pixels (I16)"=w593, "Image"=w594) -> ("Image Out"=w590:T3)  [unwired: 4 in, 5 out]
                    n351 = call "IMAQ Cast Image"("Image Type"=w592, "# Shifts"=4, "Image Dst"=w589, "Image Src"=w590) -> ("Image Dst Out"=w572:T3)  [unwired: 2 in, 5 out]
                    n352 = call "IMAQ Inverse"("Image Src"=w572) -> ("Image Dst Out"=w573:T3)  [unwired: 3 in, 7 out]
                    n353 = call "IMAQ AutoMThreshold"("Number of Classes"=2, "Image"=w573) -> ("Threshold Data out"=w588:T13)  [unwired: 2 in, 2 out]
                    n354 = Initialize Array(1 ("Border Size"), 3 ("dimension size"), 1 ("taille de la dimension")) -> (w566:i32[][])
                    n355 = call "IMAQ MultiThreshold"("Threshold Data"=w588, "Image Src"=w573) -> ("Image Dst Out"=w585:T3)  [unwired: 2 in, 2 out]
                    n356 = call "IMAQ Morphology"("Number of iterations (1)"=3, "Structuring Element"=w566, "Operation"=T7."Erode", "Image Src"=w585) -> ("Image Dst Out"=w582:T3)  [unwired: 3 in, 4 out]
                    n357 = Initialize Array(1 ("Border Size"), 3 ("dimension size"), 1 ("taille de la dimension")) -> (w544:i32[][])
                    n358 = call "IMAQ Morphology"("Number of iterations (1)"=3, "Structuring Element"=w544, "Operation"=T7."Dilate", "Image Src"=w582) -> ("Image Dst Out"=w568:T3)  [unwired: 3 in, 4 out]
                    n359 = Array Max & Min(array=w537) -> (max value=w581:dbl, min value=w580:dbl)  [unwired: 2 out]
                    n360 = Initialize Array(1 ("Border Size"), 3 ("dimension size"), 1 ("taille de la dimension")) -> (w541:i32[][])
                    n361 = Subtract(x=w581, y=w580) -> (x-y=w579:dbl)
                    n362 = call "IMAQ Morphology"("Number of iterations (1)"=3, "Structuring Element"=w541, "Operation"=T7."Dilate", "Image Src"=w568) -> ("Image Dst Out"=w567:T3)  [unwired: 3 in, 4 out]
                    n363 = Initialize Array(1 ("Border Size"), 3 ("dimension size"), 1 ("taille de la dimension")) -> (w531:i32[][])
                    n364 = call "IMAQ Morphology"("Number of iterations (1)"=3, "Structuring Element"=w531, "Operation"=T7."Erode", "Image Src"=w567) -> ("Image Dst Out"=w556:T3)  [unwired: 3 in, 4 out]
                    n365 = call "IMAQ Copy"("Image Dst"=w561, "Image Src"=w556) -> ("error out"=w548:errorcluster, "Image Dst Out"=w554:T3)  [unwired: 1 in, 3 out]
                    n366 = call "IMAQ Danielsson"("error in (no error)"=w548, "Image Dst"=w549, "Image Src"=w554) -> ("error out"=w547:errorcluster, "Image Dst Out"=w553:T3)  [unwired: 1 out]
                    n367 = call "IMAQ ImageToArray"("error in (no error)"=w547, "Image"=w554) -> ("Image Pixels (U8)"=w560:u8[][])  [unwired: 1 in, 5 out]
                    n368 = Increment(x=w560) -> (x+1=w559:u8[][])
                    n369 = Reciprocal(x=w559) -> (1/x=w558:dbl[][])
                    n370 = call "IMAQ Label"("Image Dst"=w575, "Image Src"=w556) -> ("Number of Particles"=w574:i32, "Image Dst Out"=w534:T3)  [unwired: 2 in, 1 out]
                    n371 = Round Toward -Infinity(1:w558) -> (0:w532:dbl[][])
                    n372 = call "IMAQ ImageToArray"("Image"=w556) -> ("Image Pixels (U8)"=w535:u8[][])  [unwired: 2 in, 5 out]
                    n373 = call "IMAQ ArrayToImage"("Image Pixels (U8)"=w532, "Image"=w554) -> ("Image Out"=w557:T3)  [unwired: 4 in, 5 out]
                    n374 = Reshape Array(w535, w533) -> (w529:u8[])
                    "Cells detect" <- w529
                    n375 = call "IMAQ Danielsson"("Image Src"=w557) -> ("Image Dst Out"=w555:T3)  [unwired: 2 in, 2 out]
                    n376 = Multiply(x=w579, y=w529) -> (x*y=w586:dbl[])
                    n377 = Add(x=w580, y=w586) -> (x+y=w536:dbl[])
                    n378 = Build Array(w537, w536) -> (→"RBC anal Checked":dbl[][])
                  }
                  frame #3 {
                    # "Decays only in Plasma"
                    # "Filter decays Before/After and IN/OUT of cells"
                    n379 = script code="clear all"() -> ("??"=w605:errorcluster)  [unwired: 1 in]
                    n380 = local read "Cells detect"() -> (w604:u8[])
                    n381 = script code="data2 = Data;\ndata1 = double(~Data);\ndist_map1 = bwdist(data1);\ndist_map2 = -bwdist(data2);\ndist_map = dist_map1 + dist_map2;\ndist_map0 = -dist_map;\n\n% OUT OF CELL  ========================================================\nborders = find(dist_map0 == 1);\nOUT_after = zeros(length(dist_map0),1); OUT_before = OUT_after;\nind_before = []; ind_after = []; \nfor i = 1:length(borders) - 1\n\na = borders(i); b = borders(i+1);\nif dist_map0(a+1) < 0\ncontinue\nelse\n%  Search for the maxima\nm = 0; ind_max = [];\nif numel(dist_map0) > 2\n for k = a+1:b-1\n     if dist_map0(k) >= dist_map0(k+1) && dist_map0(k) >= dist_map0(k-1)\n        m = m + 1;\n        ind_max(m) = k;\n     end\n end\nend\n\n% ind_aft = a:ind_max(1) - 1;\n% ind_bef = ind_max(end) + 1:b;\n\nind_aft = a:ind_max(1);\nind_bef = ind_max(end):b;\n\nind_before = [ind_before ind_bef];\nind_after = [ind_after ind_aft];\nend\nend\nOUT_before(ind_before) = 1;\nOUT_after(ind_after) = 1;\n% figure(5), plot(OUT_before)\n\nx = 1:length(dist_map0);\ny = OUT_before;"("??"=w605, "Data"=w604) -> ("OUT_before"=w606:dbl[][], "OUT_after"=w611:dbl[][])  [unwired: 1 out]
                    n382 = Index Array(array=w611, index (col)=0 ("index (row)")) -> (element=w609:dbl[])  [unwired: 1 in]
                    n383 = Index Array(array=w606, index (col)=0 ("index (row)")) -> (element=w608:dbl[])  [unwired: 1 in]
                    n384 = To Long Integer(number=w609) -> (32bit integer=→"RBC_after":i32[])
                    n385 = To Long Integer(number=w608) -> (32bit integer=→"RBC_before":i32[])
                  }
                  frame #4 {
                    w612 = 0.3 ("y")
                    # "Moyenne hematocrite et flux en supprimant le premier et dernier point qui peuvent être faux"
                    # "Extract flow from RBCs shadows"
                    n386 = local read "N pulses per point"() -> (w624:i32)
                    n387 = local read "Repeat each point"() -> (w625:i64)
                    n388 = local read "Total time per point (s)"() -> (w623:dbl)
                    n389 = Multiply(x=w625, y=w624) -> (x*y=w622:i64)
                    n390 = Divide(x=w623, y=w622) -> (x/y=w621:dbl)
                    n391 = Divide(x=w621, y=w634) -> ()  [unwired: 1 out]
                    n392 = property on="RBC anal Checked" class="WFGraph (strict)"("XScale.Multiplier"=w621) -> ()  [unwired: 2 in, 2 out]
                    n393 = call "IMAQ ImageToArray"("Image"=w647) -> ("Image Pixels (I16)"=w636:i16[][])  [unwired: 2 in, 5 out]
                    n394 = Multiply(x=w634, y=w645) -> (x*y=w644:dbl)
                    n395 = Divide(x=w612, y=w634) -> (x/y=w641:dbl)
                    n396 = Divide(x=w644, y=w612) -> (x/y=w643:dbl)
                    n397 = Reshape Array(w636, w645) -> (w635:i16[])
                    n398 = Round Toward -Infinity(1:w641) -> (0:w640:dbl)
                    n399 = Divide(x=w612, y=2.0) -> (x/y=w638:dbl)
                    n400 = Round Toward +Infinity(x=w643) -> (ceil(x): smallest int >= x=w642:dbl)
                    n401 = To Long Integer(number=w640) -> (32bit integer=w639:i32)
                    n402 = for {
                      N: w642 -> [w650]
                      tunnel: w635 -> [w659]
                      shift-right: [w652] -> _
                      shift-left: 1 ("index of element") -> [w654]
                      tunnel: [w671] -> _ mode=indexing
                      shift-right: [w669] -> _
                      shift-left: w638 -> [w671]
                      tunnel: [w672] -> w613 mode=indexing
                      tunnel: w639 -> [w673]
                      tunnel: w612 -> [w670]
                      tunnel: [w661] -> w626 mode=indexing
                      i -> [w651]
                      stop <- w649 stop-if-true
                      # "Extract number of cells per bloc"
                      # "Extract proportion of RBCs"
                      n403 = Decrement(x=w650) -> (x-1=w648:i32)
                      n404 = Multiply(x=w673, y=w651) -> (x*y=w674:i32)
                      n405 = Array Subset(array=w659, index=w674, length=w673) -> (w658:i16[])
                      n406 = Array Max & Min(array=w658) -> (max value=w653:i16)  [unwired: 3 out]
                      n407 = call "waitbar.vi"("Number at end of work"=w648, "Current Number"=w651) -> ("Break Computation"=w649:bool)
                      n408 = Max & Min(x=w653, y=w654) -> (max(x,y)=w652:i32)  [unwired: 1 out]
                      n409 = Subtract(x=w652, y=w654) -> (x-y=w660:i32)
                      n410 = Increment(x=w660) -> (x+1=w655:i32)
                      n411 = for {
                        N: w655 -> [_]
                        tunnel: w659 -> [w678]
                        tunnel: w658 -> [w679]
                        shift-right: [w681] -> w656
                        shift-left: 0.0 -> [w680]
                        tunnel: w654 -> [w683]
                        i -> [w684]
                        n412 = Add(x=w684, y=w683) -> (x+y=w677:i32)
                        n413 = call "OccurDetector.vi"("Indice to find"=w677, "Reference Matrix"=w679) -> ("Number of occurence"=w675:i32)
                        n414 = call "OccurDetector.vi"("Indice to find"=w677, "Reference Matrix"=w678) -> ("Number of occurence"=w676:i32)
                        n415 = Divide(x=w675, y=w676) -> (x/y=w682:dbl)
                        n416 = Add(x=w682, y=w680) -> (x+y=w681:dbl)
                      }
                      n417 = Add(x=w671, y=w670) -> (x+y=w669:dbl)
                      n418 = Array Size(array=w658) -> (size(s)=w663:i32)
                      n419 = Sort 1D Array(array=w658) -> (sorted array=w668:i16[])
                      n420 = Reverse 1D Array(array=w668) -> (reversed array=w667:i16[])
                      n421 = Search 1D Array(1D array=w667, element=i16 0 ("élément")) -> (index of element=w662:i32)  [unwired: 1 out]
                      n422 = Equal?(x=w662, y=-1) -> (x = y?=w664:bool)
                      n423 = case shown="False" w664 {
                        tunnel: w663 -> [w688 _]
                        tunnel: w662 -> [w689 _]
                        tunnel: [w685 100.0 ("y")] -> w661
                        frame False {
                          n424 = Divide(x=w689, y=w688) -> (x/y=w687:dbl)
                          n425 = Multiply(x=w687, y=100.0) -> (x*y=w685:dbl)
                        }
                        frame True {
                        }
                      }
                      n426 = Divide(x=w656, y=w670) -> (x/y=w672:dbl)
                    }
                    n427 = Array Size(array=w613) -> (size(s)=w615:i32)
                    n428 = Array Size(array=w626) -> (size(s)=w628:i32)
                    n429 = Subtract(x=w615, y=2) -> (x-y=w618:i32)
                    n430 = Subtract(x=w628, y=2) -> (x-y=w632:i32)
                    n431 = Array Subset(array=w613, index=1 ("indice"), length=w618) -> (w620:dbl[])
                    n432 = Array Subset(array=w626, index=1 ("indice"), length=w632) -> (w630:dbl[])
                    n433 = Add Array Elements(numeric array=w620) -> (sum=w617:dbl)
                    n434 = Add Array Elements(numeric array=w630) -> (sum=w631:dbl)
                    n435 = Divide(x=w617, y=w618) -> (x/y=→"Mean Flow":dbl)
                    n436 = Divide(x=w631, y=w632) -> (x/y=→"Mean Hematocrit":dbl)
                  }
                  frame #5 {
                    w714 = T8 1 items=["Grayscale (U8)", "Grayscale (I16)", "Grayscale (SGL)", "Complex (CSG)", "RGB (U32)", "HSL (U32)", "RGB (U64)", "Grayscale (U16)"] ("Image Type")
                    w709 = T8 1 items=["Grayscale (U8)", "Grayscale (I16)", "Grayscale (SGL)", "Complex (CSG)", "RGB (U32)", "HSL (U32)", "RGB (U64)", "Grayscale (U16)"] ("Image Type")
                    w723 = T8 1 items=["Grayscale (U8)", "Grayscale (I16)", "Grayscale (SGL)", "Complex (CSG)", "RGB (U32)", "HSL (U32)", "RGB (U64)", "Grayscale (U16)"] ("Image Type")
                    w728 = T8 1 items=["Grayscale (U8)", "Grayscale (I16)", "Grayscale (SGL)", "Complex (CSG)", "RGB (U32)", "HSL (U32)", "RGB (U64)", "Grayscale (U16)"] ("Image Type")
                    # "matrice1"
                    # "outside all (partie0)"
                    # "matrice2"
                    n437 = call "IMAQ Create"("Border Size"=3, "Image Name"="matrice1", "Image Type"=w709) -> ("New Image"=w708:T3)  [unwired: 1 in, 2 out]
                    n438 = call "IMAQ Create"("Border Size"=3, "Image Name"="matrice2", "Image Type"=w714) -> ("New Image"=w707:T3)  [unwired: 1 in, 2 out]
                    n439 = local read "Raw Data Image"() -> (w729:T3[][])
                    n440 = call "IMAQ Create"("Border Size"=3, "Image Name"="RBCmatrix", "Image Type"=w728) -> ("New Image"=w717:T3)  [unwired: 1 in, 2 out]
                    n441 = call "IMAQ Create"("Border Size"=3, "Image Name"="Non-RBCmatrix", "Image Type"=w723) -> ("New Image"=w716:T3)  [unwired: 1 in, 2 out]
                    n442 = local read "Channel analysed for EAT"() -> (w720:u16)
                    n443 = local read "Point Analysed"() -> (w706:i32)
                    n444 = Index Array(array=w729, index (row)=w720, index (col)=w706) -> (element=w719:T3)
                    n445 = call "IMAQ ImageToArray"("Optional Rectangle"=w705, "Image"=w719) -> ("Image Pixels (I16)"=w718:i16[][])  [unwired: 1 in, 5 out]
                    n446 = stacked-sequence {
                      seq-local: [w755 _ _ _] -> [_ _ w841 _]
                      seq-local: [w754 _ _ _] -> [_ _ w839 _]
                      seq-local: [w752 _ _ _] -> [_ _ w840 _]
                      seq-local: [w746 _ _ _] -> [_ _ _ w874]
                      seq-local: [w744 _ _ _] -> [_ _ _ w873]
                      seq-local: [w753 _ _ _] -> [_ _ _ w871]
                      seq-local: [w739 _ _ _] -> [_ _ w842 w872]
                      tunnel: w694 -> [_ w803 _ _]
                      tunnel: [_ w802 _ _] -> w722
                      tunnel: [_ w801 _ _] -> w721
                      tunnel: [_ w800 _ _] -> w695
                      tunnel: [_ w799 _ _] -> w697
                      tunnel: w718 -> [_ w798 w847 w879]
                      tunnel: w704 -> [_ w797 w845 w877]
                      tunnel: w693 -> [w771 _ _ _]
                      tunnel: [_ _ w844 _] -> w715
                      tunnel: [_ _ w843 _] -> w703
                      tunnel: [_ _ _ w876] -> w691
                      tunnel: [_ _ _ w875] -> w701
                      tunnel: w699 -> [w770 _ _ _]
                      tunnel: [w739 _ _ _] -> w692
                      frame #0 {
                        # "matrice1"
                        # "from time 1"
                        # "to time 1"
                        # "matrice 2"
                        # "to time 2"
                        # "from time 2"
                        n447 = call "IMAQ ImageToArray"("Image"=w771) -> ("Image Pixels (U8)"=w780:u8[][])  [unwired: 2 in, 5 out]
                        n448 = call "IMAQ ImageToArray"("Image"=w770) -> ("Image Pixels (U8)"=w781:u8[][])  [unwired: 2 in, 5 out]
                        n449 = To Word Integer(number=w780) -> (16bit integer=w779:i16[][])
                        n450 = To Word Integer(number=w781) -> (16bit integer=w774:i16[][])
                        n451 = Array Size(array=w779) -> (size(s)=w782:i32[])
                        n452 = Decrement(x=w774) -> (x-1=w772:i16[][])
                        n453 = local read "Interpulse interval (us)"() -> (w759:dbl)
                        n454 = Multiply Array Elements(1:w782) -> (0:w778:i32)
                        n455 = Reshape Array(w772, w778) -> (w777:i16[])
                        n456 = for {
                          tunnel: w777 -> [w785] mode=indexing
                          tunnel: [w783] -> w776 mode=indexing
                          # "Replace the border to allow 0 elements"
                          n457 = Max & Min(x=w785, y=i16 0) -> (max(x,y)=w783:i16)  [unwired: 1 out]
                        }
                        n458 = Reshape Array(w779, w778) -> (w775:i16[])
                        n459 = Negate(x=w776) -> (-x=w773:i16[])
                        n460 = Add(x=w775, y=w773) -> (x+y=w739:i16[])
                        n461 = Array Max & Min(array=w739) -> (max value=w733:i16, min value=w732:i16)  [unwired: 2 out]
                        n462 = Sort 1D Array(array=w739) -> (sorted array=w749:i16[])
                        n463 = Divide(x=w759, y=1000.0) -> (x/y=w736:dbl)
                        n464 = Multiply(x=w733, y=w736) -> (x*y=w738:dbl)
                        n465 = property on="To time (ms) 1" class="DigNum (strict)"("Maximum"=w738) -> ()  [unwired: 2 in, 2 out]
                        n466 = property on="To time (ms) 2" class="DigNum (strict)"("Maximum"=w738) -> ()  [unwired: 2 in, 2 out]
                        n467 = local write "Max"(w738) -> ()
                        n468 = Multiply(x=w732, y=w736) -> (x*y=w737:dbl)
                        n469 = Divide(x="From time (ms) 2", y=w736) -> (x/y=w752:dbl)
                        n470 = Divide(x="To time (ms) 2", y=w736) -> (x/y=w755:dbl)
                        n471 = Increment(x=w755) -> (x+1=w761:dbl)
                        n472 = Round Toward +Infinity(x=w752) -> (ceil(x): smallest int >= x=w760:dbl)
                        n473 = property on="From time (ms) 2" class="DigNum (strict)"("Minimum"=w737) -> ()  [unwired: 2 in, 2 out]
                        n474 = property on="From time (ms) 1" class="DigNum (strict)"("Minimum"=w737) -> ()  [unwired: 2 in, 2 out]
                        n475 = local write "Min"(w737) -> ()
                        n476 = property on="To time (ms) 2" class="DigNum (strict)"("OutOfRngActMax"=u8 1 ("Response to Value Outside Limits:Maximum")) -> ()  [unwired: 2 in, 2 out]
                        n477 = Round Toward -Infinity(1:w761) -> (0:w735:dbl)
                        n478 = In Range and Coerce(upper limit=w733, x=w735, lower limit=w732) -> (coerced(x)=w734:dbl)  [unwired: 1 out]
                        n479 = Search 1D Array(1D array=w749, element=w760) -> (index of element=w762:i32)  [unwired: 1 out]
                        n480 = Search 1D Array(1D array=w749, element=w734) -> (index of element=w766:i32)  [unwired: 1 out]
                        n481 = property on="From time (ms) 2" class="DigNum (strict)"("OutOfRngActMin"=u8 1 ("Response to Value Outside Limits:Minimum")) -> ()  [unwired: 2 in, 2 out]
                        n482 = Subtract(x=w766, y=w762) -> (x-y=w764:i32)
                        n483 = Divide(x="To time (ms) 1", y=w736) -> (x/y=w746:dbl)
                        n484 = Divide(x="From time (ms) 1", y=w736) -> (x/y=w745:dbl)
                        n485 = local read "N samples/decay min"() -> (w763:i32)
                        n486 = Initialize Array(i16 0 ("élément"), w764, w763) -> (w754:i16[][])
                        n487 = Round Toward +Infinity(x=w745) -> (ceil(x): smallest int >= x=w744:dbl)
                        n488 = Increment(x=w746) -> (x+1=w750:dbl)
                        n489 = Round Toward -Infinity(1:w750) -> (0:w731:dbl)
                        n490 = In Range and Coerce(upper limit=w733, x=w731, lower limit=w732) -> (coerced(x)=w730:dbl)  [unwired: 1 out]
                        n491 = property on="To time (ms) 1" class="DigNum (strict)"("OutOfRngActMax"=u8 1 ("Response to Value Outside Limits:Maximum")) -> ()  [unwired: 2 in, 2 out]
                        n492 = property on="From time (ms) 1" class="DigNum (strict)"("OutOfRngActMin"=u8 1 ("Response to Value Outside Limits:Minimum")) -> ()  [unwired: 2 in, 2 out]
                        n493 = Search 1D Array(1D array=w749, element=w744) -> (index of element=w742:i32)  [unwired: 1 out]
                        n494 = Search 1D Array(1D array=w749, element=w730) -> (index of element=w743:i32)  [unwired: 1 out]
                        n495 = Subtract(x=w743, y=w742) -> (x-y=w751:i32)
                        n496 = Initialize Array(i16 0 ("élément"), w751, w763) -> (w753:i16[][])
                      }
                      frame #1 {
                        # "Number of 1"
                        # "Number of 0"
                        n497 = local read "N samples/decay min"() -> (w786:i32)
                        n498 = Sort 1D Array(array=w803) -> (sorted array=w794:u8[])
                        n499 = Search 1D Array(1D array=w794, element=u8 1 ("élément")) -> (index of element=w788:i32)  [unwired: 1 out]
                        n500 = Subtract(x=w797, y=w788) -> (x-y=w787:i32)
                        n501 = Initialize Array(i16 0 ("élément"), w788, w786) -> (w791:i16[][])
                        n502 = Initialize Array(i16 0 ("élément"), w787, w786) -> (w789:i16[][])
                        n503 = for {
                          N: w797 -> [_]
                          tunnel: w803 -> [w820] mode=indexing
                          tunnel: w798 -> [w817]
                          shift-right: [w807] -> w801
                          shift-left: w791 -> [w814]
                          shift-right: [w812] -> w802
                          shift-left: w789 -> [w813]
                          shift-right: [w809] -> w800
                          shift-left: 0 -> [w811]
                          shift-right: [w808] -> w799
                          shift-left: 0 -> [w810]
                          tunnel: w786 -> [w804]
                          i -> [w806]
                          # "select decay  inside and outside RBCs"
                          n504 = Array Subset(array=w817, index (row)=w806, length (row)=1 ("longueur")) -> (w816:i16[][])  [unwired: 2 in]
                          n505 = Equal?(x=0, y=w820) -> (x = y?=w818:bool)
                          n506 = Reshape Array(w816, w804) -> (w815:i16[])
                          n507 = case shown="True" w818 {
                            tunnel: w815 -> [w825 w833]
                            tunnel: w814 -> [w829 w834]
                            tunnel: [w829 w835] -> w807
                            tunnel: w813 -> [w826 w838]
                            tunnel: [w824 w838] -> w812
                            tunnel: w811 -> [w827 w830]
                            tunnel: w810 -> [w822 w836]
                            tunnel: [w827 w837] -> w809
                            tunnel: [w828 w836] -> w808
                            frame False {
                              # "Add line to RBC matrix"
                              n508 = Build Array(w825) -> (w823:i16[][])
                              n509 = Increment(x=w822) -> (x+1=w828:i32)
                              n510 = Replace Array Subset(array=w826, new element=w823, index (row)=w822, index (col)=0 ("indice désactivé (col)")) -> (w824:i16[][])
                            }
                            frame True {
                              # "Add line to non-RBC matrix"
                              n511 = Build Array(w833) -> (w832:i16[][])
                              n512 = Increment(x=w830) -> (x+1=w837:i32)
                              n513 = Replace Array Subset(array=w834, new element=w832, index (row)=w830, index (col)=0 ("indice désactivé (col)")) -> (w835:i16[][])
                            }
                          }
                        }
                      }
                      frame #2 {
                        # "matrice2"
                        # "matrice1"
                        # "matrice2"
                        # "matrice1"
                        n514 = for {
                          N: w845 -> [_]
                          shift-right: [w854] -> w843
                          shift-left: 0 -> [w855]
                          tunnel: w847 -> [w853]
                          shift-right: [w851] -> w844
                          shift-left: w839 -> [w852]
                          tunnel: w842 -> [w848] mode=indexing
                          tunnel: w841 -> [w850]
                          tunnel: w840 -> [w849]
                          i -> [w858]
                          n515 = In Range and Coerce(upper limit=w850, x=w848, lower limit=w849) -> (In Range?=w857:bool)  [unwired: 1 out]
                          n516 = Array Subset(array=w853, index (row)=w858, length (row)=1 ("longueur")) -> (w861:i16[][])  [unwired: 2 in]
                          n517 = local read "N samples/decay min"() -> (w860:i32)
                          n518 = Reshape Array(w861, w860) -> (w856:i16[])
                          n519 = case shown="True" w857 {
                            tunnel: w856 -> [_ w868]
                            tunnel: w855 -> [w862 w866]
                            tunnel: [w862 w867] -> w854
                            tunnel: w852 -> [w863 w865]
                            tunnel: [w863 w864] -> w851
                            frame False {
                            }
                            frame True {
                              # "Add line to matrice2"
                              n520 = Build Array(w868) -> (w870:i16[][])
                              n521 = Increment(x=w866) -> (x+1=w867:i32)
                              n522 = Replace Array Subset(array=w865, new element=w870, index (row)=w866, index (col)=0 ("indice désactivé (col)")) -> (w864:i16[][])
                            }
                          }
                        }
                      }
                      frame #3 {
                        # "matrice1"
                        # "matrice1"
                        # "matrice1"
                        # "matrice1"
                        n523 = for {
                          N: w877 -> [_]
                          shift-right: [w887] -> w875
                          shift-left: 0 -> [w888]
                          shift-right: [w885] -> w876
                          shift-left: w871 -> [w886]
                          tunnel: w879 -> [w884]
                          tunnel: w874 -> [w883]
                          tunnel: w873 -> [w882]
                          tunnel: w872 -> [w881] mode=indexing
                          i -> [w890]
                          n524 = In Range and Coerce(upper limit=w883, x=w881, lower limit=w882) -> (In Range?=w880:bool)  [unwired: 1 out]
                          n525 = Array Subset(array=w884, index (row)=w890, length (row)=1 ("longueur")) -> (w893:i16[][])  [unwired: 2 in]
                          n526 = local read "N samples/decay min"() -> (w892:i32)
                          n527 = Reshape Array(w893, w892) -> (w889:i16[])
                          n528 = case shown="True" w880 {
                            tunnel: w889 -> [_ w902]
                            tunnel: w886 -> [w895 w896]
                            tunnel: w888 -> [w894 w898]
                            tunnel: [w895 w899] -> w885
                            tunnel: [w894 w897] -> w887
                            frame False {
                            }
                            frame True {
                              # "Add line to matrice1 matrix"
                              n529 = Build Array(w902) -> (w901:i16[][])
                              n530 = Increment(x=w898) -> (x+1=w897:i32)
                              n531 = Replace Array Subset(array=w896, new element=w901, index (row)=w898, index (col)=0 ("indice désactivé (col)")) -> (w899:i16[][])
                            }
                          }
                        }
                      }
                    }
                    n532 = call "IMAQ ArrayToImage"("Image Pixels (I16)"=w715, "Image"=w707) -> ("Image Out"=w702:T3)  [unwired: 4 in, 5 out]
                    n533 = call "IMAQ ArrayToImage"("Image Pixels (I16)"=w691, "Image"=w708) -> ("Image Out"=w700:T3)  [unwired: 4 in, 5 out]
                    n534 = call "IMAQ ArrayToImage"("Image Pixels (I16)"=w722, "Image"=w717) -> ("Image Out"=w698:T3)  [unwired: 4 in, 5 out]
                    n535 = call "IMAQ ArrayToImage"("Image Pixels (I16)"=w721, "Image"=w716) -> ("Image Out"=w696:T3)  [unwired: 4 in, 5 out]
                  }
                  frame #6 {
                    n536 = local read "Analyse PO2 RBC/InterRBC"() -> (w903:bool)
                    n537 = case shown="True" w903 {
                      tunnel: w908 -> [_ w987]
                      tunnel: w907 -> [_ w986]
                      tunnel: w906 -> [_ w985]
                      tunnel: w905 -> [_ w984]
                      tunnel: w904 -> [_ w983]
                      frame False {
                      }
                      frame True {
                        w916 = 7.11341 ("y")
                        w918 = 90.47064 ("y")
                        w940 = 7.11341 ("y")
                        w942 = 90.47064 ("y")
                        # "y0"
                        # "A1"
                        # "A2"
                        # "t1"
                        # "t2"
                        # "65 kDa version of the oxygen dye Jan 2011 - new calib-curve\n(Jun 2012)"
                        # "y0"
                        # "A1"
                        # "A2"
                        # "t1"
                        # "t2"
                        # "Analyse PO2 over 2 time periods"
                        n538 = Multiply(x=w983, y=1000.0) -> (x*y=w975:dbl)
                        n539 = local read "Skip samples"() -> (w981:i32)
                        n540 = local read "Last samples"() -> (w980:i32)
                        n541 = local read "N samples/decay min"() -> (w982:i32)
                        n542 = local read "Last samples"() -> (w979:i32)
                        n543 = local read "N samples/decay min"() -> (w977:i32)
                        n544 = local read "Skip samples"() -> (w978:i32)
                        n545 = local write "Analyse PO2 RBC/InterRBC"(FALSE ("Analyse PO2 over 2 time periods")) -> ()
                        n546 = call "AnalyDecayPhosphoAndSystem.vi"("Scan rate (Hz)"=w975, "Raw Data Image"=w985, "N pulses"=w984, "Skip samples"=w981, "Last samples"=w980, "N samples/decay"=w982) -> ("mean and fit"=w960:dbl[][], "amplitude"=→"Amplitude 1":dbl, "Tau (us)"=w962:dbl, "Standard error Tau (us)"=w911:dbl)  [unwired: 3 in, 3 out]
                        "Tau 1 (us)" <- w962
                        "Std Tau 1" <- w911
                        "Average fit 2" <- w960
                        n547 = call "AnalyDecayPhosphoAndSystem.vi"("Scan rate (Hz)"=w975, "Raw Data Image"=w987, "N pulses"=w986, "Skip samples"=w978, "Last samples"=w979, "N samples/decay"=w977) -> ("mean and fit"=w959:dbl[][], "amplitude"=→"Amplitude 2":dbl, "Tau (us)"=w972:dbl, "Standard error Tau (us)"=w971:dbl)  [unwired: 6 out]
                        "Tau 2 (us)" <- w972
                        "Std Tau 2" <- w971
                        "Average fit  3" <- w959
                        n548 = Build Array (concatenate)(w960, w959) -> (→"Average fit 1/2":dbl[][])
                        n549 = Build Array(w972) -> (w935:dbl[])
                        n550 = Build Array(w971) -> (w936:dbl[])
                        n551 = Build Array(w962) -> (w913:dbl[])
                        n552 = Build Array(w911) -> (w910:dbl[])
                        n553 = Divide(x=w913, y=w916) -> (x/y=w933:dbl[])
                        n554 = Divide(x=w913, y=w918) -> (x/y=w932:dbl[])
                        n555 = Divide(x=w935, y=w940) -> (x/y=w957:dbl[])
                        n556 = Divide(x=w935, y=w942) -> (x/y=w956:dbl[])
                        n557 = Negate(x=w933) -> (-x=w924:dbl[])
                        n558 = Negate(x=w932) -> (-x=w925:dbl[])
                        n559 = Negate(x=w957) -> (-x=w948:dbl[])
                        n560 = Negate(x=w956) -> (-x=w949:dbl[])
                        n561 = Exponential(1:w925) -> (0:w931:dbl[])
                        n562 = Exponential(1:w924) -> (0:w930:dbl[])
                        n563 = Exponential(1:w949) -> (0:w955:dbl[])
                        n564 = Exponential(1:w948) -> (0:w954:dbl[])
                        n565 = Multiply(x=w931, y=161.37547) -> (x*y=w919:dbl[])
                        n566 = Divide(x=w919, y=w918) -> (x/y=w923:dbl[])
                        n567 = Negate(x=w923) -> (-x=w920:dbl[])
                        n568 = Multiply(x=w930, y=546.54987) -> (x*y=w917:dbl[])
                        n569 = Divide(x=w917, y=w916) -> (x/y=w922:dbl[])
                        n570 = Negate(x=w922) -> (-x=w921:dbl[])
                        n571 = Add(x=w920, y=w921) -> (x+y=w915:dbl[])
                        n572 = Multiply(x=w955, y=161.37547) -> (x*y=w943:dbl[])
                        n573 = Divide(x=w943, y=w942) -> (x/y=w947:dbl[])
                        n574 = Negate(x=w947) -> (-x=w944:dbl[])
                        n575 = Multiply(x=w954, y=546.54987) -> (x*y=w941:dbl[])
                        n576 = Divide(x=w941, y=w940) -> (x/y=w946:dbl[])
                        n577 = Negate(x=w946) -> (-x=w945:dbl[])
                        n578 = Add(x=w944, y=w945) -> (x+y=w939:dbl[])
                        n579 = Multiply(x=w915, y=w910) -> (x*y=w914:dbl[])
                        n580 = Multiply(x=w939, y=w936) -> (x*y=w938:dbl[])
                        n581 = Add(x=w919, y=w917) -> (x+y=w927:dbl[])
                        n582 = Add(x=w927, y=-96.55396) -> (x+y=w912:dbl[])
                        n583 = Add(x=w943, y=w941) -> (x+y=w951:dbl[])
                        n584 = Add(x=w951, y=-96.55396) -> (x+y=w937:dbl[])
                        n585 = Absolute Value(x=w914) -> (abs(x)=w909:dbl[])
                        n586 = Absolute Value(x=w938) -> (abs(x)=w934:dbl[])
                        n587 = Index Array(array=w912, index=0 ("indice")) -> (element=→"pO2 (1)":dbl)
                        n588 = Index Array(array=w909, index=0 ("indice")) -> (element=→"Std pO2 (1)":dbl)
                        n589 = Index Array(array=w937, index=0 ("indice")) -> (element=→"pO2 (2)":dbl)
                        n590 = Index Array(array=w934, index=0 ("indice")) -> (element=→"Std pO2 (2)":dbl)
                        "Number of decays 1" <- w984
                        "Number of decays 2" <- w986
                      }
                    }
                  }
                  frame #7 {
                    n591 = local read "Analyse EAT"() -> (w989:bool)
                    n592 = case shown="True" w989 {
                      tunnel: w992 -> [_ w998]
                      tunnel: w991 -> [_ w1058]
                      tunnel: w990 -> [_ w1057]
                      tunnel: w988 -> [_ w999]
                      frame False {
                      }
                      frame True {
                        w1011 = -3.0 ("x")
                        w1043 = T8 1 items=["Grayscale (U8)", "Grayscale (I16)", "Grayscale (SGL)", "Complex (CSG)", "RGB (U32)", "HSL (U32)", "RGB (U64)", "Grayscale (U16)"] ("Image Type")
                        n593 = local read "Channel analysed for EAT"() -> (w1055:u16)
                        n594 = local read "RBC_before"() -> (w1027:i32[])
                        n595 = local read "RBC before"() -> (w1028:bool)
                        n596 = local read "RBC_after"() -> (w1018:i32[])
                        n597 = local read "Raw Data Image"() -> (w1056:T3[][])
                        n598 = Sort 1D Array(array=w1057) -> (sorted array=w1045:i16[])
                        n599 = local read "Point Analysed"() -> (w1029:i32)
                        "Point EAT" <- w1029
                        n600 = Array Max & Min(array=w1045) -> (max value=w1048:i16, min value=w1049:i16)  [unwired: 2 out]
                        n601 = Select(t=w1027, s=w1028, f=w1018) -> (s? t:f=w1021:i32[])
                        n602 = Subtract(x=w1048, y=w1049) -> (x-y=w1047:i16)
                        n603 = Array Size(array=w1018) -> (size(s)=w1017:i32)
                        n604 = Increment(x=w1048) -> (x+1=w1050:i16)
                        n605 = Increment(x=w1047) -> (x+1=w1046:i16)
                        n606 = call "IMAQ Create"("Border Size"=3, "Image Name"="Local Decays", "Image Type"=w1043) -> ("New Image"=w1040:T3)  [unwired: 1 in, 2 out]
                        n607 = Index Array(array=w1056, index (row)=w1055, index (col)=w1029) -> (element=w1054:T3)
                        n608 = Initialize Array(1 ("y"), w1017) -> (w1016:i32[])
                        n609 = call <vilib>:"General Histogram.vi"("X"=w1045, "max"=w1050, "min"=w1049, "# bins"=w1046) -> ("Histogram"=w1026:i32[], "Axis"=w1044:dbl[])  [unwired: 7 in, 3 out]
                        n610 = Or(x="RBC after", y="RBC before") -> (x .or. y?=w1022:bool)
                        n611 = Subtract(x=w1044, y=0.5) -> (x-y=w1051:dbl[])
                        n612 = call "IMAQ ImageToArray"("Optional Rectangle"=w1058, "Image"=w1054) -> ("Image Pixels (I16)"=w1053:i16[][])  [unwired: 1 in, 5 out]
                        n613 = To Long Integer(number=w1051) -> (32bit integer=w1025:i32[])
                        n614 = Select(t=w1021, s=w1022, f=w1016) -> (s? t:f=w1020:i32[])
                        n615 = for {
                          N -> [w1072]
                          tunnel: w1025 -> [w1075] mode=indexing
                          tunnel: w1057 -> [w1076]
                          tunnel: w1026 -> [w1074] mode=indexing
                          tunnel: w1040 -> [w1070]
                          tunnel: w998 -> [w1069]
                          tunnel: [w1068] -> w1008 mode=indexing
                          tunnel: [w1067] -> w1039 mode=indexing
                          tunnel: [w1066] -> w1038 mode=indexing
                          tunnel: [w1065] -> w1007 mode=indexing
                          tunnel: [w1064] -> w1004 mode=indexing
                          tunnel: [w1063] -> w1033 mode=indexing
                          tunnel: [w1062] -> w1037 mode=indexing
                          tunnel: [w1061] -> w1036 mode=indexing
                          tunnel: w1053 -> [w1060]
                          tunnel: w1020 -> [w1059]
                          i -> [w1073]
                          stop <- w1071 stop-if-true
                          n616 = stacked-sequence {
                            seq-local: [w1080 _ _ _] -> [_ w1085 _ _]
                            seq-local: [_ w1084 _ _] -> [_ _ w1171 _]
                            seq-local: [_ w1083 _ _] -> [_ _ w1142 _]
                            tunnel: w1076 -> [_ w1088 _ _]
                            tunnel: w1075 -> [_ w1087 w1156 _]
                            tunnel: w1074 -> [w1077 _ _ _]
                            tunnel: w1073 -> [_ _ _ w1175]
                            tunnel: w1072 -> [_ _ _ w1174]
                            tunnel: [_ _ _ w1173] -> w1071
                            tunnel: w1070 -> [_ _ w1170 _]
                            tunnel: w1069 -> [_ _ w1164 _]
                            tunnel: [_ _ w1162 _] -> w1068
                            tunnel: [_ _ w1161 _] -> w1067
                            tunnel: [_ _ w1158 _] -> w1066
                            tunnel: [_ _ w1157 _] -> w1065
                            tunnel: [_ _ w1142 _] -> w1064
                            tunnel: [_ _ w1156 _] -> w1063
                            tunnel: [_ _ w1143 _] -> w1062
                            tunnel: [_ _ w1145 _] -> w1061
                            tunnel: w1060 -> [_ w1082 _ _]
                            tunnel: w1059 -> [_ w1081 _ _]
                            frame #0 {
                              n617 = local read "N samples/decay min"() -> (w1079:i32)
                              n618 = Initialize Array(i16 0 ("élément"), w1077, w1079) -> (w1080:i16[][])
                            }
                            frame #1 {
                              n619 = for {
                                tunnel: w1088 -> [w1100] mode=indexing
                                shift-right: [w1097] -> w1084
                                shift-left: w1085 -> [w1098]
                                shift-right: [w1103] -> w1083
                                shift-left: 0 -> [w1102]
                                tunnel: w1087 -> [w1101]
                                tunnel: w1082 -> [w1096]
                                tunnel: w1081 -> [w1089] mode=indexing
                                i -> [w1099]
                                n620 = Equal?(x=w1100, y=w1101) -> (x = y?=w1092:bool)
                                n621 = local read "BA"() -> (w1091:bool)
                                n622 = Equal?(x=w1089, y=1) -> (x = y?=w1095:bool)
                                n623 = And(x=w1095, y=w1092) -> (x .and. y?=w1093:bool)
                                n624 = Select(t=w1093, s=w1091, f=w1092) -> (s? t:f=w1090:bool)
                                n625 = case shown="True" w1090 {
                                tunnel: [w1105 w1117] -> w1103
                                tunnel: w1102 -> [w1105 w1110]
                                tunnel: w1099 -> [_ w1114]
                                tunnel: w1096 -> [_ w1113]
                                tunnel: w1098 -> [w1104 w1109]
                                tunnel: [w1104 w1108] -> w1097
                                frame False {
                                }
                                frame True {
                                n626 = local read "N samples/decay min"() -> (w1115:i32)
                                n627 = Array Subset(array=w1113, index (row)=w1114, length (row)=1 ("longueur")) -> (w1116:i16[][])  [unwired: 2 in]
                                n628 = Reshape Array(w1116, w1115) -> (w1111:i16[])
                                n629 = Increment(x=w1110) -> (x+1=w1117:i32)
                                n630 = Build Array(w1111) -> (w1107:i16[][])
                                n631 = Replace Array Subset(array=w1109, new element=w1107, index (row)=w1110, index (col)=0 ("indice")) -> (w1108:i16[][])
                                }
                                }
                              }
                            }
                            frame #2 {
                              w1124 = 7.11341 ("y")
                              w1126 = 90.47064 ("y")
                              # "y0"
                              # "A1"
                              # "A2"
                              # "t1"
                              # "t2"
                              n632 = local read "Skip samples"() -> (w1168:i32)
                              n633 = local read "Last samples"() -> (w1167:i32)
                              n634 = local read "N samples/decay min"() -> (w1169:i32)
                              n635 = call "IMAQ ArrayToImage"("Image Pixels (I16)"=w1171, "Image"=w1170) -> ("Image Out"=w1166:T3)  [unwired: 4 in, 5 out]
                              n636 = Multiply(x=w1164, y=1000.0) -> (x*y=w1163:dbl)
                              n637 = call "AnalyDecayPhosphoAndSystem.vi"("Scan rate (Hz)"=w1163, "Raw Data Image"=w1166, "N pulses"=w1142, "Skip samples"=w1168, "Last samples"=w1167, "N samples/decay"=w1169) -> ("mean and fit"=w1146:dbl[][], "Tau (us)"=w1162:dbl, "Standard error Tau (us)"=w1161:dbl)  [unwired: 7 out]
                              n638 = Array Subset(array=w1146, index (row)=2 ("indice"), length (row)=1 ("longueur")) -> (w1150:dbl[][])  [unwired: 2 in]
                              n639 = Build Array(w1161) -> (w1121:dbl[])
                              n640 = Build Array(w1162) -> (w1120:dbl[])
                              n641 = Array Size(array=w1146) -> (size(s)=w1152:i32[])
                              n642 = Array Subset(array=w1146, index (row)=0 ("indice"), length (row)=1 ("longueur")) -> (w1153:dbl[][])  [unwired: 2 in]
                              n643 = Index Array(array=w1152, index=1 ("indice")) -> (element=w1147:i32)
                              n644 = Reshape Array(w1150, w1147) -> (w1144:dbl[])
                              n645 = Divide(x=w1120, y=w1124) -> (x/y=w1141:dbl[])
                              n646 = Divide(x=w1120, y=w1126) -> (x/y=w1140:dbl[])
                              n647 = Negate(x=w1141) -> (-x=w1132:dbl[])
                              n648 = Negate(x=w1140) -> (-x=w1133:dbl[])
                              n649 = Exponential(1:w1133) -> (0:w1139:dbl[])
                              n650 = Exponential(1:w1132) -> (0:w1138:dbl[])
                              n651 = Multiply(x=w1139, y=161.37547) -> (x*y=w1127:dbl[])
                              n652 = Divide(x=w1127, y=w1126) -> (x/y=w1131:dbl[])
                              n653 = Negate(x=w1131) -> (-x=w1128:dbl[])
                              n654 = Multiply(x=w1138, y=546.54987) -> (x*y=w1125:dbl[])
                              n655 = Divide(x=w1125, y=w1124) -> (x/y=w1130:dbl[])
                              n656 = Negate(x=w1130) -> (-x=w1129:dbl[])
                              n657 = Add(x=w1128, y=w1129) -> (x+y=w1123:dbl[])
                              n658 = Multiply(x=w1123, y=w1121) -> (x*y=w1122:dbl[])
                              n659 = Add(x=w1127, y=w1125) -> (x+y=w1135:dbl[])
                              n660 = Add(x=w1135, y=-96.55396) -> (x+y=w1118:dbl[])
                              n661 = Absolute Value(x=w1122) -> (abs(x)=w1119:dbl[])
                              n662 = Index Array(array=w1119, index=0 ("indice")) -> (element=w1158:dbl)
                              n663 = Index Array(array=w1118, index=0 ("indice")) -> (element=w1157:dbl)
                              n664 = Reshape Array(w1153, w1147) -> (w1143:dbl[])
                              n665 = Subtract(x=w1144, y=w1143) -> (x-y=w1145:dbl[])
                            }
                            frame #3 {
                              n666 = Increment(x=w1175) -> (x+1=w1172:i32)
                              n667 = call "waitbar.vi"("Number at end of work"=w1174, "Current Number"=w1172) -> ("Break Computation"=w1173:bool)
                            }
                          }
                        }
                        "Error Tau around RBCs" <- w1039
                        "Error PO2 around RBCs" <- w1038
                        "Average / RBCs" <- w1037
                        "Std / RBCs" <- w1036
                        n668 = local write "Analyse EAT"(FALSE ("Analyse EAT")) -> ()
                        n669 = local read "N samples/decay min"() -> (w1035:i32)
                        n670 = Divide(x=w1035, y=w998) -> (x/y=w1034:dbl)
                        n671 = Multiply(x=w1033, y=w1034) -> (x*y=w1000:dbl[])
                        n672 = Index Array(array=w1000, index=0) -> (element=w1013:dbl)
                        n673 = Subtract(x=w1011, y=w1013) -> (x-y=w996:dbl)
                        n674 = Subtract(x=20.0, y=w1011) -> (x-y=w997:dbl)
                        n675 = Divide(x=w999, y=1000) -> (x/y=w995:dbl)
                        n676 = Divide(x=w997, y=w995) -> (x/y=w1009:dbl)
                        n677 = Divide(x=w996, y=w995) -> (x/y=w1012:dbl)
                        n678 = To Long Integer(number=w1012) -> (32bit integer=w1002:i32)
                        n679 = To Long Integer(number=w1009) -> (32bit integer=w1003:i32)
                        n680 = Array Subset(array=w1000, index=w1002, length=w1003) -> (w993:dbl[])
                        n681 = Array Subset(array=w1008, index=w1002, length=w1003) -> (w994:dbl[])
                        n682 = Array Subset(array=w1007, index=w1002, length=w1003) -> (w1006:dbl[])
                        n683 = Array Subset(array=w1004, index=w1002, length=w1003) -> (w1005:i32[])
                        n684 = Bundle "Bundle"(w993, w994) -> (→"Tau / RBCs":cluster{dbl[], dbl[]})  [unwired: 1 out]
                        n685 = local write "Decays"(w1005) -> ()
                        n686 = Bundle "Bundle"(w993, w1006) -> (→"PO2 / RBCs":cluster{dbl[], dbl[]})  [unwired: 1 out]
                        n687 = Bundle "Bundle"(w993, w1005) -> (→"Decays / RBCs":cluster{dbl[], i32[]})  [unwired: 1 out]
                      }
                    }
                  }
                }
              }
            }
          }
          frame #4 {
            # "Display image"
            n688 = case shown="True" "Analyse Average" {
              frame False {
              }
              frame True {
                n689 = local write "Not NewlyAcquired"(FALSE ("Not NewlyAcquired")) -> ()
                n690 = local write "Analyse Average"(FALSE ("RE-Analyse")) -> ()
                n691 = local write "Analyse"(TRUE ("Analyse")) -> ()
              }
            }
            n692 = local read "Total time per point (s)"() -> (w1176:dbl)
            n693 = local read "N pulses per point"() -> (w1179:i32)
            n694 = local read "Repeat each point"() -> (w1180:i64)
            n695 = Not Equal?(x="Display raw Data", y="Display raw changed") -> (x != y?=w1177:bool)
            n696 = Multiply(x=w1179, y=w1180) -> (x*y=w1178:i64)
            n697 = case shown="True" w1177 {
              tunnel: "Display raw Data" -> [_ w1186]
              tunnel: w1176 -> [_ w1185]
              tunnel: w1178 -> [_ w1184]
              frame False {
              }
              frame True {
                n698 = local write "Display raw changed"(w1186) -> ()
                n699 = case shown="True" w1186 {
                  tunnel: w1185 -> [_ w1192]
                  tunnel: w1184 -> [_ w1191]
                  frame False {
                    n700 = local read "Local error"() -> (w1189:errorcluster)
                    n701 = call "IMAQ WindShow"("error in (no error)"=w1189, "Hide/Show (Show)"=FALSE, "Window Number (0...15)"=13) -> ("error out"=w1188:errorcluster)  [unwired: 2 in, 3 out]
                    n702 = local write "Local error"(w1188) -> ()
                  }
                  frame True {
                    n703 = stacked-sequence {
                      tunnel: w1192 -> [_ w1216 _]
                      tunnel: w1191 -> [_ w1214 _]
                      frame #0 {
                        w1210 = 1 ("X Step Size")
                        # "Display restriction"
                        n704 = local read "N pulses per point"() -> (w1200:i32)
                        n705 = local read "Repeat each point"() -> (w1199:i64)
                        n706 = local read "Decays Max"() -> (w1195:i32)
                        n707 = local read "N samples/decay min"() -> (w1206:i32)
                        n708 = local read "Skip samples"() -> (w1208:i32)
                        n709 = Multiply(x=w1200, y=w1199) -> (x*y=w1197:i64)
                        n710 = Less?(x=w1197, y=w1195) -> (x < y?=w1198:bool)
                        n711 = local read "Channel Analysed"() -> (w1203:u16)
                        n712 = local read "Raw Data Image"() -> (w1201:T3[][])
                        n713 = local read "Point Number"() -> (w1204:i32)
                        n714 = Select(t=w1197, s=w1198, f=w1195) -> (s? t:f=w1196:i64)
                        n715 = Build Array(w1208, 1 ("élément"), w1206, w1196) -> (w1209:i64[])
                        n716 = local read "Raw Data Display"() -> (w1194:T3)
                        n717 = local read "Local error"() -> (w1205:errorcluster)
                        n718 = Decrement(x=w1209) -> (x-1=w1202:i64[])
                        n719 = Index Array(array=w1201, index (row)=w1203, index (col)=w1204) -> (element=w1193:T3)
                        n720 = call "IMAQ Extract"("Y Step Size"=w1210, "Optional Rectangle"=w1202, "error in (no error)"=w1205, "X Step Size"=w1210, "Image Dst"=w1194, "Image Src"=w1193) -> ()  [unwired: 6 out]
                      }
                      frame #1 {
                        n721 = Divide(x=w1216, y=0.1) -> (x/y=w1213:dbl)
                        n722 = local read "Raw Data Display"() -> (w1211:T3)
                        n723 = Divide(x=w1214, y=w1216) -> (x/y=w1217:dbl)
                        n724 = Round Toward -Infinity(1:w1213) -> (0:w1215:dbl)
                        n725 = To Long Integer(number=w1215) -> (32bit integer=w1212:i32)
                        n726 = for {
                          N: w1212 -> [_]
                          tunnel: w1211 -> [w1231]
                          tunnel: w1217 -> [w1220]
                          i -> [w1226]
                          n727 = Increment(x=w1226) -> (x+1=w1222:i32)
                          n728 = Multiply(x=0.1, y=w1222) -> (x*y=w1221:dbl)
                          n729 = Multiply(x=w1220, y=w1221) -> (x*y=w1219:dbl)
                          n730 = To Long Integer(number=w1219) -> (32bit integer=w1224:i32)
                          n731 = Bundle("Y"=100, w1224) -> (w1228:cluster{"Y":i32, i32})  [unwired: 1 out]
                          n732 = Format Into String(format string="%.2f" ("chaîne de format"), w1221) -> (resulting string=w1227:string)  [unwired: 2 in, 1 out]
                          n733 = call "IMAQ Overlay Text"("Text Color (black)"=u32 16711680, "String"=w1227, "Origin"=w1228, "Image"=w1231) -> ()  [unwired: 4 in, 4 out]
                        }
                      }
                      frame #2 {
                        w1235 = 13 ("Window Number (0...15)")
                        n734 = local read "Raw Data Display"() -> (w1234:T3)
                        n735 = call "LUT_selector.vi"("LUT1"="LUT") -> ("Palette1"=w1232:cluster{u8, u8, u8}[])  [unwired: 1 in, 1 out]
                        n736 = call "Imaq WindDraw"("Window Number (0...15)"=w1235, "Color Palette"=w1232, "Title"="Phosphorescence Raw Data", "Image"=w1234) -> ("error out"=w1240:errorcluster)  [unwired: 2 in, 5 out]
                        n737 = call "IMAQ WindSize"("error in (no error)"=w1240, "Scrollbars? (N)"=TRUE, "Window Number"=w1235) -> ("error out"=w1237:errorcluster)  [unwired: 2 in, 3 out]
                        n738 = call "IMAQ WindShow"("error in (no error)"=w1237, "Bring To Front? (N)"=TRUE, "Hide/Show (Show)"=TRUE, "Window Number (0...15)"=w1235) -> ("error out"=w1238:errorcluster)  [unwired: 1 in, 3 out]
                        n739 = local write "Local error"(w1238) -> ()
                      }
                    }
                  }
                }
              }
            }
          }
        }
        n740 = Wait (ms)(milliseconds to wait=1 ("y")) -> ()  [unwired: 1 out]
        n741 = local read "ForceEnd"() -> (w148:bool)
        n742 = Or(x="stop", y=w148) -> (x .or. y?=w149:bool)
      }
    }
    frame #2 {
      # "EAT"
      # "Decay"
      # "RBC flow"
      # "Time Lapsed"
      # "Averaged"
      # "Clear display"
      # "Erase Images"
      # "Close Pictures windows"
      # "Free memory"
      n743 = local read "Average fit"() -> (w1285:dbl[][])
      n744 = local write "Acquisition Time"(timestamp(-9593251200 s since 1904-01-01) ("Acquisition Time")) -> ()
      n745 = local write "Working file"(path "") -> ()
      n746 = call "IMAQ WindClose"("Window Number (0...15)"=13) -> ("error out"=w1316:errorcluster)  [unwired: 3 in, 2 out]
      n747 = local read "DataValues"() -> (w1256:T1)
      n748 = Array Size(array=w1285) -> (size(s)=w1280:i32[])
      "size(s) 2" <- w1280
      n749 = call "IMAQ WindClose"("Window Number (0...15)"=14, "error in (no error)"=w1316) -> ()  [unwired: 2 in, 3 out]
      n750 = Array Size(array=w1256) -> (size(s)=w1253:i32)
      n751 = for {
        N: w1253 -> [_]
        tunnel: [w1319] -> w1252 mode=indexing
        w1321 = 0.0 ("Standard error Tau (us)")
        w1322 = 0.0 ("element 2")
        w1324 = 0.0 ("element")
        w1323 = 0.0 ("Tau (us)")
        w1325 = 0.0 ("Area (au)")
        w1320 = 0.0 ("amplitude")
        n752 = local write "amplitude"(w1320) -> ()
        n753 = local write "Area (au)"(w1325) -> ()
        n754 = local write "Tau (us)"(w1323) -> ()
        n755 = local write "element"(w1324) -> ()
        n756 = local write "element 2"(w1322) -> ()
        n757 = local write "Standard error Tau (us)"(w1321) -> ()
        n758 = Bundle("amplitude"=w1320, "Area (au)"=w1325, "Tau (us)"=w1323, "element"=w1324, "element 2"=w1322, "Standard error Tau (us)"=w1321) -> (w1319:T14)  [unwired: 1 in]
      }
      n759 = Index Array(array=w1280, index=0) -> (element=w1282:i32)
      n760 = Index Array(array=w1280, index=1) -> (element=w1281:i32)
      n761 = local write "to time (s)"(0.0 ("to time (s)")) -> ()
      n762 = Initialize Array(0.0, w1282, w1281) -> (w1279:dbl[][])
      n763 = local read "Image To Save"() -> (w1314:T3)
      n764 = local read "Image 8bit"() -> (w1313:T3)
      n765 = local write "Average fit"(w1279) -> ()
      n766 = local write "Mean Flow"(0.0 ("Mean Flow")) -> ()
      n767 = local write "Mean Hematocrit"(0.0 ("Mean Hematocrit")) -> ()
      n768 = call "IMAQ Dispose"("Image"=w1313) -> ()  [unwired: 2 in, 4 out]
      n769 = call "IMAQ Dispose"("Image"=w1314) -> ()  [unwired: 2 in, 4 out]
      n770 = local write "DataValues"(w1252) -> ()
      n771 = local read "Raw Data Display"() -> (w1312:T3)
      n772 = local read "Decays"() -> (w1306:i32[])
      n773 = local read "TmpDataPicture"() -> (w1310:T3)
      n774 = local read "RBC anal Checked"() -> (w1278:dbl[][])
      n775 = Array Size(array=w1306) -> (size(s)=w1297:i32)
      n776 = call "IMAQ Dispose"("Image"=w1310) -> ()  [unwired: 2 in, 4 out]
      n777 = call "IMAQ Dispose"("Image"=w1312) -> ()  [unwired: 2 in, 4 out]
      n778 = Array Size(array=w1278) -> (size(s)=w1271:i32[])
      "size(s) 3" <- w1271
      n779 = Initialize Array(0, w1297) -> (w1300:i32[])
      n780 = Initialize Array(0.0, w1297) -> (w1299:dbl[])
      n781 = Initialize Array(0.0, w1297) -> (w1296:dbl[])
      n782 = Initialize Array(0.0, w1297) -> (w1295:dbl[])
      n783 = local write "Tau"(w1295) -> ()
      n784 = local read "Raw Data Image"() -> (w1315:T3[][])
      n785 = local write "Time"(w1296) -> ()
      n786 = local write "Decays"(w1300) -> ()
      n787 = local write "Po2"(w1299) -> ()
      n788 = Index Array(array=w1271, index=0) -> (element=w1274:i32)
      n789 = Index Array(array=w1271, index=1) -> (element=w1273:i32)
      n790 = local read "Local Raw Data"() -> (w1311:T3)
      n791 = Initialize Array(0.0, w1274, w1273) -> (w1272:dbl[][])
      n792 = Bundle "Bundle"(w1296, w1295) -> (w1301:cluster{dbl[], dbl[]})  [unwired: 1 out]
      n793 = Bundle "Bundle"(w1296, w1299) -> (w1302:cluster{dbl[], dbl[]})  [unwired: 1 out]
      n794 = Bundle "Bundle"(w1296, w1300) -> (w1303:cluster{dbl[], i32[]})  [unwired: 1 out]
      n795 = local write "RBC anal Checked"(w1272) -> ()
      n796 = for {
        tunnel: w1315 -> [w1326] mode=indexing
        n797 = for {
          tunnel: w1326 -> [w1327] mode=indexing
          n798 = call "IMAQ Dispose"("Image"=w1327) -> ()  [unwired: 2 in, 4 out]
        }
      }
      n799 = local write "PO2 / RBCs"(w1302) -> ()
      n800 = local write "Tau / RBCs"(w1301) -> ()
      n801 = local write "Decays / RBCs"(w1303) -> ()
      n802 = call "IMAQ Dispose"("Image"=w1311) -> ()  [unwired: 2 in, 4 out]
      n803 = local write "Number of decays 1"(0 ("Number pulse 1")) -> ()
      n804 = local write "pO2 (1)"(0.0 ("PO2 1")) -> ()
      n805 = local write "Std pO2 (1)"(0.0 ("Std PO2 1")) -> ()
      n806 = local write "Std Tau 1"(0.0 ("Std Tau 1")) -> ()
      n807 = local write "Tau 1 (us)"(0.0 ("Tau 1 (us)")) -> ()
      n808 = local write "Amplitude 1"(0.0 ("Amplitude 1")) -> ()
      n809 = local write "From time (ms) 1"(-1.0 ("From time (ms) 1")) -> ()
      n810 = local write "To time (ms) 1"(1.0 ("To time (ms) 1")) -> ()
      n811 = local read "Average fit 1/2"() -> (w1294:dbl[][])
      n812 = local write "Max"(20.0 ("Max")) -> ()
      n813 = local write "Min"(-3.0 ("Min")) -> ()
      n814 = local write "localTimeData"(timestamp[][] [] ("localTimeData")) -> ()
      n815 = Array Size(array=w1294) -> (size(s)=w1288:i32[])
      "size(s)" <- w1288
      n816 = local write "Number of decays 2"(0 ("Number pulse 2")) -> ()
      n817 = local write "pO2 (2)"(0.0 ("PO2 2")) -> ()
      n818 = local write "Tau 2 (us)"(0.0 ("Tau 2 (us)")) -> ()
      n819 = local write "Std pO2 (2)"(0.0 ("Std PO2 2")) -> ()
      n820 = local write "Std Tau 2"(0.0 ("Std Tau 2")) -> ()
      n821 = local write "Amplitude 2"(0.0 ("Amplitude 2")) -> ()
      n822 = local write "From time (ms) 2"(8.0 ("From time (ms) 2")) -> ()
      n823 = local write "To time (ms) 2"(12.0 ("To time (ms) 2")) -> ()
      n824 = Index Array(array=w1288, index=0) -> (element=w1290:i32)
      n825 = Index Array(array=w1288, index=1) -> (element=w1287:i32)
      n826 = Initialize Array(0.0, w1290, w1287) -> (w1292:dbl[][])
      n827 = local write "Average fit 1/2"(w1292) -> ()
    }
  }
